vi "Results_file_Plotter.vi"() -> ()   [LabVIEW 2013]
uses:
  Anemometry/Anemometry Sub Vis/Data_plotting_vis/Plot_Slice.ctl
  Anemometry/Anemometry Sub Vis/Data_plotting_vis/Plotter_Mode.ctl
  Anemometry/Anemometry Sub Vis/Data_plotting_vis/Data_File_Type.ctl
  Anemometry/Anemometry Sub Vis/File/Setup_Filetype.ctl
  Anemometry/Anemometry Sub Vis/Controls/Global_mode.ctl
  Anemometry/Anemometry Sub Vis/Data_plotting_vis/Results_plotter_Global.vi
  Anemometry/Anemometry Sub Vis/Globals/Trav_pos_global.vi
  Instance           1 28Saved   Results_file_Plotter .vi
  Anemometry/Anemometry Sub Vis/Globals/Constants_global.vi
panel:
  out "Selected Row?":bool
  out "Edit Raw DF?":bool
  in  "Tab Control":T1(tab)=enum."Save "
  in  "Template":path
  in  "Empty":bool
  in  "Result files to read":path[](array[path])
  in  "Add results file":bool
  in  "File Types to Read":T2
  in  "Vector Plot?":bool
  in  "Ordinate Name":string
  out "2nd Add label":string
  out "First Add label":string
  in  "Additional X Values":dbl[](array[numeric]) format="%.2f"
  in  "Additional Y Values":dbl[](array[numeric]) format="%.2f"
  in  "Show Results Space Analysis":bool
  in  "Show Plot Space Analysis":bool
  in  "Multi Ordinate":i32[](listbox)
  in  "Multi Ordinate?":bool
  in  "Ordinate":u16(ring) items=["Date", "Profile", "Multi Run Start Time", "Multi Run Row Type", "Multi Run Row Number", "Point Time", "Time Stamp", "Measuring Instrument Type", "Comments", "Run Messages", "X_{HF} (mm)", "Y_{HF} (mm)", "Z_{HF} (mm)", "X_{5HP} (mm)", "Y_{5HP} (mm)", "Z_{5HP} (mm)", "Repeat", "U_{HF}/U_{ref}", "TI_{HF} %", "\\sigma_{HF}/U_{ref}", "L(U) Est (m)", "U_{5HP}/U_{ref}", "U_{HF}/U_{5HP}", "TI_{U(5HP)} %", "Vmag_{5HP}/U_{ref}", "V_{5HP}/U_{5HP}", "W_{5HP}/U_{5HP}", "U_{ref}", "U_{HF}", "Tau(HF)", "uhf^2", "uhf^3/(uhf^2)^1.5", "(uhf^4/(uhf^2)^2) -3", "HW (Uhf) Standard Error in Mean", "HW (Uhf) Standard Error in Variance", "HW Cal", "Vmag_{5HP}", "U_{5HP}", "V_{5HP}", "W_{5HP}", "Vmag_SD", "U_SD", "V_SD", "W_SD", "Tau(5HP1) (nose)", "Tau(5HP2) (bottom)", "Tau(5HP3) (top)", "Tau(5HP4) (side)", "Tau(5HP5) (side)", "GoodFraction", "5HP Mode", "5HP ReturnType", "Reference Temperature Used for Corrections", "Atmos Pressure Used for Corrections", "Av Analogue Sampling Rate", "No of Analogue Samples", "No Of Measurement Blocks", "Flow Measurement Time", "X (URef) (mm)", "Y (URef) (mm)", "Z (URef) (mm)", "Original Results Filename", "Current Data Filename", "Current Data File 1st Folder level", "Current Data File 2nd Folder level", "Current Data File 3rd Folder level", "Current Data File 4th Folder level", "Current File Number", "Raw Data Filename"]
  in  "Intensity Plot?":bool
  in  "Absisca":u16(ring) items=["Date", "Profile", "Multi Run Start Time", "Multi Run Row Type", "Multi Run Row Number", "Point Time", "Time Stamp", "Measuring Instrument Type", "Comments", "Run Messages", "X_{HF} (mm)", "Y_{HF} (mm)", "Z_{HF} (mm)", "X_{5HP} (mm)", "Y_{5HP} (mm)", "Z_{5HP} (mm)", "Repeat", "U_{HF}/U_{ref}", "TI_{HF} %", "\\sigma_{HF}/U_{ref}", "L(U) Est (m)", "U_{5HP}/U_{ref}", "U_{HF}/U_{5HP}", "TI_{U(5HP)} %", "Vmag_{5HP}/U_{ref}", "V_{5HP}/U_{5HP}", "W_{5HP}/U_{5HP}", "U_{ref}", "U_{HF}", "Tau(HF)", "uhf^2", "uhf^3/(uhf^2)^1.5", "(uhf^4/(uhf^2)^2) -3", "HW (Uhf) Standard Error in Mean", "HW (Uhf) Standard Error in Variance", "HW Cal", "Vmag_{5HP}", "U_{5HP}", "V_{5HP}", "W_{5HP}", "Vmag_SD", "U_SD", "V_SD", "W_SD", "Tau(5HP1) (nose)", "Tau(5HP2) (bottom)", "Tau(5HP3) (top)", "Tau(5HP4) (side)", "Tau(5HP5) (side)", "GoodFraction", "5HP Mode", "5HP ReturnType", "Reference Temperature Used for Corrections", "Atmos Pressure Used for Corrections", "Av Analogue Sampling Rate", "No of Analogue Samples", "No Of Measurement Blocks", "Flow Measurement Time", "X (URef) (mm)", "Y (URef) (mm)", "Z (URef) (mm)", "Original Results Filename", "Current Data Filename", "Current Data File 1st Folder level", "Current Data File 2nd Folder level", "Current Data File 3rd Folder level", "Current Data File 4th Folder level", "Current File Number", "Raw Data Filename"]
  in  "Job Directory":path
  in  "Save Averaged rows":bool
  in  "Save Surface Fit":bool
  in  "Output Filename":path
  in  "Save Data in Rows":bool
  in  "Save Plot data":bool
  in  "Header":string
  in  "Process Point":bool
  in  "Kill Point":bool
  out "Table":string[][](table)
  in  "Post Process Plotted Data":bool
  in  "...using routine":string
  in  "Calculate new metadata":bool
  in  "Add /Edit metadata":bool
  in  "Delete Plotted data from file":bool
  in  "Save Setup":bool
  in  "Load Setup":bool
  in  "stop":bool
  out "Current":string="Graph Scales"
  in  "Single Series":i32[](listbox)=[0]
  in  "Edit Template File":bool
  in  "color and symbol":bool
  out "nRows":i32
  in  "Filter Bins 2":i32[](listbox)=[0]
  in  "Filter 6":u16(ring)
  in  "Filter 5":u16(ring)
  in  "Filter 4":u16(ring) items=["Show All (160)", "BLANK (160)", "CalCheck (0)", "Zeroes (0)", "NOT BLANK (0)", "NOT CalCheck (160)", "NOT Zeroes (160)"]
  in  "Filter 3":u16(ring) items=["Show All (352)", "B2 (80)", "BLANK (0)", "C1 (160)", "C2 (112)", "NOT B2 (272)", "NOT BLANK (352)", "NOT C1 (192)", "NOT C2 (240)"]
  in  "Filter Array":u16[](array[ring])=[0, 0, 0, 0, 0, 0] items=["Don't Filter", "Date", "Profile", "Multi Run Start Time", "Multi Run Row Type", "Multi Run Row Number", "Point Time", "Time Stamp", "Measuring Instrument Type", "Comments", "Run Messages", "X_{HF} (mm)", "Y_{HF} (mm)", "Z_{HF} (mm)", "X_{5HP} (mm)", "Y_{5HP} (mm)", "Z_{5HP} (mm)", "Repeat", "U_{HF}/U_{ref}", "TI_{HF} %", "\\sigma_{HF}/U_{ref}", "L(U) Est (m)", "U_{5HP}/U_{ref}", "U_{HF}/U_{5HP}", "TI_{U(5HP)} %", "Vmag_{5HP}/U_{ref}", "V_{5HP}/U_{5HP}", "W_{5HP}/U_{5HP}", "U_{ref}", "U_{HF}", "Tau(HF)", "uhf^2", "uhf^3/(uhf^2)^1.5", "(uhf^4/(uhf^2)^2) -3", "HW (Uhf) Standard Error in Mean", "HW (Uhf) Standard Error in Variance", "HW Cal", "Vmag_{5HP}", "U_{5HP}", "V_{5HP}", "W_{5HP}", "Vmag_SD", "U_SD", "V_SD", "W_SD", "Tau(5HP1) (nose)", "Tau(5HP2) (bottom)", "Tau(5HP3) (top)", "Tau(5HP4) (side)", "Tau(5HP5) (side)", "GoodFraction", "5HP Mode", "5HP ReturnType", "Reference Temperature Used for Corrections", "Atmos Pressure Used for Corrections", "Av Analogue Sampling Rate", "No of Analogue Samples", "No Of Measurement Blocks", "Flow Measurement Time", "X (URef) (mm)", "Y (URef) (mm)", "Z (URef) (mm)", "Original Results Filename", "Current Data Filename", "Current Data File 1st Folder level", "Current Data File 2nd Folder level", "Current Data File 3rd Folder level", "Current Data File 4th Folder level", "Current File Number", "Raw Data Filename"]
  in  "Filter Bins 1":i32[](listbox)=[0]
  in  "Create picture Vi Name":string caption="Picture VI:"
  in  "Save Plot as jpg":bool
  in  "Reload Files":bool
  out "Selected Row":i32
  out "Warning!":string
  out "XY Plot":cluster{dbl[], dbl[]}[](graph)
  out "Edit Raw Data Header Info":bool
  out "Raw DF in Orig Pos?":bool
  out "Intensity Graph":dbl[][](graph)
  in  "Bkgnd Value":dbl
  in  "Update":bool
  in  "Plot Resolution":bool
  in  "Point Size":i32(slide)=1 scale=0.0..10.0
  in  "No of Contours":i32=20
  in  "Slice mode":T3
  in  "Z Ch Name":u16(ring) items=["Date", "Profile", "Multi Run Start Time", "Multi Run Row Type", "Multi Run Row Number", "Point Time", "Time Stamp", "Measuring Instrument Type", "Comments", "Run Messages", "X_{HF} (mm)", "Y_{HF} (mm)", "Z_{HF} (mm)", "X_{5HP} (mm)", "Y_{5HP} (mm)", "Z_{5HP} (mm)", "Repeat", "U_{HF}/U_{ref}", "TI_{HF} %", "\\sigma_{HF}/U_{ref}", "L(U) Est (m)", "U_{5HP}/U_{ref}", "U_{HF}/U_{5HP}", "TI_{U(5HP)} %", "Vmag_{5HP}/U_{ref}", "V_{5HP}/U_{5HP}", "W_{5HP}/U_{5HP}", "U_{ref}", "U_{HF}", "Tau(HF)", "uhf^2", "uhf^3/(uhf^2)^1.5", "(uhf^4/(uhf^2)^2) -3", "HW (Uhf) Standard Error in Mean", "HW (Uhf) Standard Error in Variance", "HW Cal", "Vmag_{5HP}", "U_{5HP}", "V_{5HP}", "W_{5HP}", "Vmag_SD", "U_SD", "V_SD", "W_SD", "Tau(5HP1) (nose)", "Tau(5HP2) (bottom)", "Tau(5HP3) (top)", "Tau(5HP4) (side)", "Tau(5HP5) (side)", "GoodFraction", "5HP Mode", "5HP ReturnType", "Reference Temperature Used for Corrections", "Atmos Pressure Used for Corrections", "Av Analogue Sampling Rate", "No of Analogue Samples", "No Of Measurement Blocks", "Flow Measurement Time", "X (URef) (mm)", "Y (URef) (mm)", "Z (URef) (mm)", "Original Results Filename", "Current Data Filename", "Current Data File 1st Folder level", "Current Data File 2nd Folder level", "Current Data File 3rd Folder level", "Current Data File 4th Folder level", "Current File Number", "Raw Data Filename"]
  in  "Y Ch Name":u16(ring) items=["Date", "Profile", "Multi Run Start Time", "Multi Run Row Type", "Multi Run Row Number", "Point Time", "Time Stamp", "Measuring Instrument Type", "Comments", "Run Messages", "X_{HF} (mm)", "Y_{HF} (mm)", "Z_{HF} (mm)", "X_{5HP} (mm)", "Y_{5HP} (mm)", "Z_{5HP} (mm)", "Repeat", "U_{HF}/U_{ref}", "TI_{HF} %", "\\sigma_{HF}/U_{ref}", "L(U) Est (m)", "U_{5HP}/U_{ref}", "U_{HF}/U_{5HP}", "TI_{U(5HP)} %", "Vmag_{5HP}/U_{ref}", "V_{5HP}/U_{5HP}", "W_{5HP}/U_{5HP}", "U_{ref}", "U_{HF}", "Tau(HF)", "uhf^2", "uhf^3/(uhf^2)^1.5", "(uhf^4/(uhf^2)^2) -3", "HW (Uhf) Standard Error in Mean", "HW (Uhf) Standard Error in Variance", "HW Cal", "Vmag_{5HP}", "U_{5HP}", "V_{5HP}", "W_{5HP}", "Vmag_SD", "U_SD", "V_SD", "W_SD", "Tau(5HP1) (nose)", "Tau(5HP2) (bottom)", "Tau(5HP3) (top)", "Tau(5HP4) (side)", "Tau(5HP5) (side)", "GoodFraction", "5HP Mode", "5HP ReturnType", "Reference Temperature Used for Corrections", "Atmos Pressure Used for Corrections", "Av Analogue Sampling Rate", "No of Analogue Samples", "No Of Measurement Blocks", "Flow Measurement Time", "X (URef) (mm)", "Y (URef) (mm)", "Z (URef) (mm)", "Original Results Filename", "Current Data Filename", "Current Data File 1st Folder level", "Current Data File 2nd Folder level", "Current Data File 3rd Folder level", "Current Data File 4th Folder level", "Current File Number", "Raw Data Filename"]
  in  "X Ch Name":u16(ring) items=["Date", "Profile", "Multi Run Start Time", "Multi Run Row Type", "Multi Run Row Number", "Point Time", "Time Stamp", "Measuring Instrument Type", "Comments", "Run Messages", "X_{HF} (mm)", "Y_{HF} (mm)", "Z_{HF} (mm)", "X_{5HP} (mm)", "Y_{5HP} (mm)", "Z_{5HP} (mm)", "Repeat", "U_{HF}/U_{ref}", "TI_{HF} %", "\\sigma_{HF}/U_{ref}", "L(U) Est (m)", "U_{5HP}/U_{ref}", "U_{HF}/U_{5HP}", "TI_{U(5HP)} %", "Vmag_{5HP}/U_{ref}", "V_{5HP}/U_{5HP}", "W_{5HP}/U_{5HP}", "U_{ref}", "U_{HF}", "Tau(HF)", "uhf^2", "uhf^3/(uhf^2)^1.5", "(uhf^4/(uhf^2)^2) -3", "HW (Uhf) Standard Error in Mean", "HW (Uhf) Standard Error in Variance", "HW Cal", "Vmag_{5HP}", "U_{5HP}", "V_{5HP}", "W_{5HP}", "Vmag_SD", "U_SD", "V_SD", "W_SD", "Tau(5HP1) (nose)", "Tau(5HP2) (bottom)", "Tau(5HP3) (top)", "Tau(5HP4) (side)", "Tau(5HP5) (side)", "GoodFraction", "5HP Mode", "5HP ReturnType", "Reference Temperature Used for Corrections", "Atmos Pressure Used for Corrections", "Av Analogue Sampling Rate", "No of Analogue Samples", "No Of Measurement Blocks", "Flow Measurement Time", "X (URef) (mm)", "Y (URef) (mm)", "Z (URef) (mm)", "Original Results Filename", "Current Data Filename", "Current Data File 1st Folder level", "Current Data File 2nd Folder level", "Current Data File 3rd Folder level", "Current Data File 4th Folder level", "Current File Number", "Raw Data Filename"]
  in  "Resolution":dbl=1.0 min=0.0 format="%.4f"
  out "Surface Area":dbl format="%^_6g"
  out "Surface Integral":dbl format="%^_6g"
  out "Surface Average":dbl format="%^#.6g"
  out "Uadvec":dbl
  in  "Full_Res_Results_Folder":path
  out "Last used Template":path
  out "Cursor index":i32
  out "Choosen Path":path
  in  "VI Refnum Calculation":refnum<vi>
  out "Filetype":string[](array[string])
  out "Mode":T4
  out "Plotted rows only?":bool
  in  "type specifier VI Refnum (for type only) 2":refnum<vi>
  in  "type specifier VI Refnum (for type only)":refnum<vi>
  out "Accept Array":bool[][](array[boolean])
  out "Previous slice mode":T3
  out "Slice mode Change?":bool
  out "Non-Blank Rows":bool[](array[boolean])
  out "File Index":i32
  out "Tolerances":dbl[](array[numeric]) format="%.2f"
  in  "Results files choosen":path[](array[path])
  in  "Transpose":bool
  out "Plotted Series":bool[][](array[boolean])
  in  "Results file":path
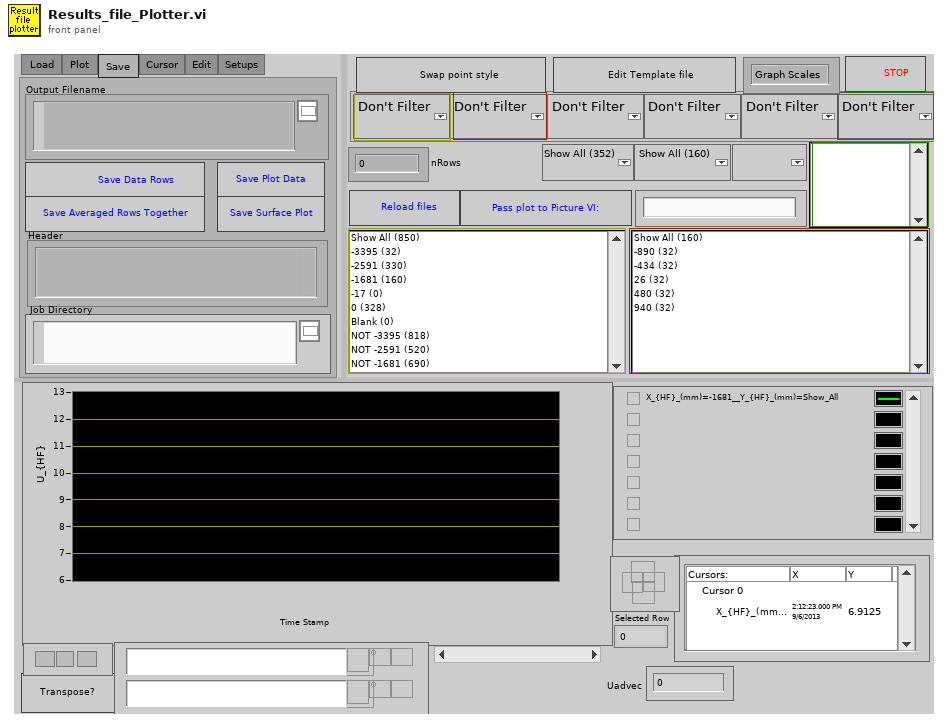
[diagram p1: front panel]
types:
  T1 = enum32{"Load ", "Plot ", "Save ", "Cursor", "Edit", "Setups"}
  T2 = typedef "Data_File_Type.ctl" = enum16{"Read All File Types", "Results Files Only", "Raw Data Files Only", "Calibration Files Only", "Gas Desk Files Only", "Old Results Files Only", "Tabulated Data Files Only"}
  T3 = typedef "Plot_Slice.ctl" = enum16{"XY Slice (Plan)", "YX Slice (Plan)", "YZ Slice (Cross)", "ZY Slice (Cross)", "XZ Slice (Side)", "ZX Slice (Side)"}
  T4 = typedef "Plotter_Mode.ctl" = enum16{"Save file", "Delete unwanted rows", "Edit Values with constants", "Edit values per row", "Edit Raw Data file header", "Post Process Plotted Rows"}
  T5 = typedef "Setup_Filetype.ctl" = enum16{"Measurement Setups", "Calibration Setups", "General", "Results File Plotter Setups", "Speed Calib Tweaks"}
  T6 = enum16{"Zero or one", "One", "Zero or more", "One or more"}
  T7 = typedef "Global_mode.ctl" = enum16{"Read Global", "Load Global From File", "Write Global to File"}
  T8 = enum16{"Edit Existing Template File", "Create New Template File"}
  T9 = enum16{"Show only data summary", "Show data summary", "No data summary"}
  T10 = typedef "All_Setup.ctl" = cluster{"Result files to read":path[], "Template":path, "Transpose":bool, "Additional X Values":dbl[], "Additional Y Values":dbl[], "Ordinate":u16, "Absisca":u16, "Filter Array":u16[], "color and symbol":bool, "Output Filename":path, "Jpg Vi Name":string, "Intensity Plot?":bool, "Multi Ordinate?":bool, "Filter Bins 1":i32[], "Filter Bins 2":i32[], "Multi Ordinate":i32[]}
  T11 = enum16{"Left Button", "Center Button", "Right Button", "Window Close"}
  T12 = enum32{"existing file", "new file", "new or existing file", "existing dir", "new dir", "new or existing dir", "existing file (use LLBs)", "new file (use LLBs)", "new or existing file (use LLBs)", "new or existing file or directory (use LLBs)"}
  T13 = cluster{"Plot Color":u32, "Plot Interpolation":u8, "Point Style":u8, "Line Style":u8, "Fill/Pt. Color":u32, "Line Width":u8, "Bar Plot Style":u8, "Fill To":i16}[]
  T14 = typedef "Group_Binning.ctl" = cluster{"Index":i32, "Tolerance":dbl, "Precision":string}
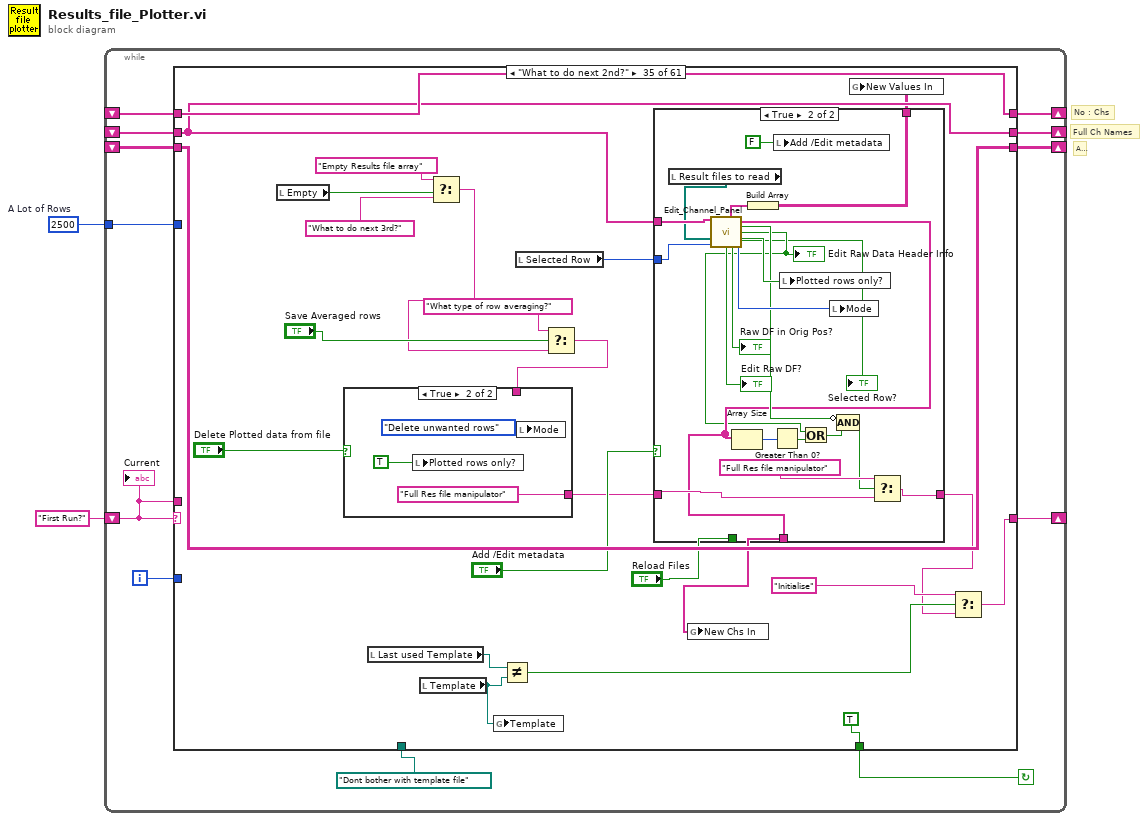
[diagram p0: block diagram]
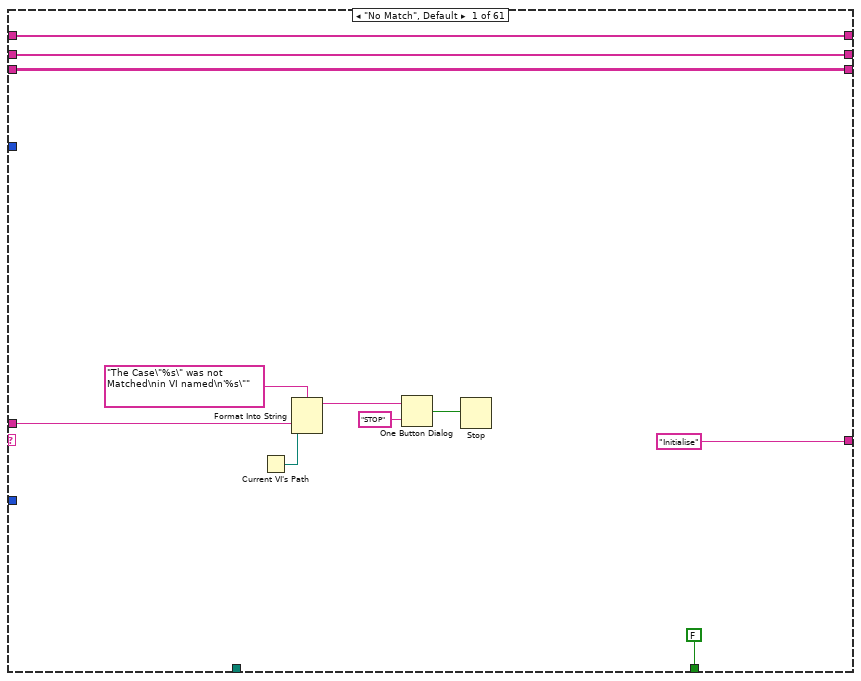
[diagram p2: hidden frame]
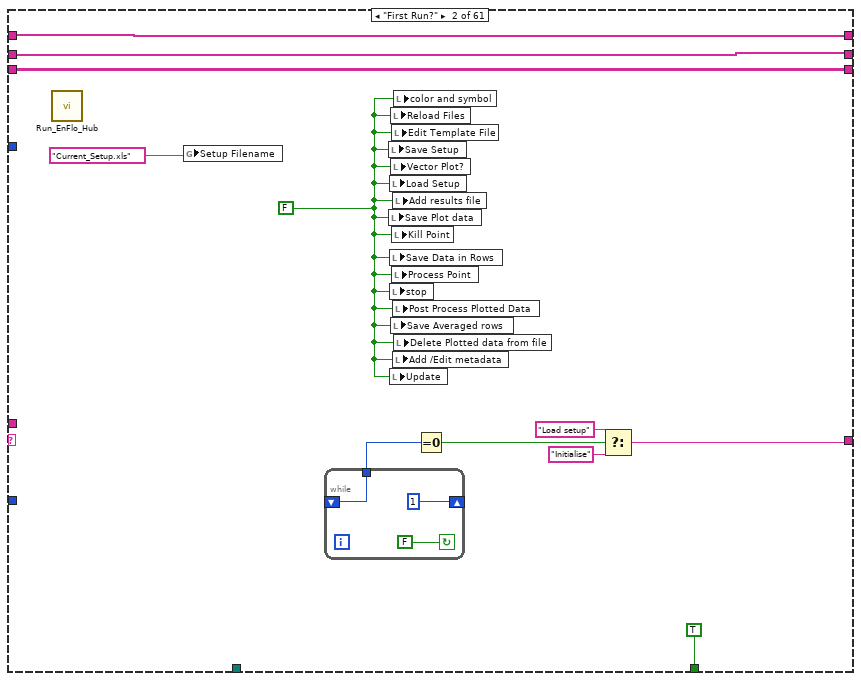
[diagram p3: hidden frame]
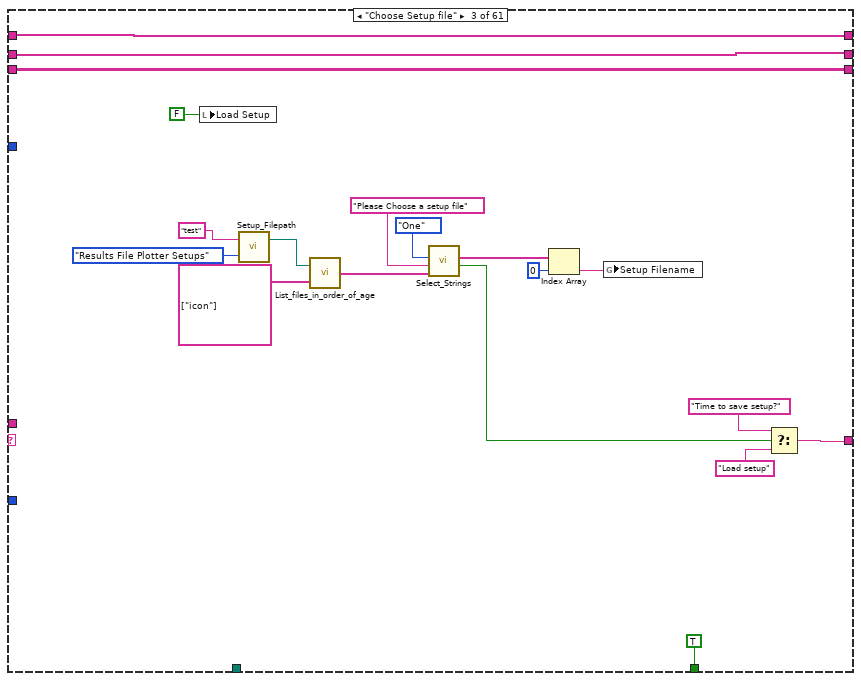
[diagram p4: hidden frame]
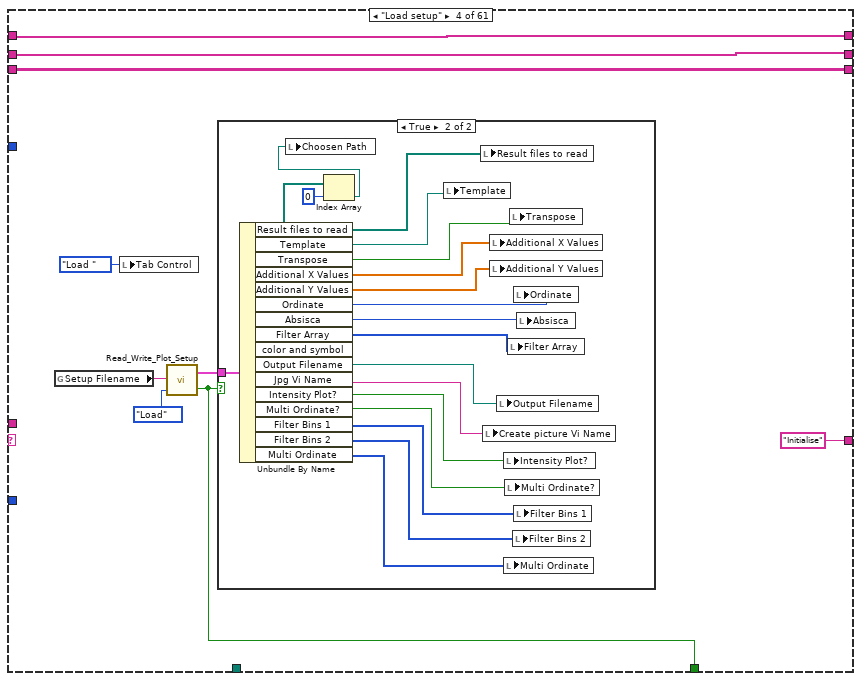
[diagram p5: hidden frame]
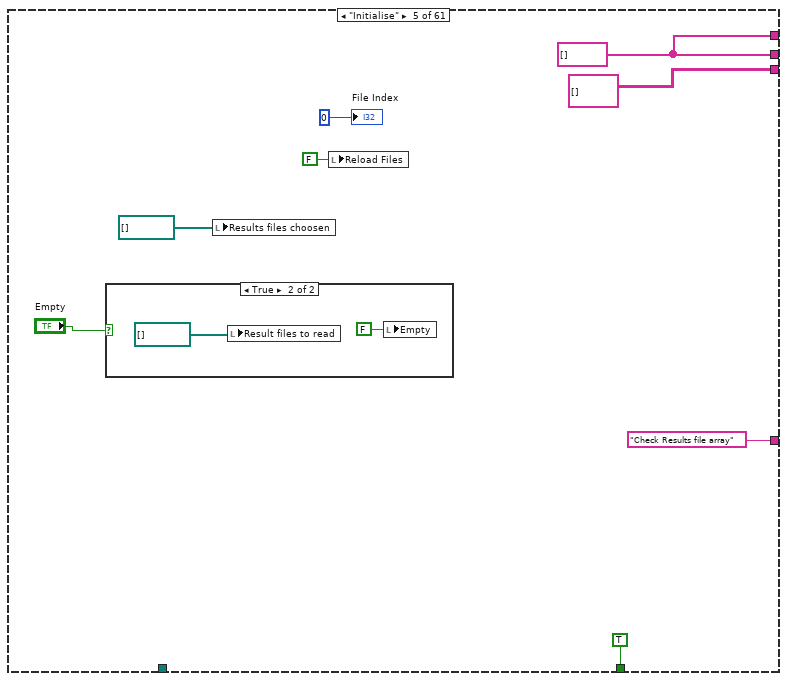
[diagram p7: hidden frame]
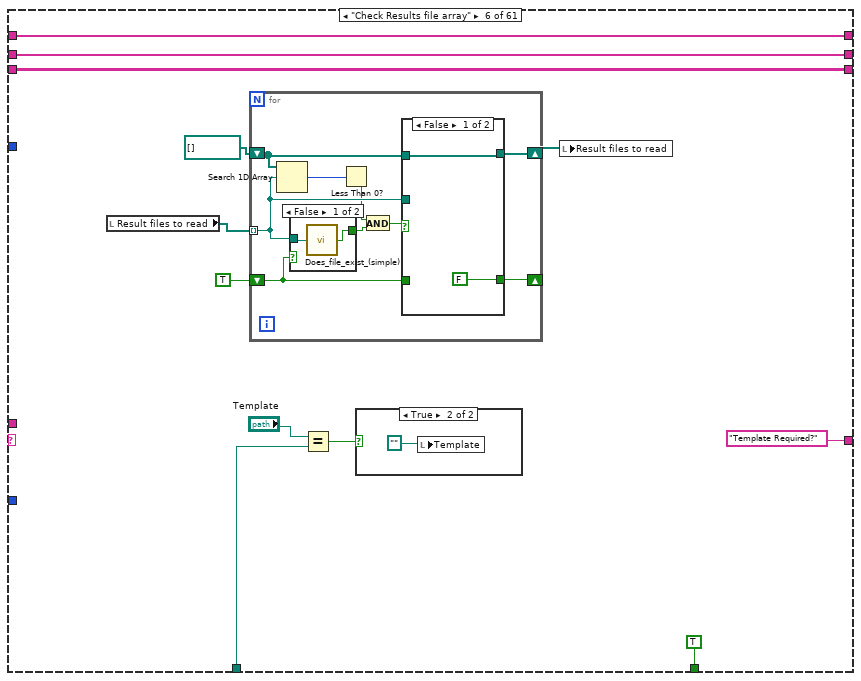
[diagram p9: hidden frame]
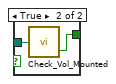
[diagram p11: hidden frame]
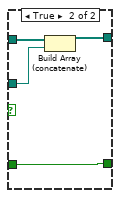
[diagram p12: hidden frame]
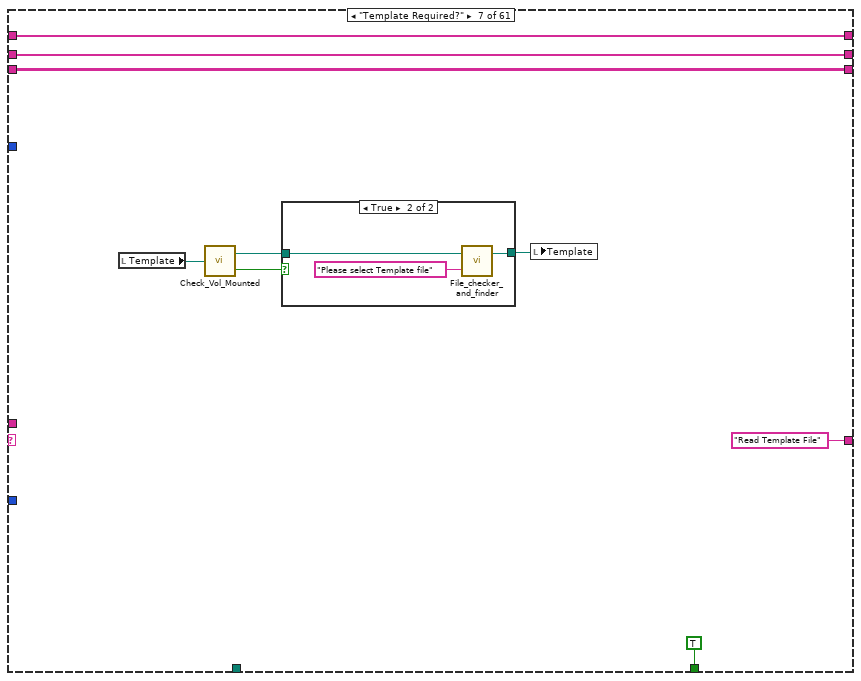
[diagram p13: hidden frame]
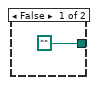
[diagram p14: hidden frame]
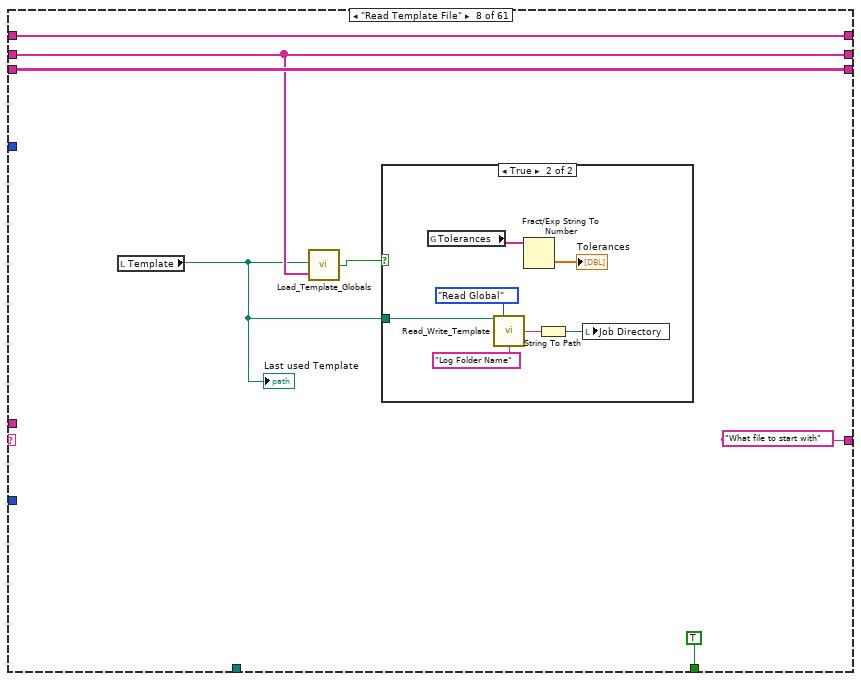
[diagram p15: hidden frame]
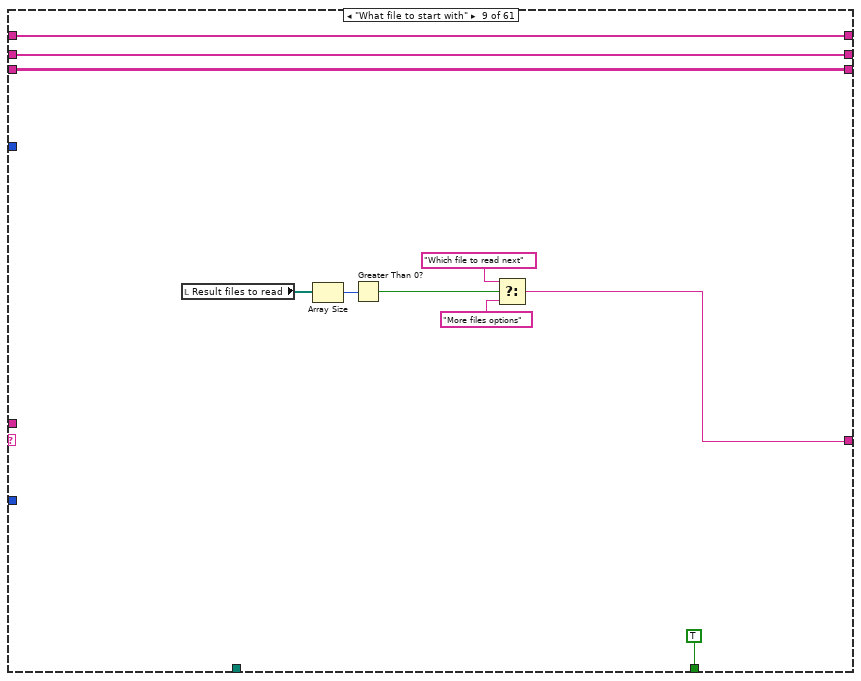
[diagram p17: hidden frame]
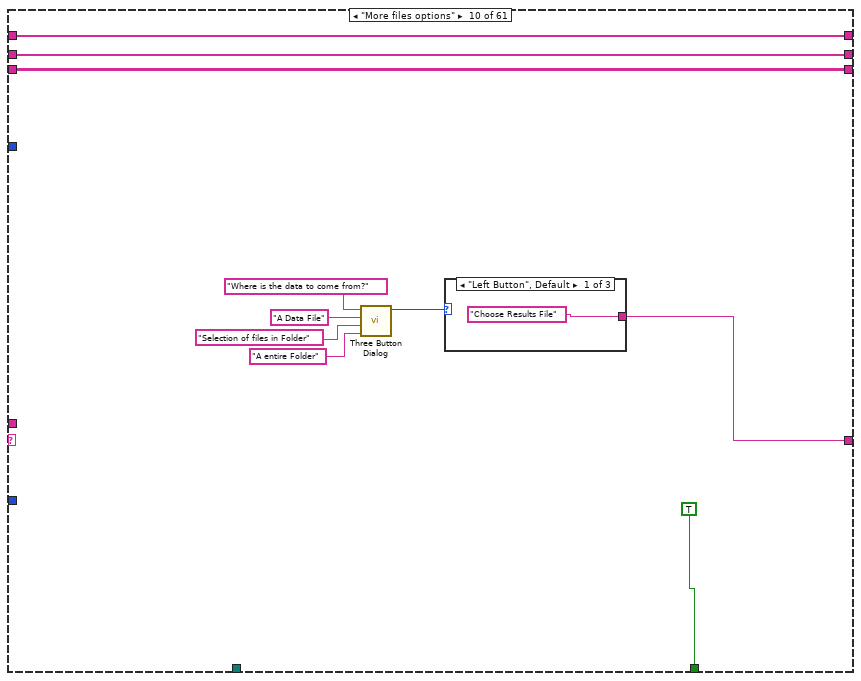
[diagram p18: hidden frame]
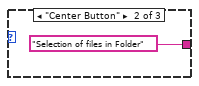
[diagram p19: hidden frame]
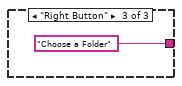
[diagram p20: hidden frame]
diagram:
  w1 = 2500  # A Lot of Rows
  # "No : Chs"
  # "Full Ch Names"
  # "All"
  n1 = while {
    shift-left: _ -> [w7]
    shift-right: [w8] -> _
    shift-left: "First Run?" -> [w11]
    shift-right: [w4] -> _
    shift-left: _ -> [w9]
    shift-right: [w14] -> _
    shift-left: _ -> [w12]
    shift-right: [w5] -> _
    tunnel: w1 -> [w3]
    i -> [w6]
    stop <- w13 continue-if-true
    n2 = case shown="\"What to do next 2nd?\"" w11 {
      tunnel: w9 -> [w25 w35 w57 w65 _ w106 w134 w143 w164 w174 w186 w200 w231 w258 w281 w403 w425 w451 w476 w502 w556 w570 w607 w909 w978 w1033 w1058 w1077 w1163 w1214 w1244 w1533 w1549 w1570 w1600 w1666 w1699 w1774 w1797 w1812 w1876 w1928 w1954 w2163 w2175 w2201 w2327 w2471 w2505 w2520 w2545 w2572 w2615 w2633 w2676 w2779 w2813 w3177 w3192 w3228 w3236]
      tunnel: [w25 w35 w57 w65 w91 w106 w134 w143 w164 w174 w186 w200 w231 w258 w279 w403 w425 w451 w476 w502 w556 w570 w607 w909 w978 w1033 w1058 w1077 w1163 w1214 w1242 w1533 w1549 w1570 w1600 w1666 w1699 w1774 w1797 w1812 w1876 w1928 w1952 w2163 w2175 w2199 w2320 w2471 w2505 w2520 w2545 w2572 w2615 w2633 w2676 w2779 w2813 w3177 w3192 w3228 w3236] -> w14
      tunnel: ["Initialise" w28 w52 "Initialise" ("t") "Check Results file array" ("t") "Template Required?" "Read Template File" "What file to start with" w155 w170 "Which file to read next" "Which file to read next" "Which file to read next" w254 w276 w394 "What is present?" "Ordinate Selector Type" w473 "Which rows are Non-Blank?" w549 "Create Selectors" w596 "Re Plot Data?" w973 "Prepare Filter2 strings" "Plot Data" w1074 "Add Axis names" "Analyse Plot Space" w1245 "What to do next?" "What to do next?" ("t") w1556 w1593 w1644 w1697 w1768 w1793 w1811 w1875 "Initialise" w1955 w2154 "Create Selectors" w2202 w2328 w2469 w2503 w2510 w2529 "Save XY plot as jpg" "Create Selectors" w2630 w2679 w2763 w2818 "Save Setup" ("t") "Initialise" ("t") w3197 "Time to save setup?"] -> w4
      tunnel: [FALSE TRUE TRUE w61 TRUE TRUE TRUE TRUE TRUE TRUE TRUE TRUE TRUE w249 w283 TRUE TRUE TRUE TRUE TRUE TRUE TRUE TRUE TRUE TRUE TRUE TRUE w1075 TRUE TRUE w1246 TRUE TRUE ("OK?") TRUE TRUE ("OK?") TRUE ("OK?") w1695 TRUE TRUE w1810 w1874 TRUE w1956 TRUE ("OK?") TRUE ("OK?") w2203 w2329 TRUE TRUE TRUE TRUE TRUE TRUE TRUE TRUE TRUE TRUE TRUE TRUE w3206 TRUE ("OK?")] -> w13
      tunnel: w12 -> [w24 w34 w56 w64 _ w105 w133 w145 w163 w173 w185 w199 w230 w257 w282 w399 w424 w452 w477 w503 w555 w568 w602 w911 w967 w1035 w1060 w1076 w1165 w1216 w1243 w1532 w1548 w1569 w1611 w1665 w1698 w1773 w1796 w1809 w1873 w1927 w1953 w2162 w2172 w2200 w2326 w2472 w2504 w2519 w2549 w2575 w2614 w2632 w2675 w2778 w2812 w3176 w3191 w3227 w3235]
      tunnel: w11 -> [w16 _ _ _ _ _ _ _ _ _ _ _ _ _ _ _ _ _ _ _ _ _ _ _ _ _ _ _ _ _ _ _ _ _ _ _ _ _ _ _ _ _ _ _ _ _ _ _ _ _ _ _ _ _ _ _ _ _ _ _ _]
      tunnel: path "Dont bother with template file" ("Template File") -> [_ _ _ _ _ w99 _ _ _ _ _ _ _ _ _ _ _ _ _ _ _ _ _ _ _ _ _ _ _ _ _ _ _ _ _ _ _ _ _ _ _ _ _ _ _ _ _ _ _ _ _ _ _ _ _ _ _ w3174 w3186 _ _]
      tunnel: [w15 w33 w55 w66 w91 w104 w132 w144 w161 w171 w183 w197 w228 w256 w278 w387 w423 w453 w475 w501 w547 w569 w600 w908 w969 w1026 w1053 w1073 w1157 w1209 w1238 w1529 w1550 w1568 w1601 w1667 w1700 w1772 w1795 w1808 w1872 w1926 w1946 w2164 w2180 w2190 w2323 w2481 w2506 w2521 w2546 w2573 w2616 w2634 w2680 w2780 w2819 w3178 w3193 w3229 w3237] -> w8
      tunnel: w7 -> [w15 w33 w55 w66 _ w104 w132 w144 w161 w171 w183 w197 w228 w256 w277 w387 w423 w453 w475 w501 w547 w569 w600 w908 w969 w1026 w1053 w1073 w1157 w1209 w1237 w1529 w1550 w1568 w1601 w1667 w1700 w1772 w1795 w1808 w1872 w1926 w1945 w2164 w2180 w2194 w2322 w2481 w2506 w2521 w2546 w2573 w2616 w2634 w2680 w2780 w2819 w3178 w3193 w3229 w3237]
      tunnel: w6 -> [_ _ _ _ _ _ _ _ _ _ _ _ _ _ _ _ _ _ _ _ _ _ _ _ _ _ _ _ _ _ _ _ _ _ _ _ w1696 _ _ _ _ _ _ _ _ _ _ _ _ _ _ _ _ _ _ _ _ _ _ _ _]
      tunnel: [w24 w34 w56 w64 string[][] [] w105 w133 w145 w163 w173 w185 w199 w230 w257 w280 w399 w424 w452 w477 w503 w555 w568 w602 w911 w967 w1035 w1060 w1076 w1165 w1216 w1241 w1532 w1548 w1569 w1611 w1665 w1698 w1773 w1796 w1809 w1873 w1927 w1951 w2162 w2172 w2198 w2319 w2472 w2504 w2519 w2549 w2575 w2614 w2632 w2675 w2778 w2812 w3176 w3191 w3227 w3235] -> w5
      tunnel: w3 -> [_ _ _ _ _ _ _ _ _ _ _ _ _ _ _ _ _ _ _ _ _ _ _ _ _ _ _ _ _ _ _ _ _ _ _ _ _ _ w1791 _ w1871 _ _ _ _ _ _ _ _ _ _ _ _ w2629 w2673 _ w2810 _ _ _ _]
      frame "No Match", Default {
        n3 = Current VI's Path() -> (path=w17:path)
        n4 = Format Into String(format string="The Case\"%s\" was not Matched\nin VI named\n'%s\"" ("Format String"), w16, w17) -> (resulting string=w20:string)  [unwired: 2 in, 1 out]
        n5 = One Button Dialog(message=w20, button name ("OK")="STOP") -> (true=w18:bool)
        n6 = Stop(stop? (T)=w18) -> ()
      }
      frame "First Run?" {
        w26 = FALSE ("Save Plot data")
        n7 = call "Run_EnFlo_Hub.vi"() -> ()  [unwired: 8 out]
        n8 = global write "Results_plotter_Global.vi" "Setup Filename"("Current_Setup.xls" ("Setup filename")) -> ()
        n9 = while {
          shift-right: [1] -> _
          shift-left: _ -> [w38]
          tunnel: [w38] -> w30
          stop <- FALSE continue-if-true
        }
        n10 = local write "Save Setup"(w26) -> ()
        n11 = local write "Save Plot data"(w26) -> ()
        n12 = local write "Load Setup"(w26) -> ()
        n13 = local write "Save Data in Rows"(w26) -> ()
        n14 = local write "stop"(w26) -> ()
        n15 = local write "Update"(w26) -> ()
        n16 = local write "Reload Files"(w26) -> ()
        n17 = local write "Vector Plot?"(w26) -> ()
        n18 = local write "Save Averaged rows"(w26) -> ()
        n19 = local write "Edit Template File"(w26) -> ()
        n20 = local write "Kill Point"(w26) -> ()
        n21 = local write "Process Point"(w26) -> ()
        n22 = local write "Add results file"(w26) -> ()
        n23 = local write "Post Process Plotted Data"(w26) -> ()
        n24 = local write "Add /Edit metadata"(w26) -> ()
        n25 = local write "color and symbol"(w26) -> ()
        n26 = local write "Delete Plotted data from file"(w26) -> ()
        n27 = Equal To 0?(x=w30) -> (x = 0?=w29:bool)
        n28 = Select(t="Load setup", s=w29, f="Initialise") -> (s? t:f=w28:string)
      }
      frame "Choose Setup file" {
        n29 = local write "Load Setup"(FALSE ("Save Setup")) -> ()
        n30 = call "Setup_Filepath.vi"("Setup File Type"=Setup_Filetype."Results File Plotter Setups", "Filename in"="test") -> ("Directory"=w40:path)  [unwired: 1 out]
        n31 = call "List_files_in_order_of_age.vi"("Files to Hide"=string[] ["icon"], "Folder"=w40) -> ("file names"=w51:string[])
        n32 = call "Select_Strings.vi"("Available Ch names"=w51, "Message"="Please Choose a setup file", "Selector mode"=T6."One") -> ("Cancel"=w45:bool, "Selected Channel Names"=w48:string[])  [unwired: 1 in, 3 out]
        n33 = Index Array(array=w48, index=0) -> (element=w46:string)
        n34 = global write "Results_plotter_Global.vi" "Setup Filename"(w46) -> ()
        n35 = Select(t="Time to save setup?", s=w45, f="Load setup") -> (s? t:f=w52:string)
      }
      frame "Load setup" {
        n36 = global read "Results_plotter_Global.vi" "Setup Filename"() -> (w60:string)
        n37 = local write "Tab Control"(T1."Load " ("Tab Control")) -> ()
        n38 = call "Read_Write_Plot_Setup.vi"("Mode"=enum16{"Load", "Save"}."Load", "Setup filename"=w60) -> ("OK?"=w61:bool, "Cluster 2"=w62:T10)  [unwired: 1 in]
        n39 = case shown="True" w61 {
          tunnel: w62 -> [_ w85]
          frame False {
          }
          frame True {
            n40 = Unbundle By Name(w85) -> ("Result files to read"=w70:path[], "Template"=w68:path, "Transpose"=w75:bool, "Additional X Values"=w76:dbl[], "Additional Y Values"=w77:dbl[], "Ordinate"=w78:u16, "Absisca"=w79:u16, "Filter Array"=w80:u16[], "Output Filename"=w81:path, "Jpg Vi Name"=w82:string, "Intensity Plot?"=w83:bool, "Multi Ordinate?"=w84:bool, "Filter Bins 1"=w74:i32[], "Filter Bins 2"=w73:i32[], "Multi Ordinate"=w72:i32[])  [unwired: 1 out]
            n41 = Index Array(array=w70, index=0) -> (element=w69:path)
            n42 = local write "Choosen Path"(w69) -> ()
            n43 = local write "Template"(w68) -> ()
            n44 = local write "Result files to read"(w70) -> ()
            n45 = local write "Create picture Vi Name"(w82) -> ()
            n46 = local write "Additional X Values"(w76) -> ()
            n47 = local write "Additional Y Values"(w77) -> ()
            n48 = local write "Output Filename"(w81) -> ()
            n49 = local write "Intensity Plot?"(w83) -> ()
            n50 = local write "Multi Ordinate"(w72) -> ()
            n51 = local write "Multi Ordinate?"(w84) -> ()
            n52 = local write "Filter Array"(w80) -> ()
            n53 = local write "Transpose"(w75) -> ()
            n54 = local write "Filter Bins 2"(w73) -> ()
            n55 = local write "Ordinate"(w78) -> ()
            n56 = local write "Filter Bins 1"(w74) -> ()
            n57 = local write "Absisca"(w79) -> ()
          }
        }
      }
      frame "Initialise" {
        w91 = string[] [] ("Channel names")
        n58 = case shown="True" "Empty" {
          frame False {
          }
          frame True {
            n59 = local write "Result files to read"(path[] [] ("Result files to read")) -> ()
            n60 = local write "Empty"(FALSE ("Empty")) -> ()
          }
        }
        n61 = local write "Results files choosen"(path[] [] ("Results file choosen")) -> ()
        n62 = local write "Reload Files"(FALSE ("Reload Files")) -> ()
        "File Index" <- 0
      }
      frame "Check Results file array" {
        n63 = local read "Result files to read"() -> (w103:path[])
        n64 = for {
          shift-right: [w117] -> w101
          shift-left: path[] [] -> [w116]
          tunnel: w103 -> [w115] mode=indexing
          shift-right: [w110] -> _
          shift-left: TRUE -> [w109]
          n65 = Search 1D Array(1D array=w116, element=w115) -> (index of element=w114:i32)  [unwired: 1 out]
          n66 = case shown="False" w109 {
            tunnel: w115 -> [w119 w121]
            tunnel: [w118 w120] -> w112
            frame False {
              n67 = call "Does_file_exist_(simple).vi"("Pathname"=w119) -> ("exists?"=w118:bool)
            }
            frame True {
              n68 = call "Check_Vol_Mounted.vi"("Filename"=w121) -> ("exists?"=w120:bool)  [unwired: 1 out]
            }
          }
          n69 = Less Than 0?(x=w114) -> (x < 0?=w111:bool)
          n70 = And(x=w111, y=w112) -> (x .and. y?=w113:bool)
          n71 = case shown="False" w113 {
            tunnel: w116 -> [w123 w127]
            tunnel: w115 -> [_ w126]
            tunnel: [w123 w125] -> w117
            tunnel: [FALSE w124] -> w110
            tunnel: w109 -> [_ w124]
            frame False {
            }
            frame True {
              n72 = Build Array (concatenate)(w127, w126) -> (w125:path[])
            }
          }
        }
        n73 = Equal?(x="Template", y=w99) -> (x = y?=w98:bool)
        n74 = case shown="True" w98 {
          frame False {
          }
          frame True {
            n75 = local write "Template"(path "") -> ()
          }
        }
        n76 = local write "Result files to read"(w101) -> ()
      }
      frame "Template Required?" {
        n77 = local read "Template"() -> (w131:path)
        n78 = call "Check_Vol_Mounted.vi"("Filename"=w131) -> ("Filename Out"=w130:path, "exists?"=w129:bool)
        n79 = case shown="True" w129 {
          tunnel: w130 -> [_ w139]
          tunnel: [path "" w138] -> w128
          frame False {
          }
          frame True {
            n80 = call "File_checker_and_finder.vi"("Promp if not found"="Please select Template file", "Filename In"=w139) -> ("Filename Out"=w138:path)  [unwired: 1 out]
          }
        }
        n81 = local write "Template"(w128) -> ()
      }
      frame "Read Template File" {
        n82 = local read "Template"() -> (w141:path)
        "Last used Template" <- w141
        n83 = call "Load_Template_Globals.vi"("Channel Names"=w143, "Template-read"=w141) -> ("Valid Template File?"=w142:bool)
        n84 = case shown="True" w142 {
          tunnel: w141 -> [_ w149]
          frame False {
          }
          frame True {
            n85 = global read "Results_plotter_Global.vi" "Tolerances"() -> (w153:string[])
            n86 = call "Read_Write_Template.vi"("Template File"=w149, "Mode"=Global_mode."Read Global", "Data type"="Log Folder Name" ("Variable name")) -> ("Single Value Out"=w151:string)  [unwired: 5 in, 7 out]
            n87 = Fract/Exp String To Number(string=w153) -> (number=→"Tolerances":dbl[])  [unwired: 4 out]
            n88 = String To Path(string=w151) -> (path=w148:path)
            n89 = local write "Job Directory"(w148) -> ()
          }
        }
      }
      frame "What file to start with" {
        n90 = local read "Result files to read"() -> (w160:path[])
        n91 = Array Size(array=w160) -> (size(s)=w159:i32)
        n92 = Greater Than 0?(x=w159) -> (x > 0?=w156:bool)
        n93 = Select(t="Which file to read next", s=w156, f="More files options") -> (s? t:f=w155:string)
      }
      frame "More files options" {
        n94 = call <vilib>:"Three Button Dialog.vi"("Right Button Text (\"Cancel\")"="A entire Folder" ("F button name (\"Cancel\")"), "Center Button Text (\"No\")"="Selection of files in Folder" ("T button name (\"OK\")"), "Left Button Text (\"Yes\")"="A Data File" ("T button name (\"OK\")"), "message"="Where is the data to come from?") -> ("Which Button?"=w169:T11)  [unwired: 1 in, 6 out]
        n95 = case shown="\"Left Button\", Default" w169 {
          tunnel: ["Choose Results File" "Selection of files in Folder" "Choose a Folder"] -> w170
          frame "Left Button", Default {
          }
          frame "Center Button" {
          }
          frame "Right Button" {
          }
        }
      }
      frame "Choose Results File" {
        (unwired) T12."existing file" ("select mode (2)")
        n96 = local read "Choosen Path"() -> (w178:path)
        n97 = File Dialog(7:"Please Choose a Results File" ("Promp if not found"), 11:w178) -> (1:w180:bool, 3:w179:path)  [unwired: 1 in, 6 out]
        "Choosen Path" <- w179
        n98 = case shown="False" w180 {
          tunnel: w179 -> [w187 _]
          frame False {
            n99 = local read "Result files to read"() -> (w188:path[])
            n100 = Build Array (concatenate)(w188, w187) -> (w189:path[])
            n101 = local write "Result files to read"(w189) -> ()
          }
          frame True {
          }
        }
      }
      frame "Choose a Folder" {
        n102 = local read "Choosen Path"() -> (w191:path)
        n103 = File Dialog(7:"Please Choose the folder that contains the Results files to be plotted" ("prompt"), 11:w191) -> (3:w190:path)  [unwired: 1 in, 7 out]
        n104 = local write "Choosen Path"(w190) -> ()
        n105 = call "Get_folder_and_filenames.vi"("file path (dialog if empty)"=w190) -> ("Files"=w192:path[])  [unwired: 1 out]
        n106 = for {
          shift-right: [w211] -> w193
          shift-left: "Result files to read" -> [w210]
          tunnel: w192 -> [w208] mode=indexing
          n107 = Search 1D Array(1D array=w210, element=w208) -> (index of element=w209:i32)  [unwired: 1 out]
          n108 = Strip Path(path=w208) -> (name=w207:string)  [unwired: 1 out]
          n109 = Less Than 0?(x=w209) -> (x < 0?=w206:bool)
          n110 = call "Add_filename_suffix.vi"("Filename"=w207) -> ("Original Suffix"=w204:string)  [unwired: 1 in, 3 out]
          n111 = call "Match_Pat_Case_In.vi"("String to match"=".jpg" ("x"), "String"=w204) -> ("offset past match"=w202:i32)  [unwired: 1 in, 3 out]
          n112 = Less Than 0?(x=w202) -> (x < 0?=w201:bool)
          n113 = And(x=w206, y=w201) -> (x .and. y?=w205:bool)
          n114 = case shown="True" w205 {
            tunnel: w210 -> [w212 w215]
            tunnel: w208 -> [_ w214]
            tunnel: [w212 w213] -> w211
            frame False {
            }
            frame True {
              n115 = Build Array (concatenate)(w215, w214) -> (w213:path[])
            }
          }
        }
        n116 = local write "Result files to read"(w193) -> ()
      }
      frame "Selection of files in Folder" {
        n117 = local read "Choosen Path"() -> (w217:path)
        n118 = local read "Result files to read"() -> (w220:path[])
        n119 = File Dialog(7:"Please Choose the folder that contains the Results files to be plotted" ("prompt"), 11:w217) -> (3:w216:path)  [unwired: 1 in, 7 out]
        n120 = call "Get_folder_and_filenames.vi"("file path (dialog if empty)"=w216) -> ("Files"=w222:path[])  [unwired: 1 out]
        n121 = local write "Choosen Path"(w216) -> ()
        n122 = for {
          tunnel: w222 -> [w245] mode=indexing
          tunnel: [w244] -> w225 mode=indexing
          n123 = Strip Path(path=w245) -> (name=w244:string)  [unwired: 1 out]
        }
        n124 = call "Select_Strings.vi"("Available Ch names"=w225, "Message"="Please select the desired data files", "Selector mode"=T6."Zero or more") -> ("Ch Indicies Choosen"=w223:i32[])  [unwired: 1 in, 4 out]
        n125 = for {
          tunnel: w223 -> [w243] mode=indexing
          tunnel: w222 -> [w242]
          tunnel: [w241] -> w218 mode=indexing
          n126 = Index Array(array=w242, index=w243) -> (element=w241:path)
        }
        n127 = for {
          shift-right: [w236] -> w219
          shift-left: w220 -> [w235]
          tunnel: w218 -> [w234] mode=indexing
          n128 = Search 1D Array(1D array=w235, element=w234) -> (index of element=w233:i32)  [unwired: 1 out]
          n129 = Less Than 0?(x=w233) -> (x < 0?=w232:bool)
          n130 = case shown="True" w232 {
            tunnel: w235 -> [w237 w240]
            tunnel: w234 -> [_ w239]
            tunnel: [w237 w238] -> w236
            frame False {
            }
            frame True {
              n131 = Build Array (concatenate)(w240, w239) -> (w238:path[])
            }
          }
        }
        n132 = local write "Result files to read"(w219) -> ()
      }
      frame "Which file to read next" {
        n133 = local read "Result files to read"() -> (w255:path[])
        n134 = local read "File Index"() -> (w252:i32)
        n135 = Array Size(array=w255) -> (size(s)=w253:i32)
        n136 = Equal?(x=w253, y=w252) -> (x = y?=w251:bool)
        n137 = case shown="False" w251 {
          tunnel: w255 -> [w261 _]
          tunnel: [w262 "Load Selectors"] -> w254
          tunnel: w252 -> [w260 w274]
          tunnel: [w259 w274] -> w247
          frame False {
            n138 = Index Array(array=w261, index=w260) -> (element=w263:path)
            n139 = Search 1D Array(1D array="Results files choosen", element=w263) -> (index of element=w265:i32)  [unwired: 1 out]
            n140 = call "Add_filename_suffix.vi"() -> ()  [unwired: 2 in, 4 out]
            n141 = case shown="-1" w265 {
              tunnel: "Results files choosen" -> [_ w273]
              tunnel: w263 -> [w269 w272]
              tunnel: ["Which file to read next" "Load Data"] -> w262
              frame 0, Default {
                n142 = Format Into String(format string="The filename\n \"%s\"\n has already been chosen" ("Format String"), w269) -> (resulting string=w267:string)  [unwired: 2 in, 1 out]
                n143 = One Button Dialog(message=w267) -> ()  [unwired: 2 out]
              }
              frame -1 {
                n144 = Build Array (concatenate)(w273, w272) -> (w271:path[])
                n145 = local write "Results files choosen"(w271) -> ()
              }
            }
            n146 = local write "Results file"(w263) -> ()
            n147 = Increment(x=w260) -> (x+1=w259:i32)
          }
          frame True {
          }
        }
        n148 = local read "stop"() -> (w250:bool)
        n149 = Decrement(x=w247) -> (x-1=w246:i32)
        n150 = Build Array(w246) -> (w248:i32[])
        n151 = Not(x=w250) -> (.not. x?=w249:bool)
        n152 = local write "File Index"(w247) -> ()
        n153 = property on="Result files to read" class="Arr (strict)"("Index Values"=w248) -> ()  [unwired: 2 in, 2 out]
      }
      frame "Load Data" {
        n154 = stacked-sequence {
          seq-local: [w288 _] -> [_ w348]
          seq-local: [w287 _] -> [_ w353]
          seq-local: [w286 _] -> [_ w352]
          seq-local: [w284 _] -> [_ w351]
          tunnel: [TRUE _] -> w283
          tunnel: w282 -> [w302 w354]
          tunnel: w281 -> [w301 _]
          tunnel: [w300 _] -> w280
          tunnel: [w299 _] -> w279
          tunnel: [w298 _] -> w278
          tunnel: w277 -> [w297 _]
          tunnel: ["Which file to read next" _] -> w276
          frame #0 {
            w291 = TRUE  # Add Extra Channels?
            n155 = local read "Template"() -> (w295:path)
            n156 = call "Read_Data_file.vi"("Results file"="Results file", "Add Extra Channels?"=w291, "Template File"=w295, "Desired File Types"="File Types to Read") -> ("Row numbers"=w286:i32[], "Template File Out"=w292:path, "Filetype"=w287:string, "Results file Out"=w288:path, "Ch names Out"=w293:string[], "Channel Values Out"=w289:string[][])  [unwired: 1 in, 9 out]
            n157 = local write "Template"(w292) -> ()
            n158 = Array Size(array=w293) -> (size(s)=w294:i32)
            n159 = Greater Than 0?(x=w294) -> (x > 0?=w284:bool)
            n160 = case shown="True" w284 {
              tunnel: w302 -> [w304 w318]
              tunnel: w301 -> [w306 w312]
              tunnel: w289 -> [_ w310]
              tunnel: [w304 w308] -> w300
              tunnel: [w306 w316] -> w299
              tunnel: [w305 w307] -> w298
              tunnel: w297 -> [w305 _]
              tunnel: w293 -> [_ w311]
              frame False {
              }
              frame True {
                n161 = for {
                  tunnel: w310 -> [w320] mode=indexing
                  tunnel: [w319] -> w309 mode=indexing
                  n162 = for {
                    tunnel: w320 -> [w322] mode=indexing
                    tunnel: [w321] -> w319 mode=indexing
                    n163 = call "Fast_string_Replace.vi"("Replace match with:"="[", "Input String"=w322, "regular expression"="(") -> ("Output String"=w323:string)  [unwired: 2 out]
                    n164 = call "Fast_string_Replace.vi"("Replace match with:"="]", "Input String"=w323, "regular expression"=")") -> ("Output String"=w321:string)  [unwired: 2 out]
                  }
                }
                n165 = call "Merge_channel_names.vi"("Preferred Channel array"=w312, "Channel array"=w311) -> ("Merged Channels"=w316:string[], "Preferred Channels Changed?"=w314:bool, "Channel Array Changed?"=w315:bool)
                n166 = for {
                  tunnel: w316 -> [w345] mode=indexing
                  tunnel: [w342] -> w307 mode=indexing
                  n167 = call "Fast_string_Replace.vi"("Replace match with:"=" ", "Input String"=w345, "regular expression"=":") -> ("Output String"=w341:string)  [unwired: 2 out]
                  n168 = call "Fast_string_Replace.vi"("Replace match with:"=" ", "Input String"=w341, "regular expression"="  ") -> ("Output String"=w340:string)  [unwired: 2 out]
                  n169 = call <vilib>:"Trim Whitespace.vi"("string"=w340) -> ("trimmed string"=w342:string)  [unwired: 1 in]
                }
                n170 = case shown="True" w314 {
                  tunnel: w318 -> [w333 w335]
                  tunnel: w312 -> [_ w337]
                  tunnel: [w333 w334] -> w313
                  tunnel: w316 -> [_ w336]
                  frame False {
                  }
                  frame True {
                    n171 = call "Merge_2D_values.vi"("Values In"=w335, "Present Channels"=w337, "Desired Channels"=w336) -> ("Values Out"=w334:string[][])
                  }
                }
                n172 = case shown="True" w315 {
                  tunnel: [w328 w332] -> w317
                  tunnel: w311 -> [_ w331]
                  tunnel: w309 -> [w328 w330]
                  tunnel: w316 -> [_ w329]
                  frame False {
                  }
                  frame True {
                    n173 = call "Merge_2D_values.vi"("Values In"=w330, "Present Channels"=w331, "Desired Channels"=w329) -> ("Values Out"=w332:string[][])
                  }
                }
                n174 = global write "Results_plotter_Global.vi" "Channel names"(w307) -> ()
                n175 = Build Array (concatenate)(w313, w317) -> (w308:string[][])
                n176 = global write "Results_plotter_Global.vi" "All Data"(w308) -> ()
              }
            }
          }
          frame #1 {
            n177 = local read "File Index"() -> (w350:i32)
            n178 = Decrement(x=w350) -> (x-1=w349:i32)
            n179 = local read "Result files to read"() -> (w347:path[])
            n180 = case shown="True" w351 {
              tunnel: w354 -> [_ w367]
              tunnel: w353 -> [_ w365]
              tunnel: w352 -> [_ w363]
              tunnel: w349 -> [w355 w361]
              tunnel: w348 -> [_ w360]
              tunnel: w347 -> [w357 w362]
              tunnel: [w356 w359] -> w346
              frame False {
                n181 = Delete From Array(array=w357, length=1, index=w355) -> (array with subset deleted=w356:path[])  [unwired: 1 out]
                n182 = local write "File Index"(w355) -> ()
              }
              frame True {
                n183 = Array Size(array=w367) -> (size(s)=w369:i32[])
                n184 = Index Array(array=w369, index=0 ("Index")) -> (element=w366:i32)
                n185 = for {
                  tunnel: w361 -> [w386]
                  tunnel: [w385] -> w371 mode=indexing
                  tunnel: w366 -> [w382]
                  tunnel: w363 -> [w381] mode=indexing
                  i -> [w383]
                  n186 = Add(x=w383, y=w382) -> (x+y=w384:i32)
                  n187 = Build Array(w386, w381, w384) -> (w385:i32[])
                }
                n188 = case shown="1, Default" w361 {
                  tunnel: w371 -> [w374 w379]
                  tunnel: [w374 w378] -> w370
                  tunnel: w365 -> [w373 w377]
                  tunnel: [w372 w375] -> w364
                  frame 0 {
                    n189 = Build Array(w373) -> (w372:string[])
                  }
                  frame 1, Default {
                    n190 = global read "Results_plotter_Global.vi" "Row Reference"() -> (w380:i32[][])
                    n191 = local read "Filetype"() -> (w376:string[])
                    n192 = Build Array (concatenate)(w376, w377) -> (w375:string[])
                    n193 = Build Array (concatenate)(w380, w379) -> (w378:i32[][])
                  }
                }
                "Filetype" <- w364
                n194 = Replace Array Subset(array=w362, new element=w360, index=w361) -> (w359:path[])
                n195 = global write "Results_plotter_Global.vi" "Row Reference"(w370) -> ()
              }
            }
            n196 = local write "Result files to read"(w346) -> ()
          }
        }
      }
      frame "Load Selectors" {
        n197 = while {
          shift-right: [w407] -> w392
          shift-left: _ -> [w409]
          tunnel: [w409] -> w391
          tunnel: w387 -> [w407]
          stop <- FALSE continue-if-true
        }
        n198 = Array Size(array=w399) -> (size(s)=w398:i32[])
        n199 = local read "Tolerances"() -> (w395:dbl[])
        n200 = Index Array(array=w398, index=0 ("Index")) -> (element=→"nRows":i32)
        n201 = Equal?(x=w392, y=w391) -> (x = y?=w390:bool)
        n202 = Build Array (concatenate)("Don't Filter" ("Input Element"), w387) -> (w404:string[])
        n203 = Array Size(array=w387) -> (size(s)=w401:i32)
        n204 = Array Size(array=w395) -> (size(s)=w400:i32)
        n205 = property on="Z Ch Name" class="Ring (strict)"("Strings []"=w387) -> ()  [unwired: 2 in, 2 out]
        n206 = property on="Y Ch Name" class="Ring (strict)"("Strings []"=w387) -> ()  [unwired: 2 in, 2 out]
        n207 = property on="X Ch Name" class="Ring (strict)"("Strings []"=w387) -> ()  [unwired: 2 in, 2 out]
        n208 = property on="X Axis" class="Ring (strict)"("Strings []"=w387) -> ()  [unwired: 2 in, 2 out]
        n209 = property on="Ordinate" class="Ring (strict)"("Strings []"=w387) -> ()  [unwired: 2 in, 2 out]
        n210 = property on="Filter on column 1:" class="Ring (strict)"("Strings []"=w404) -> ()  [unwired: 2 in, 2 out]
        n211 = property on="Multi Ordinate" class="LstBox (strict)"("Item Names"=w387) -> ()  [unwired: 2 in, 2 out]
        n212 = Not Equal?(x=w401, y=w400) -> (x != y?=w402:bool)
        n213 = case shown="True" w402 {
          tunnel: w401 -> [_ w416]
          tunnel: w400 -> [_ w415]
          tunnel: w395 -> [_ w412]
          frame False {
          }
          frame True {
            n214 = Subtract(x=w416, y=w415) -> (x-y=w414:i32)
            n215 = Initialize Array(1.0 ("Element Data"), w414) -> (w411:dbl[])
            n216 = Build Array (concatenate)(w412, w411) -> (w410:dbl[])
            n217 = local write "Tolerances"(w410) -> ()
          }
        }
        n218 = global write "Results_plotter_Global.vi" "First Loop"(TRUE) -> ()
        n219 = Select(t="What is present?", s=w390, f="Set Axis Channels") -> (s? t:f=w394:string)
      }
      frame "Set Axis Channels" {
        n220 = Array Size(array=w423) -> (size(s)=w422:i32)
        n221 = Build Array("X" ("regular expression"), "Y" ("regular expression"), "Z" ("regular expression")) -> (w417:string[])
        n222 = Decrement(x=w422) -> (x-1=w421:i32)
        n223 = for {
          tunnel: w423 -> [w435]
          tunnel: w421 -> [w434]
          tunnel: w417 -> [w433] mode=indexing
          i -> [w429]
          n224 = while {
            tunnel: w435 -> [w449] mode=indexing
            tunnel: w434 -> [w448]
            tunnel: w433 -> [w446]
            tunnel: [w439] -> w432
            tunnel: [w444] -> w431
            i -> [w444]
            stop <- w447 continue-if-true
            n225 = call "Match_Pat_Case_In.vi"("String to match"=w446, "String"=w449) -> ("offset past match"=w443:i32)  [unwired: 1 in, 3 out]
            n226 = In Range and Coerce(upper limit=4, x=w443, lower limit=0) -> (In Range?=w440:bool)  [unwired: 1 out]
            n227 = Less?(x=w444, y=w448) -> (x < y?=w445:bool)
            n228 = Not(x=w440) -> (.not. x?=w439:bool)
            n229 = And(x=w439, y=w445) -> (x .and. y?=w447:bool)
          }
          n230 = Select(t=0, s=w432, f=w431) -> (s? t:f=w428:i32)
          n231 = case shown="1" w429 {
            tunnel: w428 -> [w436 w437 w438]
            frame 0, Default {
              n232 = local write "X Ch Name"(w436) -> ()
            }
            frame 1 {
              n233 = local write "Y Ch Name"(w437) -> ()
            }
            frame 2 {
              n234 = local write "Z Ch Name"(w438) -> ()
            }
          }
        }
      }
      frame "What is present?" {
        n235 = case shown="True" "Show Results Space Analysis" {
          tunnel: w453 -> [_ w457]
          tunnel: w452 -> [_ w456]
          frame False {
          }
          frame True {
            n236 = stacked-sequence {
              tunnel: w457 -> [w461]
              tunnel: w456 -> [w460]
              frame #0 {
                w458 = FALSE  # Summarise All
                n237 = call "Summarise.vi"("Channel Names"=w461, "Data"=w460, "Summarise All"=w458) -> ("Summary"=w459:string[][])  [unwired: 2 in]
                n238 = call "Results_Space_Analysis.vi"("Table"=w459) -> ()
              }
            }
          }
        }
      }
      frame "Ordinate Selector Type" {
        n239 = while {
          tunnel: [w480] -> w471
          shift-left: _ -> [w480]
          shift-right: ["Slice mode"] -> w472
          stop <- FALSE continue-if-true
          "Previous slice mode" <- w480
        }
        n240 = Not(x="Multi Ordinate?") -> (.not. x?=w466:bool)
        n241 = property on="Multi Ordinate" class="LstBox (strict)"("Visible"="Multi Ordinate?") -> ()  [unwired: 2 in, 2 out]
        n242 = property on="Ordinate Name" class="Str"("Visible"="Multi Ordinate?") -> ()  [unwired: 2 in, 2 out]
        n243 = property on="Ordinate" class="Ring (strict)"("Visible"=w466) -> ()  [unwired: 2 in, 2 out]
        n244 = property on="First Add label" class="Str"("Visible"=w466) -> ()  [unwired: 2 in, 2 out]
        n245 = property on="2nd Add label" class="Str"("Visible"=w466) -> ()  [unwired: 2 in, 2 out]
        n246 = property on="Additional Y Values" class="Arr (strict)"("Visible"=w466) -> ()  [unwired: 2 in, 2 out]
        n247 = property on="Additional X Values" class="Arr (strict)"("Visible"=w466) -> ()  [unwired: 2 in, 2 out]
        n248 = Not Equal?(x=w472, y=w471) -> (x != y?=w463:bool)
        n249 = local read "Intensity Plot?"() -> (w470:bool)
        n250 = Or(x=w463, y="Update") -> (x .or. y?=w464:bool)
        n251 = global read "Results_plotter_Global.vi" "First Loop"() -> (w467:bool)
        n252 = case shown="False" "Multi Ordinate?" {
          frame False {
            n253 = Build Array("Ordinate") -> (w482:u16[])
            n254 = local write "Multi Ordinate"(w482) -> ()
          }
          frame True {
          }
        }
        n255 = Compound Arithmetic op=AND(invert w467, w464, w470) -> (w469:bool)
        "Slice mode Change?" <- w469
        n256 = Select(t="Change Slice mode", s=w469, f="Which rows are Non-Blank?") -> (s? t:f=w473:string)
      }
      frame "Change Slice mode" {
        n257 = local read "Previous slice mode"() -> (w486:T3)
        n258 = local read "Slice mode"() -> (w500:T3)
        n259 = case shown="\"YX Slice (Plan)\"" w500 {
          tunnel: [w512 w517 w524 w529 w536 w542] -> w499
          tunnel: "Y Ch Name" -> [w510 w517 w524 w530 w535 w540]
          tunnel: "X Ch Name" -> [w512 w516 w523 w528 w536 w541]
          tunnel: [w511 w518 w523 w528 w535 w540] -> w490
          tunnel: "Z Ch Name" -> [w511 w518 w522 w529 w534 w542]
          tunnel: [w510 w516 w522 w530 w534 w541] -> w488
          tunnel: w486 -> [w509 w514 w520 w526 w533 w538]
          tunnel: [w507 w513 w519 w525 w532 w537] -> w485
          frame "XY Slice (Plan)" {
            n260 = Equal?(x=Plot_Slice."YX Slice (Plan)" ("Previous slice mode"), y=w509) -> (x = y?=w507:bool)
          }
          frame "YX Slice (Plan)" {
            n261 = Equal?(x=Plot_Slice."XY Slice (Plan)" ("Previous slice mode"), y=w514) -> (x = y?=w513:bool)
          }
          frame "YZ Slice (Cross)" {
            n262 = Equal?(x=Plot_Slice."ZY Slice (Cross)" ("Previous slice mode"), y=w520) -> (x = y?=w519:bool)
          }
          frame "ZY Slice (Cross)" {
            n263 = Equal?(x=Plot_Slice."YZ Slice (Cross)" ("Previous slice mode"), y=w526) -> (x = y?=w525:bool)
          }
          frame "XZ Slice (Side)" {
            n264 = Equal?(x=Plot_Slice."ZX Slice (Side)" ("Previous slice mode"), y=w533) -> (x = y?=w532:bool)
          }
          frame "ZX Slice (Side)" {
            n265 = Equal?(x=Plot_Slice."XZ Slice (Side)" ("Previous slice mode"), y=w538) -> (x = y?=w537:bool)
          }
        }
        n266 = case shown="True" w485 {
          frame False {
          }
          frame True {
            n267 = local read "Transpose"() -> (w506:bool)
            n268 = Not(x=w506) -> (.not. x?=w505:bool)
            n269 = local write "Transpose"(w505) -> ()
          }
        }
        n270 = local write "Update"(FALSE ("Update")) -> ()
        n271 = Increment(x=w490) -> (x+1=w493:u16)
        n272 = Increment(x=w488) -> (x+1=w492:u16)
        n273 = local read "Filter Array"() -> (w497:u16[])
        n274 = Array Subset(array=w497, index=2 ("Array Index")) -> (w495:u16[])  [unwired: 1 in]
        n275 = Build Array (concatenate)(w493, w492, w495) -> (w494:u16[])
        n276 = local write "Filter Array"(w494) -> ()
        n277 = local write "Absisca"(w499) -> ()
      }
      frame "Which rows are Non-Blank?" {
        n278 = while {
          tunnel: [w559] -> w553
          tunnel: [w560] -> w554
          shift-left: _ -> [w561]
          shift-right: [w562] -> w546
          shift-left: _ -> [w564]
          shift-right: [w563] -> _
          stop <- FALSE continue-if-true
          n279 = local read "Multi Ordinate"() -> (w562:i32[])
          n280 = local read "Absisca"() -> (w563:u16)
          n281 = Equal?(x=w563, y=w564) -> (x = y?=w560:bool)
          n282 = Equal?(x=w562, y=w561) -> (x = y?=w559:bool)
        }
        n283 = global read "Results_plotter_Global.vi" "First Loop"() -> (w548:bool)
        n284 = Compound Arithmetic op=AND(invert w548, w554, w553) -> (w552:bool)
        n285 = Array Size(array=w546) -> (size(s)=w545:i32)
        n286 = Greater?(x=w545, y=1) -> (0:w543:bool)
        n287 = global write "Results_plotter_Global.vi" "Multi Ordinate?"(w543) -> ()
        n288 = Select(t="Create Selectors", s=w552, f="Evaluate Blank Rows") -> (s? t:f=w549:string)
      }
      frame "Evaluate Blank Rows" {
        n289 = local read "Multi Ordinate"() -> (w566:i32[])
        n290 = local read "Absisca"() -> (w567:u16)
        n291 = for {
          tunnel: w568 -> [w574] mode=indexing
          tunnel: w567 -> [w577]
          tunnel: w566 -> [w576]
          tunnel: [w573] -> w565 mode=indexing
          n292 = Index Array(array=w574, index=w577) -> (element=w578:string)
          n293 = call "Convert_to_number.vi"("string"=w578) -> ("Number"=w579:dbl)  [unwired: 1 out]
          n294 = Not A Number/Path/Refnum?(number/path/refnum=w579) -> (NaN/Path/Refnum?=w575:bool)
          n295 = case shown="False" w575 {
            tunnel: w576 -> [w583 _]
            tunnel: w574 -> [w582 _]
            tunnel: [w580 FALSE] -> w573
            frame False {
              n296 = for {
                tunnel: w583 -> [w589] mode=indexing
                tunnel: w582 -> [w587]
                tunnel: [w584] -> w581 mode=indexing
                n297 = Index Array(array=w587, index=w589) -> (element=w588:string)
                n298 = call "Convert_to_number.vi"("string"=w588) -> ("Number"=w586:dbl)  [unwired: 1 out]
                n299 = Not A Number/Path/Refnum?(number/path/refnum=w586) -> (NaN/Path/Refnum?=w585:bool)
                n300 = Not(x=w585) -> (.not. x?=w584:bool)
              }
              n301 = Or Array Elements(Boolean array=w581) -> (logical OR=w580:bool)
            }
            frame True {
            }
          }
        }
        "Non-Blank Rows" <- w565
      }
      frame "Create Selectors" {
        n302 = local read "Non-Blank Rows"() -> (w594:bool[])
        n303 = local read "Tolerances"() -> (w592:dbl[])
        n304 = global read "Results_plotter_Global.vi" "Precision"() -> (w591:string[])
        n305 = Array Size(array=w602) -> (size(s)=w601:i32[])
        n306 = Index Array(array=w601, index=0 ("Index")) -> (element=w604:i32)
        n307 = for {
          tunnel: w602 -> [w620]
          tunnel: "Filter Array" -> [w612] mode=indexing
          shift-right: [w619] -> w593
          shift-left: _ -> [w617]
          tunnel: w604 -> [w618]
          tunnel: [w615] -> w599 mode=indexing
          tunnel: w594 -> [w614]
          tunnel: w592 -> [w613]
          tunnel: w591 -> [w610]
          i -> [w616]
          n308 = Decrement(x=w612) -> (x-1=w609:u16)
          n309 = Index Array(array=w610, index=w609) -> (element=w608:string)
          n310 = Index Array(array=w613, index=w609) -> (element=w611:dbl)
          n311 = case shown="1" w616 {
            tunnel: w620 -> [w633 w669 w710 w751 w792 w835 w876]
            tunnel: w612 -> [w632 w668 w709 w750 w791 w834 w875]
            tunnel: w611 -> [w631 w667 w708 w749 w790 w833 w874]
            tunnel: [w630 w666 w707 w748 w789 w832 w873] -> w619
            tunnel: w618 -> [w628 w665 w706 w747 w788 w831 w872]
            tunnel: w617 -> [_ w664 w705 w746 w787 w830 w871]
            tunnel: w616 -> [w627 w663 w702 w743 w784 w829 w868]
            tunnel: [w623 w658 w701 w742 w783 w824 w867] -> w615
            tunnel: w614 -> [w622 w657 w700 w741 w782 w823 w866]
            tunnel: w608 -> [w621 w656 w699 w740 w781 w822 w865]
            frame 0, Default {
              n312 = case shown="1, Default" w632 {
                tunnel: w633 -> [w639 w649]
                tunnel: w632 -> [w640 w648]
                tunnel: w631 -> [_ w655]
                tunnel: [w635 w652] -> w630
                tunnel: "Filter Bins 1" -> [_ w653]
                tunnel: [string[] [] ("Write Attribute") w654] -> w629
                tunnel: w628 -> [w637 _]
                tunnel: w627 -> [w643 w651]
                tunnel: [i32[] [0] ("Filter Bins Out") w650] -> w625
                tunnel: [TRUE ("Unchanged?") w647] -> w623
                tunnel: w622 -> [_ w646]
                tunnel: w621 -> [_ w645]
                frame 0 {
                  n313 = call "Create_filter_points.vi"("Channel to Filter On"=w640, "Index"=w643, "Ch Values In"=w639) -> ()  [unwired: 4 in, 4 out]
                  n314 = Initialize Array(TRUE, w637) -> (w636:bool[])
                  n315 = Build Array(w636) -> (w635:bool[][])
                }
                frame 1, Default {
                  n316 = call "Create_filter_points.vi"("Non-Blank Rows"=w646, "Precision"=w645, "Channel to Filter On"=w648, "Tolerance"=w655, "Index"=w651, "Filter Bins 1"=w653, "Ch Values In"=w649) -> ("Unchanged?"=w647:bool, "Accept array"=w652:bool[][], "Filter Bins Out"=w650:i32[], "Bin Names"=w654:string[])
                }
              }
              n317 = Equal?(x="Filter Bins 1", y=w625) -> (x = y?=w624:bool)
              n318 = case shown="False" w624 {
                tunnel: w625 -> [w634 _]
                frame False {
                  n319 = local write "Filter Bins 1"(w634) -> ()
                }
                frame True {
                }
              }
              n320 = property on="Filter bins 1" class="LstBox (strict)"("Item Names"=w629) -> ()  [unwired: 2 in, 2 out]
            }
            frame 1 {
              n321 = case shown="1, Default" w668 {
                tunnel: w669 -> [_ w681]
                tunnel: w668 -> [w672 w680]
                tunnel: w667 -> [_ w688]
                tunnel: [w676 w684] -> w666
                tunnel: "Filter Bins 2" -> [_ w686]
                tunnel: [string[] [] ("Write Attribute") w690] -> w662
                tunnel: w665 -> [_ _]
                tunnel: w664 -> [w676 w689]
                tunnel: w663 -> [w675 w687]
                tunnel: [i32[] [0] ("Filter Bins Out") w682] -> w661
                tunnel: [TRUE ("Unchanged?") w679] -> w658
                tunnel: w657 -> [_ w678]
                tunnel: w656 -> [_ w677]
                frame 0 {
                  n322 = call "Create_filter_points.vi"("Channel to Filter On"=w672, "Index"=w675) -> ()  [unwired: 5 in, 4 out]
                }
                frame 1, Default {
                  n323 = call "Create_filter_points.vi"("Non-Blank Rows"=w678, "Precision"=w677, "Channel to Filter On"=w680, "Tolerance"=w688, "Index"=w687, "Filter Bins 1"=w686, "Ch Values In"=w681) -> ("Unchanged?"=w679:bool, "Accept array"=w685:bool[][], "Filter Bins Out"=w682:i32[], "Bin Names"=w690:string[])
                  n324 = for {
                    tunnel: w689 -> [w695]
                    tunnel: w685 -> [w694] mode=indexing
                    shift-right: [w691] -> w684
                    shift-left: bool[][] [] -> [w693]
                    n325 = for {
                      tunnel: w694 -> [w698]
                      tunnel: w695 -> [w697] mode=indexing
                      tunnel: [w696] -> _ mode=indexing
                      tunnel: [w696] -> w692 mode=indexing
                      n326 = And(x=w698, y=w697) -> (x .and. y?=w696:bool[])
                    }
                    n327 = Build Array (concatenate)(w693, w692) -> (w691:bool[][])
                  }
                }
              }
              n328 = Equal?(x="Filter Bins 2", y=w661) -> (x = y?=w659:bool)
              n329 = case shown="False" w659 {
                tunnel: w661 -> [w670 _]
                frame False {
                  n330 = local write "Filter Bins 2"(w670) -> ()
                }
                frame True {
                }
              }
              n331 = property on="Filter Bins 2" class="LstBox (strict)"("Item Names"=w662) -> ()  [unwired: 2 in, 2 out]
            }
            frame 2 {
              n332 = case shown="0" w709 {
                tunnel: w710 -> [_ w720]
                tunnel: w709 -> [w713 w721]
                tunnel: w708 -> [_ w732]
                tunnel: [w716 w733] -> w707
                tunnel: "Filter 3" -> [_ w724]
                tunnel: [string[] [] ("Write Attribute") w735] -> w703
                tunnel: w706 -> [_ _]
                tunnel: w705 -> [w716 w734]
                tunnel: w702 -> [w715 w727]
                tunnel: [TRUE ("Unchanged?") w719] -> w701
                tunnel: w700 -> [_ w718]
                tunnel: w699 -> [_ w717]
                frame 0 {
                  n333 = call "Create_filter_points.vi"("Channel to Filter On"=w713, "Index"=w715) -> ()  [unwired: 5 in, 4 out]
                  n334 = local write "Filter 3"(0) -> ()
                }
                frame 1, Default {
                  n335 = Build Array(w724) -> (w731:u16[])
                  n336 = call "Create_filter_points.vi"("Non-Blank Rows"=w718, "Precision"=w717, "Channel to Filter On"=w721, "Tolerance"=w732, "Index"=w727, "Filter Bins 1"=w731, "Ch Values In"=w720) -> ("Unchanged?"=w719:bool, "Accept array"=w729:bool[][], "Filter Bins Out"=w725:i32[], "Bin Names"=w735:string[])
                  n337 = Index Array(array=w725, index=0 ("Index")) -> (element=w722:i32)
                  n338 = Index Array(array=w729, index (row)=0 ("Index")) -> (element=w728:bool[])  [unwired: 1 in]
                  n339 = Equal?(x=w724, y=w722) -> (x = y?=w723:bool)
                  n340 = case shown="True" w723 {
                    tunnel: w722 -> [w736 _]
                    frame False {
                      n341 = local write "Filter 3"(w736) -> ()
                    }
                    frame True {
                    }
                  }
                  n342 = for {
                    tunnel: w728 -> [w739]
                    tunnel: w734 -> [w738] mode=indexing
                    tunnel: [w737] -> w733 mode=indexing
                    n343 = And(x=w739, y=w738) -> (x .and. y?=w737:bool[])
                  }
                }
              }
              n344 = property on="Filter 3" class="Ring (strict)"("Strings []"=w703) -> ()  [unwired: 2 in, 2 out]
            }
            frame 3 {
              n345 = case shown="1, Default" w750 {
                tunnel: w751 -> [_ w762]
                tunnel: w750 -> [w754 w761]
                tunnel: w749 -> [_ w773]
                tunnel: [w757 w774] -> w748
                tunnel: "Filter 4" -> [_ w765]
                tunnel: [string[] [] ("Write Attribute") w776] -> w744
                tunnel: w747 -> [_ _]
                tunnel: w746 -> [w757 w775]
                tunnel: w743 -> [w756 w768]
                tunnel: [TRUE ("Unchanged?") w760] -> w742
                tunnel: w741 -> [_ w759]
                tunnel: w740 -> [_ w758]
                frame 0 {
                  n346 = call "Create_filter_points.vi"("Channel to Filter On"=w754, "Index"=w756) -> ()  [unwired: 5 in, 4 out]
                  n347 = local write "Filter 4"(0) -> ()
                }
                frame 1, Default {
                  n348 = Build Array(w765) -> (w772:u16[])
                  n349 = call "Create_filter_points.vi"("Non-Blank Rows"=w759, "Precision"=w758, "Channel to Filter On"=w761, "Tolerance"=w773, "Index"=w768, "Filter Bins 1"=w772, "Ch Values In"=w762) -> ("Unchanged?"=w760:bool, "Accept array"=w770:bool[][], "Filter Bins Out"=w766:i32[], "Bin Names"=w776:string[])
                  n350 = Index Array(array=w766, index=0 ("Index")) -> (element=w764:i32)
                  n351 = Equal?(x=w765, y=w764) -> (x = y?=w763:bool)
                  n352 = Index Array(array=w770, index (row)=0 ("Index")) -> (element=w769:bool[])  [unwired: 1 in]
                  n353 = case shown="False" w763 {
                    tunnel: w764 -> [w777 _]
                    frame False {
                      n354 = local write "Filter 4"(w777) -> ()
                    }
                    frame True {
                    }
                  }
                  n355 = for {
                    tunnel: w769 -> [w780]
                    tunnel: w775 -> [w779] mode=indexing
                    tunnel: [w778] -> w774 mode=indexing
                    n356 = And(x=w780, y=w779) -> (x .and. y?=w778:bool[])
                  }
                }
              }
              n357 = property on="Filter 4" class="Ring (strict)"("Strings []"=w744) -> ()  [unwired: 2 in, 2 out]
            }
            frame 4 {
              n358 = case shown="1, Default" w791 {
                tunnel: w792 -> [_ w803]
                tunnel: w791 -> [w795 w802]
                tunnel: w790 -> [_ w814]
                tunnel: [w798 w815] -> w789
                tunnel: "Filter 5" -> [_ w805]
                tunnel: [string[] [] ("Write Attribute") w817] -> w785
                tunnel: w788 -> [_ _]
                tunnel: w787 -> [w798 w816]
                tunnel: w784 -> [w797 w809]
                tunnel: [TRUE ("Unchanged?") w801] -> w783
                tunnel: w782 -> [_ w800]
                tunnel: w781 -> [_ w799]
                frame 0 {
                  n359 = call "Create_filter_points.vi"("Channel to Filter On"=w795, "Index"=w797) -> ()  [unwired: 5 in, 4 out]
                  n360 = local write "Filter 5"(0) -> ()
                }
                frame 1, Default {
                  n361 = Build Array(w805) -> (w813:u16[])
                  n362 = call "Create_filter_points.vi"("Non-Blank Rows"=w800, "Precision"=w799, "Channel to Filter On"=w802, "Tolerance"=w814, "Index"=w809, "Filter Bins 1"=w813, "Ch Values In"=w803) -> ("Unchanged?"=w801:bool, "Accept array"=w811:bool[][], "Filter Bins Out"=w807:i32[], "Bin Names"=w817:string[])
                  n363 = Index Array(array=w807, index=0 ("Index")) -> (element=w806:i32)
                  n364 = Equal?(x=w805, y=w806) -> (x = y?=w804:bool)
                  n365 = Index Array(array=w811, index (row)=0 ("Index")) -> (element=w810:bool[])  [unwired: 1 in]
                  n366 = case shown="False" w804 {
                    tunnel: w806 -> [w818 _]
                    frame False {
                      n367 = local write "Filter 5"(w818) -> ()
                    }
                    frame True {
                    }
                  }
                  n368 = for {
                    tunnel: w810 -> [w821]
                    tunnel: w816 -> [w820] mode=indexing
                    tunnel: [w819] -> w815 mode=indexing
                    n369 = And(x=w821, y=w820) -> (x .and. y?=w819:bool[])
                  }
                }
              }
              n370 = property on="Filter 5" class="Ring (strict)"("Strings []"=w785) -> ()  [unwired: 2 in, 2 out]
            }
            frame 5 {
              n371 = case shown="1, Default" w834 {
                tunnel: w835 -> [_ w852]
                tunnel: w834 -> [w838 w851]
                tunnel: w833 -> [_ w856]
                tunnel: [w842 w843] -> w832
                tunnel: "Single Series" -> [_ w854]
                tunnel: [string[] [] ("Write Attribute") w858] -> w828
                tunnel: w831 -> [_ _]
                tunnel: w830 -> [w842 w857]
                tunnel: w829 -> [w841 w855]
                tunnel: [i32[] [0] ("Filter Bins Out") w853] -> w827
                tunnel: [TRUE ("Unchanged?") w850] -> w824
                tunnel: w823 -> [_ w849]
                tunnel: w822 -> [_ w848]
                frame 0 {
                  n372 = call "Create_filter_points.vi"("Channel to Filter On"=w838, "Index"=w841) -> ()  [unwired: 5 in, 4 out]
                }
                frame 1, Default {
                  n373 = call "Create_filter_points.vi"("Non-Blank Rows"=w849, "Precision"=w848, "Channel to Filter On"=w851, "Tolerance"=w856, "Index"=w855, "Filter Bins 1"=w854, "Ch Values In"=w852) -> ("Unchanged?"=w850:bool, "Accept array"=w845:bool[][], "Filter Bins Out"=w853:i32[], "Bin Names"=w858:string[])
                  n374 = Index Array(array=w845, index (row)=0 ("Index")) -> (element=w846:bool[])  [unwired: 1 in]
                  n375 = for {
                    shift-right: [w859] -> w844
                    shift-left: w846 -> [w861]
                    tunnel: w845 -> [w860] mode=indexing
                    n376 = Or(x=w860, y=w861) -> (x .or. y?=w859:bool[])
                  }
                  n377 = for {
                    tunnel: w844 -> [w864]
                    tunnel: w857 -> [w863] mode=indexing
                    tunnel: [w862] -> w843 mode=indexing
                    n378 = And(x=w864, y=w863) -> (x .and. y?=w862:bool[])
                  }
                }
              }
              n379 = Equal?(x="Single Series", y=w827) -> (x = y?=w825:bool)
              n380 = case shown="False" w825 {
                tunnel: w827 -> [w836 _]
                frame False {
                  n381 = local write "Single Series"(w836) -> ()
                }
                frame True {
                }
              }
              n382 = property on="Single Series" class="LstBox (strict)"("Item Names"=w828) -> ()  [unwired: 2 in, 2 out]
            }
            frame 6 {
              n383 = case shown="1, Default" w875 {
                tunnel: w876 -> [_ w887]
                tunnel: w875 -> [w879 w886]
                tunnel: w874 -> [_ w894]
                tunnel: [w882 w899] -> w873
                tunnel: "Filter 6" -> [_ w889]
                tunnel: [string[] [] ("Write Attribute") w901] -> w869
                tunnel: w872 -> [_ _]
                tunnel: w871 -> [w882 w900]
                tunnel: w868 -> [w881 w893]
                tunnel: [TRUE ("Unchanged?") w885] -> w867
                tunnel: w866 -> [_ w884]
                tunnel: w865 -> [_ w883]
                frame 0 {
                  n384 = call "Create_filter_points.vi"("Channel to Filter On"=w879, "Index"=w881) -> ()  [unwired: 5 in, 4 out]
                  n385 = local write "Filter 6"(0) -> ()
                }
                frame 1, Default {
                  n386 = Build Array(w889) -> (w895:u16[])
                  n387 = call "Create_filter_points.vi"("Non-Blank Rows"=w884, "Precision"=w883, "Channel to Filter On"=w886, "Tolerance"=w894, "Index"=w893, "Filter Bins 1"=w895, "Ch Values In"=w887) -> ("Unchanged?"=w885:bool, "Accept array"=w897:bool[][], "Filter Bins Out"=w891:i32[], "Bin Names"=w901:string[])
                  n388 = Index Array(array=w891, index=0 ("Index")) -> (element=w890:i32)
                  n389 = Equal?(x=w889, y=w890) -> (x = y?=w888:bool)
                  n390 = Index Array(array=w897, index (row)=0 ("Index")) -> (element=w896:bool[])  [unwired: 1 in]
                  n391 = case shown="False" w888 {
                    tunnel: w890 -> [w902 _]
                    frame False {
                      n392 = local write "Filter 6"(w902) -> ()
                    }
                    frame True {
                    }
                  }
                  n393 = for {
                    tunnel: w896 -> [w905]
                    tunnel: w900 -> [w904] mode=indexing
                    tunnel: [w903] -> w899 mode=indexing
                    n394 = And(x=w905, y=w904) -> (x .and. y?=w903:bool[])
                  }
                }
              }
              n395 = property on="Filter 6" class="Ring (strict)"("Strings []"=w869) -> ()  [unwired: 2 in, 2 out]
            }
          }
        }
        "Accept Array" <- w593
        n396 = And Array Elements(Boolean array=w599) -> (logical AND=w598:bool)
        n397 = Select(t="Select all for Filter 2", s=w598, f="Create Selectors") -> (s? t:f=w596:string)
      }
      frame "Select all for Filter 2" {
        n398 = local read "Slice mode Change?"() -> (w907:bool)
        n399 = case shown="True" w907 {
          frame False {
          }
          frame True {
            n400 = property on="Filter Bins 2" class="LstBox (strict)"() -> ("Item Names"=w921:string[])  [unwired: 2 in, 2 out]
            n401 = Array Size(array=w921) -> (size(s)=w920:i32)
            n402 = Build Array("Blanks", "Numeric", "Non Numeric", "Non Blanks", "Show All" ("Input Element")) -> (w914:string[])
            n403 = local read "Filter Bins 1"() -> (w923:i32[])
            n404 = while {
              tunnel: w921 -> [w936] mode=indexing
              tunnel: w920 -> [w939]
              shift-right: [w930] -> w912
              shift-left: i32[] [] -> [w931]
              tunnel: w914 -> [w933]
              i -> [w932]
              stop <- w937 stop-if-true
              n405 = String Subset(string=w936, length (rest)=4 ("length (rest)")) -> (substring=w941:string)  [unwired: 1 out]
              n406 = Match Pattern(string=w936, regular expression=" (") -> (before substring=w934:string)  [unwired: 4 out]
              n407 = Search 1D Array(1D array=w933, element=w934) -> (index of element=w929:i32)  [unwired: 1 out]
              n408 = Equal?(x="NOT ", y=w941) -> (x = y?=w928:bool)
              n409 = Equal?(x=w939, y=w932) -> (x = y?=w938:bool)
              n410 = Less Than 0?(x=w929) -> (x < 0?=w927:bool)
              n411 = Or(x=w928, y=w938) -> (x .or. y?=w937:bool)
              n412 = Compound Arithmetic op=AND(w927, invert w928) -> (w926:bool)
              n413 = case shown="False" w926 {
                tunnel: w932 -> [_ w946]
                tunnel: w931 -> [w943 w945]
                tunnel: [w943 w944] -> w930
                frame False {
                }
                frame True {
                  n414 = Build Array (concatenate)(w945, w946) -> (w944:i32[])
                }
              }
            }
            n415 = Array Size(array=w923) -> (size(s)=w925:i32)
            n416 = case shown="1" w925 {
              tunnel: [w947 w950] -> w924
              tunnel: w923 -> [_ w949]
              tunnel: i32[] [1] ("Filter Bins 1") -> [w947 w948]
              frame 0, Default {
              }
              frame 1 {
                n417 = Index Array(array=w949, index=0 ("Index")) -> (element=w952:i32)
                n418 = Greater Than 0?(x=w952) -> (x > 0?=w951:bool)
                n419 = Select(t=w949, s=w951, f=w948) -> (s? t:f=w950:i32[])
              }
            }
            n420 = local write "Filter Bins 1"(w924) -> ()
            n421 = local write "Filter Bins 2"(w912) -> ()
          }
        }
      }
      frame "Re Plot Data?" {
        n422 = while {
          tunnel: [w1000] -> w962
          shift-left: _ -> [w1002]
          shift-right: [w1001] -> _
          tunnel: [w1005] -> w968
          shift-left: _ -> [w1003]
          shift-right: [w1004] -> _
          tunnel: [w1009] -> w970
          shift-left: _ -> [w1008]
          shift-right: [w1007] -> w954
          tunnel: [w1010] -> w971
          shift-left: _ -> [w1012]
          shift-right: [w1011] -> _
          tunnel: [w1014] -> w972
          shift-left: _ -> [w1013]
          shift-right: [w1006] -> _
          tunnel: [w1015] -> w975
          tunnel: [w1016] -> w976
          shift-left: _ -> [w1017]
          shift-right: [w1018] -> _
          shift-left: _ -> [w1020]
          shift-right: [w1019] -> _
          tunnel: [w1021] -> w955
          shift-left: _ -> [w1022]
          shift-right: [w1023] -> _
          tunnel: [w998] -> w965
          shift-right: [w995] -> _
          shift-left: _ -> [w994]
          tunnel: [w997] -> w964
          shift-right: [w993] -> _
          shift-left: _ -> [w996]
          tunnel: [w990] -> w963
          shift-right: [w991] -> _
          shift-left: _ -> [w992]
          shift-right: [w988] -> _
          shift-left: _ -> [w989]
          tunnel: [w987] -> w957
          stop <- FALSE continue-if-true
          n423 = local read "Ordinate Name"() -> (w988:string)
          n424 = local read "Additional X Values"() -> (w995:dbl[])
          n425 = local read "Additional Y Values"() -> (w993:dbl[])
          n426 = local read "Intensity Plot?"() -> (w1007:bool)
          n427 = local read "Accept Array"() -> (w1023:bool[][])
          n428 = local read "color and symbol"() -> (w991:bool)
          n429 = local read "No of Contours"() -> (w1004:i32)
          n430 = local read "Point Size"() -> (w1001:i32)
          n431 = local read "Multi Ordinate"() -> (w1018:i32[])
          n432 = local read "Transpose"() -> (w1006:bool)
          n433 = local read "Resolution"() -> (w1011:dbl)
          n434 = local read "Absisca"() -> (w1019:u16)
          n435 = Equal?(x=w988, y=w989) -> (x = y?=w987:bool)
          n436 = Equal?(x=w1006, y=w1013) -> (x = y?=w1014:bool)
          n437 = Equal?(x=w991, y=w992) -> (x = y?=w990:bool)
          n438 = Equal?(x=w1004, y=w1003) -> (x = y?=w1005:bool)
          n439 = Equal?(x=w1001, y=w1002) -> (x = y?=w1000:bool)
          n440 = Equal?(x=w1011, y=w1012) -> (x = y?=w1010:bool)
          n441 = Equal?(x=w995, y=w994) -> (x = y?=w998:bool)
          n442 = Equal?(x=w993, y=w996) -> (x = y?=w997:bool)
          n443 = Equal?(x=w1019, y=w1020) -> (x = y?=w1016:bool)
          n444 = Equal?(x=w1023, y=w1022) -> (x = y?=w1021:bool)
          n445 = Equal?(x=w1007, y=w1008) -> (x = y?=w1009:bool)
          n446 = Equal?(x=w1018, y=w1017) -> (x = y?=w1015:bool)
        }
        n447 = global read "Results_plotter_Global.vi" "First Loop"() -> (w966:bool)
        n448 = while {
          shift-right: [w986] -> _
          shift-left: _ -> [w985]
          shift-right: [w983] -> _
          shift-left: _ -> [w984]
          tunnel: [w982] -> w961
          tunnel: [w981] -> w960
          stop <- FALSE continue-if-true
          n449 = local read "Filter Bins 1"() -> (w983:i32[])
          n450 = local read "Filter Bins 2"() -> (w986:i32[])
          n451 = Equal?(x=w983, y=w984) -> (x = y?=w981:bool)
          n452 = Equal?(x=w986, y=w985) -> (x = y?=w982:bool)
        }
        n453 = Not(x=w954) -> (.not. x?=w958:bool)
        n454 = property on="Resolution" class="DigNum (strict)"("Visible"=w954) -> ()  [unwired: 2 in, 2 out]
        n455 = property on="Bkgnd Value" class="DigNum (strict)"("Visible"=w954) -> ()  [unwired: 2 in, 2 out]
        n456 = property on="Intensity Graph" class="IntGraph (strict)"("Visible"=w954) -> ()  [unwired: 2 in, 2 out]
        n457 = property on="XY Plot" class="XYGraph (strict)"("Visible"=w958) -> ()  [unwired: 2 in, 2 out]
        n458 = Compound Arithmetic op=AND(w961, w960) -> (w959:bool)
        n459 = Compound Arithmetic op=AND(w957, w959, w962, w963, w968, w971, w972, w976, w975, w955, w970, w965, w964, invert w966) -> (w974:bool)
        n460 = Select(t="What to do next?", s=w974, f="Prepare for Plotting") -> (s? t:f=w973:string)
      }
      frame "Prepare for Plotting" {
        n461 = local read "Filter Array"() -> (w1032:u16[])
        n462 = local read "Multi Ordinate"() -> (w1027:i32[])
        n463 = Index Array(array=w1032, index=0 ("Index")) -> (element=w1029:u16)
        n464 = Equal To 0?(x=w1029) -> (x = 0?=w1030:bool)
        n465 = for {
          tunnel: w1027 -> [w1038] mode=indexing
          tunnel: [w1037] -> w1025 mode=indexing
          tunnel: w1026 -> [w1036]
          n466 = Index Array(array=w1036, index=w1038) -> (element=w1037:string)
        }
        n467 = case shown="False" w1030 {
          tunnel: w1029 -> [w1044 _]
          tunnel: w1026 -> [w1042 _]
          tunnel: [w1039 string[] []] -> w1024
          frame False {
            n468 = Decrement(x=w1044) -> (x-1=w1043:u16)
            n469 = local read "Filter Bins 1"() -> (w1046:i32[])
            n470 = property on="Filter bins 1" class="LstBox (strict)"() -> ("Item Names"=w1045:string[])  [unwired: 2 in, 2 out]
            n471 = Index Array(array=w1042, index=w1043) -> (element=w1040:string)
            n472 = for {
              tunnel: w1046 -> [w1049] mode=indexing
              tunnel: w1045 -> [w1048]
              tunnel: [w1047] -> w1041 mode=indexing
              n473 = Index Array(array=w1048, index=w1049) -> (element=w1047:string)
            }
            n474 = Build Array (concatenate)(w1040, w1041) -> (w1039:string[])
          }
          frame True {
          }
        }
        n475 = global write "Results_plotter_Global.vi" "Ordinate Strings"(w1025) -> ()
        n476 = global write "Results_plotter_Global.vi" "Filter 1 Strings"(w1024) -> ()
      }
      frame "Prepare Filter2 strings" {
        n477 = local read "Filter Array"() -> (w1057:u16[])
        n478 = Index Array(array=w1057, index=1 ("Index")) -> (element=w1054:u16)
        n479 = Equal To 0?(x=w1054) -> (x = 0?=w1055:bool)
        n480 = case shown="False" w1055 {
          tunnel: w1054 -> [w1066 _]
          tunnel: w1053 -> [w1064 _]
          tunnel: [w1061 string[] []] -> w1051
          frame False {
            n481 = Decrement(x=w1066) -> (x-1=w1065:u16)
            n482 = local read "Filter Bins 2"() -> (w1068:i32[])
            n483 = property on="Filter Bins 2" class="LstBox (strict)"() -> ("Item Names"=w1067:string[])  [unwired: 2 in, 2 out]
            n484 = Index Array(array=w1064, index=w1065) -> (element=w1062:string)
            n485 = for {
              tunnel: w1068 -> [w1071] mode=indexing
              tunnel: w1067 -> [w1070]
              tunnel: [w1069] -> w1063 mode=indexing
              n486 = Index Array(array=w1070, index=w1071) -> (element=w1069:string)
            }
            n487 = Build Array (concatenate)(w1062, w1063) -> (w1061:string[])
          }
          frame True {
          }
        }
        n488 = global write "Results_plotter_Global.vi" "Filter 2 Strings"(w1051) -> ()
      }
      frame "Plot Data" {
        n489 = stacked-sequence {
          seq-local: [w1078 _ _] -> [_ w1114 _]
          seq-local: [w1079 _ _] -> [_ w1113 _]
          tunnel: w1076 -> [_ w1123 _]
          tunnel: [_ TRUE _] -> w1075
          tunnel: [_ _ w1141] -> w1074
          tunnel: w1073 -> [w1080 _ _]
          frame #0 {
            n490 = global read "Results_plotter_Global.vi" "Ordinate Strings"() -> (w1078:string[])
            n491 = for {
              tunnel: w1078 -> [w1082] mode=indexing
              tunnel: w1080 -> [w1085]
              tunnel: [w1083] -> w1079 mode=indexing
              n492 = String Length(string=w1082) -> (length=w1081:i32)
              n493 = for {
                tunnel: w1082 -> [w1089]
                tunnel: w1085 -> [w1086] mode=indexing
                shift-right: [w1093] -> w1083
                shift-left: -1 -> [w1091]
                tunnel: w1081 -> [w1087]
                i -> [w1092]
                n494 = String Subset(string=w1086, length (rest)=w1087) -> (substring=w1088:string)  [unwired: 1 out]
                n495 = Equal?(x=w1088, y=w1089) -> (x = y?=w1090:bool)
                n496 = case shown="True" w1090 {
                  tunnel: [w1105 w1108] -> w1093
                  tunnel: w1092 -> [w1104 _]
                  tunnel: w1091 -> [w1103 w1108]
                  tunnel: w1087 -> [w1102 _]
                  tunnel: w1086 -> [w1101 _]
                  frame True {
                    n497 = String Subset(string=w1101, offset (0)=w1102) -> (substring=w1095:string)  [unwired: 1 out]
                    n498 = call <vilib>:"Trim Whitespace.vi"("string"=w1095) -> ("trimmed string"=w1094:string)  [unwired: 1 in]
                    n499 = Equal?(x=w1094, y="Err") -> (x = y?=w1097:bool)
                    n500 = Equal?(x=w1094, y="err") -> (x = y?=w1098:bool)
                    n501 = Or(x=w1097, y=w1098) -> (x .or. y?=w1096:bool)
                    n502 = case shown="True" w1096 {
                      tunnel: [w1106 w1107] -> w1105
                      tunnel: w1104 -> [w1106 _]
                      tunnel: w1103 -> [_ w1107]
                      frame True {
                      }
                      frame False {
                      }
                    }
                  }
                  frame False {
                  }
                }
              }
            }
          }
          frame #1 {
            n503 = global read "Results_plotter_Global.vi" "Filter 1 Strings"() -> (w1109:string[])
            n504 = global read "Results_plotter_Global.vi" "Filter 2 Strings"() -> (w1110:string[])
            n505 = local read "Accept Array"() -> (w1125:bool[][])
            n506 = local read "Multi Ordinate?"() -> (w1119:bool)
            n507 = Select(t=5, s=w1119, f=2 ("y")) -> (s? t:f=w1117:i32)
            n508 = global write "Results_plotter_Global.vi" "Ordinate"("Multi Ordinate") -> ()
            n509 = global write "Results_plotter_Global.vi" "Absisca"("Absisca") -> ()
            n510 = global write "Results_plotter_Global.vi" "Transpose"("Transpose") -> ()
            n511 = while {
              shift-right: [w1128] -> w1122
              shift-left: _ -> [w1129]
              tunnel: "color and symbol" -> [w1130]
              tunnel: w1117 -> [w1126]
              stop <- FALSE continue-if-true
              n512 = case shown="True" w1130 {
                tunnel: w1129 -> [w1137 w1139]
                tunnel: [w1136 w1139] -> w1128
                tunnel: w1126 -> [w1131 _]
                frame True {
                  n513 = Add(x=w1137, y=1) -> (x+y=w1134:i32)
                  n514 = local write "color and symbol"(FALSE ("color and symbol")) -> ()
                  n515 = Greater?(x=w1134, y=w1131) -> (0:w1135:bool)
                  n516 = Select(t=0, s=w1135, f=w1134) -> (s? t:f=w1136:i32)
                }
                frame False {
                }
              }
            }
            n517 = call "Plot_XY_data.vi"("Channel Values"=w1123, "Ordinate Strings"=w1114, "Swap color and symbol"=w1122, "Error Bar Chs"=w1113, "Accept Array"=w1125, "Filter 1 Strings"=w1109, "Filter 2 Strings"=w1110, "Ordinate"="Multi Ordinate", "Absisca"="Absisca", "Transpose"="Transpose") -> ("Accept Array Out"=→"Plotted Series":bool[][])  [unwired: 5 out]
          }
          frame #2 {
            n518 = Select(t="Intensity plot", s="Intensity Plot?", f="Add Legend and scales") -> (s? t:f=w1141:string)
            n519 = property on="Surface Area" class="DigNum (strict)"("Visible"="Intensity Plot?") -> ()  [unwired: 2 in, 2 out]
            n520 = property on="Surface Integral" class="DigNum (strict)"("Visible"="Intensity Plot?") -> ()  [unwired: 2 in, 2 out]
            n521 = property on="Surface Average" class="DigNum (strict)"("Visible"="Intensity Plot?") -> ()  [unwired: 2 in, 2 out]
            n522 = property on="X Ch Name" class="Ring (strict)"("Visible"="Intensity Plot?") -> ()  [unwired: 2 in, 2 out]
            n523 = property on="Y Ch Name" class="Ring (strict)"("Visible"="Intensity Plot?") -> ()  [unwired: 2 in, 2 out]
            n524 = property on="Z Ch Name" class="Ring (strict)"("Visible"="Intensity Plot?") -> ()  [unwired: 2 in, 2 out]
            n525 = property on="Point Size" class="Slide (strict)"("Visible"="Intensity Plot?") -> ()  [unwired: 2 in, 2 out]
            n526 = property on="No of Contours" class="DigNum (strict)"("Visible"="Intensity Plot?") -> ()  [unwired: 2 in, 2 out]
            n527 = property on="Slice mode" class="Enum (strict)"("Visible"="Intensity Plot?") -> ()  [unwired: 2 in, 2 out]
            n528 = property on="Plot Resolution" class="Bool (strict)"("Visible"="Intensity Plot?") -> ()  [unwired: 2 in, 2 out]
            n529 = property on="Update" class="Bool (strict)"("Visible"="Intensity Plot?") -> ()  [unwired: 2 in, 2 out]
          }
        }
      }
      frame "Add Legend and scales" {
        n530 = local read "Transpose"() -> (w1147:bool)
        n531 = global read "Results_plotter_Global.vi" "Plot Index values"() -> (w1150:dbl[][])
        n532 = global read "Results_plotter_Global.vi" "XY Graph Cluster"() -> (→"XY Plot":cluster{dbl[], dbl[]}[])
        n533 = Select(t=1 ("index (row)"), s=w1147, f=0 ("index (row)")) -> (s? t:f=w1144:i32)
        n534 = Index Array(array=w1150, index (row)=w1144) -> (element=w1149:dbl[])  [unwired: 1 in]
        n535 = Array Max & Min(array=w1149) -> (max value=w1148:dbl)  [unwired: 3 out]
        n536 = global read "Results_plotter_Global.vi" "Point info"() -> (w1155:T13)
        n537 = global read "Results_plotter_Global.vi" "Legend"() -> (w1156:string[])
        n538 = Greater?(x=w1148, y=2680560000.0) -> (0:w1152:bool)
        n539 = case shown="False" w1152 {
          tunnel: [w1167 u8 7 ("X Scale.Format & Precision:Precision")] -> w1151
          tunnel: w1148 -> [w1173 _]
          frame False {
            n540 = Absolute Value(x=w1173) -> (abs(x)=w1166:dbl)
            n541 = In Range and Coerce(upper limit=100000.0 ("y"), x=w1166, lower limit=0.0001) -> (In Range?=w1170:bool)  [unwired: 1 out]
            n542 = Select(t=u8 0 ("f"), s=w1170, f=u8 1) -> (s? t:f=w1167:u8)
          }
          frame True {
          }
        }
        n543 = local write "Warning!"("") -> ()
        n544 = for {
          tunnel: w1156 -> [w1193] mode=indexing
          tunnel: w1155 -> [w1190] mode=indexing
          tunnel: [w1191] -> w1160
          i -> [w1191]
          n545 = call "Abbreviate_string.vi"("Input String"=w1193, "Max String Length"=50) -> ("Output String"=w1184:string)
          n546 = String Length(string=w1184) -> (length=w1187:i32)
          n547 = Subtract(x=w1187, y=2) -> (x-y=w1185:i32)
          n548 = String Subset(string=w1184, length (rest)=w1185) -> (substring=w1183:string)  [unwired: 1 out]
          n549 = Unbundle By Name(w1190) -> ("Point Style"=w1189:u8, "Fill/Pt. Color"=w1188:u32)
          n550 = call "Fast_string_Replace.vi"("Replace match with:"="_", "Input String"=w1183, "regular expression"=" ") -> ("Output String"=w1182:string)  [unwired: 1 in, 1 out]
          n551 = property on="XY Plot" class="XYGraph (strict)"("Active Plot"=w1191, "Plot.Plot Name"=w1182, "Plot.Point Style"=w1189, "Plot.Fill/Point Color"=w1188, "Plot.Plot Color"=w1188) -> ()  [unwired: 2 in, 2 out]
        }
        n552 = Increment(x=w1160) -> (x+1=w1159:i32)
        n553 = property on="XY Plot" class="XYGraph (strict)"("X Scale.Format & Precision:Format"=w1151) -> ()  [unwired: 2 in, 2 out]
        n554 = for {
          N: 10 -> [_]
          tunnel: w1159 -> [w1178]
          i -> [w1179]
          w1175 = u32 0
          n555 = Add(x=w1178, y=w1179) -> (x+y=w1177:i32)
          n556 = property on="XY Plot" class="XYGraph (strict)"("Active Plot"=w1177, "Plot.Plot Name"="" ("Write Attribute"), "Plot.Plot Color"=w1175, "Plot.Fill/Point Color"=w1175) -> ()  [unwired: 2 in, 2 out]
        }
      }
      frame "Add Axis names" {
        n557 = local read "Multi Ordinate"() -> (w1208:i32[])
        n558 = for {
          tunnel: w1208 -> [w1225] mode=indexing
          shift-right: [w1222] -> w1201
          shift-left: "" -> [w1221]
          tunnel: w1209 -> [w1224]
          tunnel: [w1217] -> w1200
          i -> [w1217]
          n559 = Index Array(array=w1224, index=w1225) -> (element=w1223:string)
          n560 = String Length(string=w1221) -> (length=w1220:i32)
          n561 = Less?(x=w1220, y=40) -> (x < y?=w1218:bool)
          n562 = case shown="True" w1218 {
            tunnel: w1223 -> [_ w1230]
            tunnel: [w1226 w1229] -> w1222
            tunnel: w1221 -> [w1226 w1227]
            frame False {
            }
            frame True {
              n563 = Concatenate Strings(w1227, w1230, "   ") -> (w1229:string)
            }
          }
        }
        n564 = Greater Than 0?(x=w1200) -> (x > 0?=w1198:bool)
        n565 = local read "Transpose"() -> (w1211:bool)
        n566 = local read "Absisca"() -> (w1212:u16)
        n567 = Index Array(array=w1209, index=w1212) -> (element=w1210:string)
        n568 = String Length(string=w1201) -> (length=w1204:i32)
        n569 = Empty String/Path?(string/path="Ordinate Name") -> (empty?=w1199:bool)
        n570 = Subtract(x=w1204, y=3) -> (x-y=w1202:i32)
        n571 = Compound Arithmetic op=AND(invert w1199, w1198) -> (w1197:bool)
        n572 = String Subset(string=w1201, length (rest)=w1202) -> (substring=w1196:string)  [unwired: 1 out]
        n573 = Select(t="Ordinate Name", s=w1197, f=w1196) -> (s? t:f=w1194:string)
        n574 = case shown="False" w1211 {
          tunnel: [w1231 w1234] -> w1207
          tunnel: w1194 -> [w1232 w1234]
          tunnel: [w1232 w1233] -> w1206
          tunnel: w1210 -> [w1231 w1233]
          frame False {
          }
          frame True {
          }
        }
        n575 = global write "Results_plotter_Global.vi" "X Axis Name"(w1207) -> ()
        n576 = global write "Results_plotter_Global.vi" "Y Axis Name"(w1206) -> ()
        n577 = global write "Results_plotter_Global.vi" "Value plotted Name"(w1194) -> ()
        n578 = property on="XY Plot" class="XYGraph (strict)"("X Scale.Name Label.Text"=w1207, "Y Scale.Name Label.Text"=w1206) -> ()  [unwired: 2 in, 2 out]
      }
      frame "Intensity plot" {
        # "Max"
        # "Min"
        n579 = global read "Results_plotter_Global.vi" "XY Graph Cluster"() -> (w1235:cluster{dbl[], dbl[]}[])
        n580 = local read "Tolerances"() -> (w1240:dbl[])
        n581 = local read "Absisca"() -> (w1239:u16)
        n582 = local read "Transpose"() -> (w1236:bool)
        n583 = stacked-sequence {
          seq-local: [w1253 _ _ _ _ _ _ _ _ _ _ _ _] -> [_ _ _ w1318 w1325 _ w1350 _ _ _ _ _ _]
          seq-local: [_ w1269 _ _ _ _ _ _ _ _ _ _ _] -> [_ _ _ _ w1324 _ w1349 _ _ _ _ _ _]
          seq-local: [_ _ w1301 _ _ _ _ _ _ _ _ _ _] -> [_ _ _ _ _ _ w1358 _ _ _ _ _ _]
          seq-local: [_ _ _ _ _ _ w1360 _ _ _ _ _ _] -> [_ _ _ _ _ _ _ _ w1384 _ _ _ _]
          seq-local: [_ _ _ _ _ _ w1359 _ _ _ _ _ _] -> [_ _ _ _ _ _ _ _ w1385 _ _ _ _]
          seq-local: [_ w1265 _ _ _ _ _ _ _ _ _ _ _] -> [_ _ _ _ _ _ _ _ _ w1449 _ _ _]
          seq-local: [_ _ _ w1316 _ _ _ _ _ _ _ _ _] -> [_ _ _ _ w1323 _ w1354 _ _ _ _ _ _]
          seq-local: [_ _ _ _ _ _ _ _ _ _ _ w1475 _] -> [_ _ _ _ _ _ _ _ _ _ _ _ w1525]
          seq-local: [_ _ _ _ _ _ _ _ _ _ _ w1474 _] -> [_ _ _ _ _ _ _ _ _ _ _ _ w1526]
          seq-local: [_ _ _ w1315 _ _ _ _ _ _ _ _ _] -> [_ _ _ _ _ w1338 _ _ _ _ _ _ _]
          seq-local: [_ _ _ _ _ _ _ _ _ _ _ w1472 _] -> [_ _ _ _ _ _ _ _ _ _ _ _ w1518]
          tunnel: [_ _ _ TRUE _ _ _ _ _ _ _ _ _] -> w1246
          tunnel: [_ _ _ _ _ _ _ _ _ _ _ _ "Analyse Plot Space"] -> w1245
          tunnel: w1243 -> [w1250 _ _ _ _ _ _ _ _ _ _ _ _]
          tunnel: w1244 -> [w1251 _ w1302 _ _ _ _ _ _ w1430 _ _ _]
          tunnel: [w1251 _ _ _ _ _ _ _ _ _ _ _ _] -> w1242
          tunnel: [w1250 _ _ _ _ _ _ _ _ _ _ _ _] -> w1241
          tunnel: w1240 -> [w1255 _ _ _ _ _ _ _ _ _ _ _ _]
          tunnel: w1235 -> [w1254 _ _ w1320 _ _ _ _ _ _ _ _ _]
          tunnel: w1239 -> [w1252 _ _ _ _ _ _ _ _ w1446 _ _ _]
          tunnel: w1236 -> [w1249 _ _ w1317 _ _ w1362 _ _ w1444 _ _ _]
          tunnel: [_ w1270 _ _ _ _ _ _ _ _ _ _ _] -> w1238
          tunnel: w1237 -> [_ w1270 _ _ _ _ _ _ _ w1431 _ _ _]
          frame #0 {
            n584 = Not(x=w1249) -> (.not. x?=w1248:bool)
            n585 = for {
              tunnel: w1254 -> [w1264] mode=indexing
              tunnel: w1248 -> [w1261]
              shift-right: [w1259] -> w1256
              shift-left: dbl[] [] -> [w1260]
              n586 = Unbundle(w1264) -> (w1263:dbl[], w1262:dbl[])
              n587 = Select(t=w1263, s=w1261, f=w1262) -> (s? t:f=w1258:dbl[])
              n588 = Build Array (concatenate)(w1260, w1258) -> (w1259:dbl[])
            }
            n589 = Index Array(array=w1255, index=w1252) -> (element=w1247:dbl)
            n590 = call "Numeric_bins.vi"("Values"=w1256, "Tolerance"=w1247) -> ("Bin Centres"=w1253:dbl[])  [unwired: 2 out]
          }
          frame #1 {
            n591 = local read "Filter Bins 2"() -> (w1271:i32[])
            n592 = local read "Filter Bins 1"() -> (w1273:i32[])
            n593 = Array Size(array=w1271) -> (size(s)=w1275:i32)
            n594 = Array Size(array=w1273) -> (size(s)=w1276:i32)
            n595 = Greater?(x=w1276, y=w1275) -> (0:w1274:bool)
            n596 = case shown="True" w1274 {
              tunnel: w1273 -> [_ w1298]
              tunnel: [w1294 w1298] -> w1272
              tunnel: [w1295 w1297] -> w1267
              tunnel: w1271 -> [w1294 _]
              tunnel: [1 0] -> w1265
              frame False {
                n597 = property on="Filter Bins 2" class="LstBox (strict)"() -> ("Item Names"=w1295:string[])  [unwired: 2 in, 2 out]
              }
              frame True {
                n598 = property on="Filter Bins 1" class="LstBox (strict)"() -> ("Item Names"=w1297:string[])  [unwired: 2 in, 2 out]
              }
            }
            n599 = Array Size(array=w1267) -> (size(s)=w1266:i32)
            n600 = for {
              tunnel: w1272 -> [w1281] mode=indexing
              tunnel: w1267 -> [w1287]
              shift-right: [w1284] -> w1269
              shift-left: dbl[] [] -> [w1285]
              tunnel: w1266 -> [w1280]
              n601 = Index Array(array=w1287, index=w1281) -> (element=w1283:string)
              n602 = Less?(x=w1281, y=w1280) -> (x < y?=w1279:bool)
              n603 = Match Pattern(string=w1283, regular expression=" (0)") -> (offset past match=w1282:i32)  [unwired: 4 out]
              n604 = Less Than 0?(x=w1282) -> (x < 0?=w1278:bool)
              n605 = And(x=w1278, y=w1279) -> (x .and. y?=w1277:bool)
              n606 = case shown="True" w1277 {
                tunnel: w1285 -> [w1288 w1292]
                tunnel: [w1288 w1291] -> w1284
                tunnel: w1283 -> [_ w1290]
                frame False {
                }
                frame True {
                  n607 = Fract/Exp String To Number(string=w1290) -> (number=w1289:dbl)  [unwired: 4 out]
                  n608 = Build Array (concatenate)(w1292, w1289) -> (w1291:dbl[])
                }
              }
            }
          }
          frame #2 {
            n609 = local read "Template"() -> (w1300:path)
            n610 = call "Valid_Path.vi"("Filename"=w1300) -> ("Valid Path?"=w1299:bool)
            n611 = case shown="True" w1299 {
              tunnel: w1300 -> [_ w1312]
              tunnel: w1302 -> [_ w1311]
              tunnel: [nan w1308] -> w1301
              frame False {
              }
              frame True {
                n612 = local read "Multi Ordinate"() -> (w1307:i32[])
                n613 = call "Read_Write_Template.vi"("Template File"=w1312, "Mode"=Global_mode."Read Global", "Channel names In"=w1311, "Data type"="Minimum Value") -> ("1D Info Out"=w1310:string[])  [unwired: 4 in, 7 out]
                n614 = Index Array(array=w1307, index=0 ("Index")) -> (element=w1306:i32)
                n615 = Index Array(array=w1310, index=w1306) -> (element=w1309:string)
                n616 = Fract/Exp String To Number(string=w1309, default (0 dbl)=nan) -> (number=w1308:dbl)  [unwired: 3 out]
              }
            }
          }
          frame #3 {
            n617 = call "Grid_Data.vi"("Transpose"=w1317, "XY Graph"=w1320, "Bin Centres"=w1318) -> ("No of Duplicates"=w1315:i32, "Grided data"=w1316:dbl[][])
          }
          frame #4 {
            n618 = for {
              tunnel: w1325 -> [w1330]
              tunnel: w1324 -> [w1329] mode=indexing
              tunnel: w1323 -> [w1328] mode=indexing
              shift-right: [w1326] -> w1321
              shift-left: dbl[][] [] -> [w1327]
              n619 = for {
                tunnel: w1330 -> [w1336] mode=indexing
                tunnel: w1329 -> [w1331]
                tunnel: w1328 -> [w1335] mode=indexing
                shift-right: [w1332] -> w1326
                shift-left: w1327 -> [w1334]
                n620 = Build Array(w1336, w1331, w1335) -> (w1333:dbl[])
                n621 = Build Array (concatenate)(w1334, w1333) -> (w1332:dbl[][])
              }
            }
            n622 = global write "Results_plotter_Global.vi" "Intensity Plot data in rows"(w1321) -> ()
          }
          frame #5 {
            n623 = case shown="1, Default" w1338 {
              tunnel: w1338 -> [_ w1342]
              tunnel: ["" w1340] -> w1337
              frame 0 {
              }
              frame 1, Default {
                n624 = Format Into String(format string="The Intensity Plot has %d duplicate points which have been averaged together.", w1342) -> (resulting string=w1340:string)  [unwired: 2 in, 1 out]
              }
            }
            "Warning!" <- w1337
          }
          frame #6 {
            n625 = call "Insert_extra_rows_and_col.vi"("Row Values In"=w1349, "Additional Row Values"="Additional X Values", "Column Values In"=w1350, "Data In"=w1354, "Additional Column Values"="Additional Y Values") -> ("Row Values Out"=w1351:dbl[], "Column Values Out"=w1352:dbl[], "Data Out"=w1353:dbl[][])  [unwired: 2 out]
            n626 = Select(t="Resolution", s="Plot Resolution", f=0.0) -> (s? t:f=w1344:dbl)
            n627 = call "2D_interpolation.vi"("X Axis Current"=w1352, "Min Z Value In"=w1358, "Y axis Current"=w1351, "Bkgnd Value"="Bkgnd Value", "Plot In"=w1353, "Increment Value"=w1344, "Transpose"=w1362, "Point Size"="Point Size") -> ("min Z value"=w1360:dbl, "max Z value"=w1359:dbl, "Increment Value Out"=w1348:dbl, "Plot Out"=→"Intensity Graph":dbl[][])  [unwired: 4 out]
            n628 = local write "Resolution"(w1348) -> ()
          }
          frame #7 {
            n629 = global read "Results_plotter_Global.vi" "X Scale"() -> (w1370:cluster{"Xo":dbl, "delta X":dbl})
            n630 = global read "Results_plotter_Global.vi" "Y Scale"() -> (w1366:cluster{"Xo":dbl, "delta X":dbl})
            n631 = global read "Results_plotter_Global.vi" "X Max"() -> (w1368:dbl)
            n632 = global read "Results_plotter_Global.vi" "Y Max"() -> (w1367:dbl)
            n633 = Unbundle By Name(w1366) -> ("Xo"=w1365:dbl)
            n634 = Unbundle By Name(w1370) -> ("Xo"=w1369:dbl)
            n635 = Subtract(x=w1367, y=w1365) -> (x-y=w1371:dbl)
            n636 = Subtract(x=w1368, y=w1369) -> (x-y=w1380:dbl)
            n637 = Greater?(x=w1380, y=5.0) -> (0:w1378:bool)
            n638 = Greater?(x=w1371, y=5.0) -> (0:w1373:bool)
            n639 = Select(t=u8 0 ("Write Attribute"), s=w1378, f=u8 3) -> (s? t:f=w1364:u8)
            n640 = Select(t=u8 0 ("Write Attribute"), s=w1373, f=u8 3) -> (s? t:f=w1363:u8)
            n641 = property on="Intensity Graph" class="IntGraph (strict)"("X Scale.Offset and Multiplier"=w1370, "X Scale.Range:Maximum"=w1368, "Y Scale.Offset and Multiplier"=w1366, "Y Scale.Range:Maximum"=w1367, "X Scale.Format & Precision:Precision"=w1364, "Y Scale.Format & Precision:Precision"=w1363) -> ()  [unwired: 2 in, 2 out]
          }
          frame #8 {
            n642 = Greater Than 0?(x=w1385) -> (x > 0?=w1382:bool)
            n643 = Less Than 0?(x=w1384) -> (x < 0?=w1383:bool)
            n644 = And(x=w1382, y=w1383) -> (x .and. y?=w1381:bool)
            n645 = case shown="True" w1381 {
              tunnel: w1385 -> [w1414 w1428]
              tunnel: [w1422 w1426] -> w1387
              tunnel: w1384 -> [w1410 w1423]
              frame True {
                (unwired) u32 3743
                (unwired) u32 16721152
                n646 = Absolute Value(x=w1410) -> (abs(x)=w1409:dbl)
                n647 = Absolute Value(x=w1414) -> (abs(x)=w1416:dbl)
                n648 = Absolute Value(x=w1410) -> (abs(x)=w1417:dbl)
                n649 = Max & Min(x=w1416, y=w1417) -> (max(x,y)=w1412:dbl)  [unwired: 1 out]
                n650 = Divide(x=w1409, y=w1412) -> (x/y=w1403:dbl)
                n651 = Subtract(x=1.0, y=w1403) -> (x-y=w1402:dbl)
                n652 = Multiply(x=w1402, y=u32 255) -> (x*y=w1408:dbl)
                n653 = To Unsigned Long Integer(number=w1408) -> (unsigned 32bit integer=w1392:u32)
                n654 = Multiply(x=w1392, y=u32 256) -> (x*y=w1394:u32)
                n655 = Multiply(x=w1392, y=u32 65536) -> (x*y=w1391:u32)
                n656 = Compound Arithmetic op=ADD(w1391, w1394, u32 255) -> (w1390:u32)
                n657 = Bundle("min Z value"=w1410, w1390) -> (w1419:cluster{"min Z value":dbl, u32})  [unwired: 1 out]
                n658 = Divide(x=w1414, y=w1412) -> (x/y=w1407:dbl)
                n659 = Bundle("max Z value"=0.0, u32 16777215) -> (w1418:cluster{"max Z value":dbl, u32})  [unwired: 1 out]
                n660 = Subtract(x=1.0, y=w1407) -> (x-y=w1405:dbl)
                n661 = Multiply(x=w1405, y=u32 255) -> (x*y=w1401:dbl)
                n662 = To Unsigned Long Integer(number=w1401) -> (unsigned 32bit integer=w1388:u32)
                n663 = Multiply(x=w1388, y=u32 256) -> (x*y=w1398:u32)
                n664 = Compound Arithmetic op=ADD(w1388, w1398, u32 16711680) -> (w1389:u32)
                n665 = Bundle("max Z value"=w1414, w1389) -> (w1421:cluster{"max Z value":dbl, u32})  [unwired: 1 out]
                n666 = Build Array(w1421, w1419) -> (w1420:cluster{"min Z value":dbl, u32}[])
                n667 = Build Array (concatenate)(w1420, w1418) -> (w1422:cluster{"max Z value":dbl, u32}[])
              }
              frame False {
                n668 = Bundle("max Z value"=w1428, u32 16721152) -> (w1425:cluster{"max Z value":dbl, u32})  [unwired: 1 out]
                n669 = Bundle("min Z value"=w1423, u32 3743) -> (w1424:cluster{"min Z value":dbl, u32})  [unwired: 1 out]
                n670 = Build Array(w1425, w1424) -> (w1426:cluster{"min Z value":dbl, u32}[])
              }
            }
            n671 = property on="Intensity Graph" class="IntGraph (strict)"("Ignore Array"=FALSE ("Write Attribute"), "Z Scale.Marker Values[]"=w1387) -> ()  [unwired: 2 in, 2 out]
          }
          frame #9 {
            n672 = local read "Filter Array"() -> (w1448:u16[])
            n673 = Index Array(array=w1448, index=w1449) -> (element=w1447:u16)
            n674 = Decrement(x=w1447) -> (x-1=w1445:u16)
            n675 = local read "Multi Ordinate"() -> (w1435:i32[])
            n676 = Index Array(array=w1431, index=w1445) -> (element=w1439:string)
            n677 = Index Array(array=w1431, index=w1446) -> (element=w1438:string)
            n678 = case shown="False" w1444 {
              tunnel: [w1451 w1453] -> w1437
              tunnel: w1439 -> [w1451 w1452]
              tunnel: w1438 -> [w1450 w1453]
              tunnel: [w1450 w1452] -> w1436
              frame False {
              }
              frame True {
              }
            }
            n679 = Index Array(array=w1435, index=0) -> (element=w1433:i32)
            n680 = Index Array(array=w1430, index=w1433) -> (element=w1432:string)
            n681 = global write "Results_plotter_Global.vi" "Value plotted Name"(w1432) -> ()
            n682 = property on="Intensity Graph" class="IntGraph (strict)"("X Scale.Name Label.Text"=w1436, "Y Scale.Name Label.Text"=w1437) -> ()  [unwired: 2 in, 2 out]
            n683 = global write "Results_plotter_Global.vi" "Y Axis Name"(w1436) -> ()
            n684 = global write "Results_plotter_Global.vi" "X Axis Name"(w1437) -> ()
            n685 = Format Into String(format string="Add %s values", w1439) -> (resulting string=→"First Add label":string)  [unwired: 2 in, 1 out]
            n686 = Format Into String(format string="Add %s values", w1438) -> (resulting string=→"2nd Add label":string)  [unwired: 2 in, 1 out]
          }
          frame #10 {
            n687 = property on="Intensity Graph" class="IntGraph (strict)"() -> ("Color Table"=w1455:u32[])  [unwired: 2 in, 2 out]
            n688 = Increment(x="No of Contours") -> (x+1=w1456:i32)
            n689 = Divide(x=255, y=w1456) -> (x/y=w1460:dbl)
            n690 = To Long Integer(number=w1460) -> (32bit integer=w1459:i32)
            n691 = for {
              tunnel: w1459 -> [w1468]
              tunnel: [w1465] -> w1454 mode=indexing
              tunnel: w1455 -> [w1464] mode=indexing
              tunnel: u32 0 -> [w1463]
              i -> [w1469]
              n692 = Increment(x=w1469) -> (x+1=w1466:i32)
              n693 = Quotient & Remainder(x=w1466, y=w1468) -> (x-y*floor(x/y)=w1467:i32)  [unwired: 1 out]
              n694 = case shown="0" w1467 {
                tunnel: [w1470 w1471] -> w1465
                tunnel: w1464 -> [_ w1471]
                tunnel: w1463 -> [w1470 _]
                frame 0 {
                }
                frame 1, Default {
                }
              }
            }
            n695 = property on="Intensity Graph" class="IntGraph (strict)"("Ignore Array"=TRUE ("Write Attribute"), "Color Table"=w1454) -> ()  [unwired: 2 in, 2 out]
          }
          frame #11 {
            n696 = global read "Results_plotter_Global.vi" "Raw Interpolation"() -> (w1473:dbl[][])
            n697 = Add Array Elements(numeric array=w1473) -> (sum=w1472:dbl)
            n698 = Array Size(array=w1473) -> (size(s)=w1483:i32[])
            n699 = Decrement(x=w1483) -> (x-1=w1481:i32[])
            n700 = Index Array(array=w1481, index=0) -> (element=w1482:i32)
            n701 = Index Array(array=w1481, index=1) -> (element=w1478:i32)
            n702 = for {
              N: w1482 -> [_]
              tunnel: w1473 -> [w1491]
              tunnel: w1478 -> [w1490]
              shift-right: [w1486] -> w1475
              shift-left: 0.0 -> [w1487]
              shift-right: [w1485] -> w1474
              shift-left: 0 -> [w1484]
              i -> [w1489]
              n703 = Increment(x=w1489) -> (x+1=w1488:i32)
              n704 = for {
                N: w1490 -> [_]
                tunnel: w1491 -> [w1500]
                tunnel: w1489 -> [w1505]
                tunnel: w1488 -> [w1503]
                shift-right: [w1496] -> w1486
                shift-left: w1487 -> [w1495]
                shift-right: [w1492] -> w1485
                shift-left: w1484 -> [w1493]
                i -> [w1504]
                n705 = Increment(x=w1504) -> (x+1=w1502:i32)
                n706 = Index Array(array=w1500, index (row)=w1505, index (col)=w1502) -> (element=w1501:dbl)
                n707 = Index Array(array=w1500, index (row)=w1503, index (col)=w1502) -> (element=w1498:dbl)
                n708 = Index Array(array=w1500, index (row)=w1505, index (col)=w1504) -> (element=w1506:dbl)
                n709 = Index Array(array=w1500, index (row)=w1503, index (col)=w1504) -> (element=w1499:dbl)
                n710 = Compound Arithmetic op=ADD(w1506, w1501, w1499, w1498) -> (w1494:dbl)
                n711 = Not A Number/Path/Refnum?(number/path/refnum=w1494) -> (NaN/Path/Refnum?=w1497:bool)
                n712 = case shown="False" w1497 {
                  tunnel: [w1510 w1514] -> w1496
                  tunnel: w1495 -> [w1512 w1514]
                  tunnel: w1494 -> [w1511 _]
                  tunnel: [w1509 w1513] -> w1492
                  tunnel: w1493 -> [w1508 w1513]
                  frame False {
                    n713 = Add(x=w1511, y=w1512) -> (x+y=w1510:dbl)
                    n714 = Add(x=1, y=w1508) -> (x+y=w1509:i32)
                  }
                  frame True {
                  }
                }
              }
            }
          }
          frame #12 {
            n715 = local read "Resolution"() -> (w1527:dbl)
            n716 = Divide(x=w1525, y=4.0) -> (x/y=w1523:dbl)
            n717 = Multiply(x=w1527, y=w1527) -> (x*y=w1519:dbl)
            n718 = Multiply(x=w1519, y=w1518) -> ()  [unwired: 1 out]
            n719 = Multiply(x=w1519, y=w1526) -> (x*y=w1520:dbl)
            "Surface Area" <- w1520
            n720 = Multiply(x=w1519, y=w1523) -> (x*y=w1516:dbl)
            "Surface Integral" <- w1516
            n721 = global write "Results_plotter_Global.vi" "Surface Area"(w1520) -> ()
            n722 = global write "Results_plotter_Global.vi" "Surface Integral"(w1516) -> ()
            n723 = Divide(x=16666667, y=w1516) -> (x/y=→"Uadvec":dbl)
            n724 = Divide(x=w1516, y=w1520) -> (x/y=→"Surface Average":dbl)
          }
        }
      }
      frame "Analyse Plot Space" {
        n725 = case shown="True" "Show Plot Space Analysis" {
          tunnel: w1532 -> [_ w1542]
          tunnel: w1529 -> [_ w1541]
          frame False {
          }
          frame True {
            w1538 = TRUE  # Summarise All
            n726 = global read "Results_plotter_Global.vi" "Plot Index values"() -> (w1536:dbl[][])
            n727 = Index Array(array=w1536, index (row)=2) -> (element=w1535:dbl[])  [unwired: 1 in]
            n728 = To Long Integer(number=w1535) -> (32bit integer=w1534:i32[])
            n729 = for {
              tunnel: w1534 -> [w1545] mode=indexing
              tunnel: w1542 -> [w1544]
              tunnel: [w1543] -> w1539 mode=indexing
              n730 = Index Array(array=w1544, index (row)=w1545) -> (element=w1543:string[])  [unwired: 1 in]
            }
            n731 = call "Summarise.vi"("Channel Names"=w1541, "Data"=w1539, "Summarise All"=w1538) -> ("Summary"=w1540:string[][])  [unwired: 2 in]
            n732 = call "Plot_Space_Analysis.vi"("Table"=w1540) -> ()
          }
        }
      }
      frame "Vector Plot" {
        n733 = flat-sequence {
          tunnel: w1550 -> [w1552]
          tunnel: w1548 -> [w1551]
          frame #0 {
            n734 = local read "Template"() -> (w1553:path)
            n735 = call "Vector_Plotting.vi"("Template Filename"=w1553, "Data"=w1551, "Channel Names"=w1552) -> ()  [unwired: 1 out]
          }
          frame #1 {
            n736 = local write "Vector Plot?"(FALSE ("Vector Plot?")) -> ()
          }
        }
      }
      frame "What to do next?" {
        n737 = local read "Warning!"() -> (w1563:string)
        n738 = Empty String/Path?(string/path=w1563) -> (empty?=w1562:bool)
        n739 = Not(x=w1562) -> (.not. x?=w1561:bool)
        n740 = property on="Warning!" class="Str" props=["Visible", "Blinking", "Caption"]("Visible"=w1561, "Blinking"=w1561) -> ()  [unwired: 2 in, 3 out]
        n741 = case shown="False" "Add results file" {
          tunnel: [w1585 "More files options"] -> w1566
          tunnel: "Add results file" -> [_ _]
          tunnel: "Edit Template File" -> [w1576 _]
          frame False {
            n742 = Select(t="Edit template file", s=w1576, f="What to do next 2nd?") -> (s? t:f=w1574:string)
            n743 = Or(x="Save Plot data", y="Save Surface Fit") -> (x .or. y?=w1578:bool)
            n744 = Select(t="Save Plot Data", s=w1578, f=w1574) -> (s? t:f=w1581:string)
            n745 = Select(t="Create Plot summary", s="Save Plot as jpg", f=w1581) -> (s? t:f=w1572:string)
            n746 = Select(t="Save Data in Rows", s="Save Data in Rows", f=w1572) -> (s? t:f=w1585:string)
          }
          frame True {
            n747 = local write "Add results file"(FALSE) -> ()
          }
        }
        n748 = Select(t="End", s="stop", f=w1566) -> (s? t:f=w1557:string)
        n749 = Select(t="Vector Plot", s="Vector Plot?", f=w1557) -> (s? t:f=w1556:string)
      }
      frame "What to do next 2nd?" {
        n750 = local read "Empty"() -> (w1609:bool)
        n751 = local read "Last used Template"() -> (w1597:path)
        n752 = local read "Template"() -> (w1589:path)
        n753 = Select(t="Empty Results file array", s=w1609, f="What to do next 3rd?") -> (s? t:f=w1592:string)
        n754 = global write "Results_plotter_Global.vi" "Template"(w1589) -> ()
        n755 = Not Equal?(x=w1597, y=w1589) -> (x != y?=w1596:bool)
        n756 = local read "Selected Row"() -> (w1588:i32)
        n757 = Select(t="What type of row averaging?", s="Save Averaged rows", f=w1592) -> (s? t:f=w1604:string)
        n758 = case shown="True" "Delete Plotted data from file" {
          tunnel: [w1639 "Full Res file manipulator" ("t")] -> w1602
          tunnel: w1604 -> [w1639 _]
          frame False {
          }
          frame True {
            n759 = local write "Plotted rows only?"(TRUE ("Save Plotted rows only?")) -> ()
            n760 = local write "Mode"(Plotter_Mode."Delete unwanted rows" ("Mode")) -> ()
          }
        }
        n761 = case shown="True" "Add /Edit metadata" {
          tunnel: [w1614 w1631] -> w1594
          tunnel: w1602 -> [w1615 w1632]
          tunnel: w1600 -> [_ w1630]
          tunnel: "Reload Files" -> [w1616 _]
          tunnel: [string[] [] ("New Chs Out") w1624] -> w1591
          tunnel: [string[][] [] w1623] -> w1590
          tunnel: w1588 -> [_ w1619]
          frame False {
            n762 = Select(t="Initialise", s=w1616, f=w1615) -> (s? t:f=w1614:string)
          }
          frame True {
            n763 = local read "Result files to read"() -> (w1625:path[])
            n764 = call "Edit_Channel_Panel.vi"("All Channel names"=w1630, "Result files to read"=w1625, "Selected Row"=w1619) -> ("New Values Out"=w1638:string[], "New Chs Out"=w1624:string[], "Cancel Out"=w1627:bool, "Edit Raw Data Header Info Out"=w1621:bool, "Plotted rows only?"=w1637:bool, "Selected Row?"=→"Selected Row?":bool, "Edit Raw data files?"=→"Edit Raw DF?":bool, "Raw data files in Orig Positions?"=→"Raw DF in Orig Pos?":bool, "Mode"=w1635:T4)  [unwired: 4 out]
            "Edit Raw Data Header Info" <- w1621
            n765 = Array Size(array=w1624) -> (size(s)=w1634:i32)
            n766 = Build Array(w1638) -> (w1623:string[][])
            n767 = Greater Than 0?(x=w1634) -> (x > 0?=w1622:bool)
            n768 = local write "Add /Edit metadata"(FALSE ("Add /Edit metadata")) -> ()
            n769 = local write "Plotted rows only?"(w1637) -> ()
            n770 = Or(x=w1621, y=w1622) -> (x .or. y?=w1620:bool)
            n771 = local write "Mode"(w1635) -> ()
            n772 = Compound Arithmetic op=AND(invert w1627, w1620) -> (w1626:bool)
            n773 = Select(t="Full Res file manipulator", s=w1626, f=w1632) -> (s? t:f=w1631:string)
          }
        }
        n774 = global write "Results_plotter_Global.vi" "New Chs In"(w1591) -> ()
        n775 = global write "Results_plotter_Global.vi" "New Values In"(w1590) -> ()
        n776 = Select(t="Initialise", s=w1596, f=w1594) -> (s? t:f=w1593:string)
      }
      frame "What to do next 3rd?" {
        n777 = local read "Show Results Space Analysis"() -> (w1654:bool)
        n778 = local read "Show Plot Space Analysis"() -> (w1653:bool)
        n779 = while {
          shift-right: [w1677] -> _
          shift-left: _ -> [w1676]
          shift-left: _ -> [w1675]
          shift-left: _ -> [w1674]
          tunnel: w1654 -> [w1677]
          shift-right: [w1682] -> _
          shift-left: _ -> [w1681]
          shift-left: _ -> [w1680]
          shift-left: _ -> [w1679]
          tunnel: w1653 -> [w1682]
          tunnel: [w1678] -> w1652
          tunnel: [w1673] -> w1651
          stop <- TRUE stop-if-true
          n780 = Compound Arithmetic op=AND(w1677, w1676, w1675, w1674) -> (w1673:bool)
          n781 = Compound Arithmetic op=AND(w1682, w1681, w1680, w1679) -> (w1678:bool)
        }
        n782 = Select(t="Run Calculation Routine", s="Calculate new metadata", f="Time to save setup?") -> (s? t:f=w1660:string)
        n783 = case shown="True" w1652 {
          frame False {
          }
          frame True {
            n784 = Open VI Reference(vi path="Plot_Space_Analysis.vi" ("VI path")) -> (vi reference=w1694:refnum<vi>, error out=w1693:errorcluster)  [unwired: 1 in, 4 out]
            n785 = property class="VI"(reference=w1694, error in=w1693) -> (reference out=w1692:refnum<vi>, error out=w1691:errorcluster, "Front Panel Window:Open"=w1689:bool)
            n786 = local write "Show Plot Space Analysis"(w1689) -> ()
            n787 = Close Reference(reference=w1692, error in (no error)=w1691) -> ()  [unwired: 1 out]
          }
        }
        n788 = case shown="True" w1651 {
          frame False {
          }
          frame True {
            n789 = Open VI Reference(vi path="Results_Space_Analysis.vi" ("VI path")) -> (vi reference=w1688:refnum<vi>, error out=w1687:errorcluster)  [unwired: 1 in, 4 out]
            n790 = property class="VI"(reference=w1688, error in=w1687) -> (reference out=w1686:refnum<vi>, error out=w1685:errorcluster, "Front Panel Window:Open"=w1683:bool)
            n791 = local write "Show Results Space Analysis"(w1683) -> ()
            n792 = Close Reference(reference=w1686, error in (no error)=w1685) -> ()  [unwired: 1 out]
          }
        }
        n793 = Select(t="Save Setup", s="Save Setup", f=w1660) -> (s? t:f=w1657:string)
        n794 = Select(t="Choose Setup file", s="Load Setup", f=w1657) -> (s? t:f=w1650:string)
        n795 = Or(x="Kill Point", y="Process Point") -> (x .or. y?=w1647:bool)
        n796 = Select(t="Process cursor point", s=w1647, f=w1650) -> (s? t:f=w1643:string)
        n797 = case shown="False" "Post Process Plotted Data" {
          tunnel: [w1668 "Full Res file manipulator" ("t")] -> w1644
          tunnel: w1643 -> [w1668 _]
          frame False {
          }
          frame True {
            n798 = local write "Plotted rows only?"(TRUE ("Plotted rows only?")) -> ()
            n799 = local write "Mode"(Plotter_Mode."Post Process Plotted Rows" ("Mode")) -> ()
          }
        }
      }
      frame "Time to save setup?" {
        n800 = stacked-sequence {
          seq-local: [w1704 _] -> [_ w1748]
          seq-local: [w1703 _] -> [_ w1747]
          tunnel: [w1712 _] -> w1697
          tunnel: w1696 -> [w1702 _]
          tunnel: [w1701 _] -> w1695
          frame #0 {
            n801 = while {
              shift-right: [w1734] -> _
              shift-left: _ -> [w1732]
              shift-right: [w1721] -> _
              shift-left: _ -> [w1729]
              tunnel: [w1721] -> w1711
              tunnel: [w1720] -> w1710
              shift-right: [w1722] -> _
              shift-left: _ -> [w1728]
              tunnel: [w1726] -> w1705
              tunnel: [w1723] -> w1706
              tunnel: [w1722] -> w1707
              tunnel: [w1719] -> w1703
              tunnel: w1702 -> [w1715]
              tunnel: [w1714] -> w1701
              stop <- FALSE continue-if-true
              n802 = Get Date/Time In Seconds() -> (seconds since 1Jan1904=w1730:timestamp)
              n803 = To Double Precision Float(number=w1730) -> (double precision float=w1733:dbl)
              n804 = Subtract(x=w1733, y=w1732) -> (x-y=w1736:dbl)
              n805 = local read "Show Plot Space Analysis"() -> (w1722:bool)
              n806 = Greater?(x=w1736, y=600.0) -> (0:w1717:bool)
              n807 = local read "Show Results Space Analysis"() -> (w1721:bool)
              n808 = Greater?(x=w1715, y=300) -> (0:w1713:bool)
              n809 = And(x=w1717, y=w1713) -> (x .and. y?=w1716:bool)
              n810 = case shown="False" w1716 {
                tunnel: [w1737 w1746] -> w1734
                tunnel: w1733 -> [w1738 w1746]
                tunnel: w1732 -> [w1739 _]
                tunnel: ["Check modification dates?" "Save Setup"] -> w1725
                tunnel: [TRUE w1743] -> w1714
                tunnel: w1713 -> [w1740 _]
                frame False {
                  n811 = Select(t=w1739, s=w1740, f=w1738) -> (s? t:f=w1737:dbl)
                }
                frame True {
                  n812 = global read "Trav_pos_global.vi" "Estimated Completion time"() -> (w1745:string)
                  n813 = Empty String/Path?(string/path=w1745) -> (empty?=w1743:bool)
                }
              }
              n814 = Not Equal?(x=w1722, y=w1728) -> (x != y?=w1723:bool)
              n815 = Not Equal?(x=w1721, y=w1729) -> (x != y?=w1720:bool)
              n816 = Compound Arithmetic op=AND(invert w1721, w1720) -> (w1719:bool)
              n817 = And(x=w1722, y=w1723) -> (x .and. y?=w1727:bool)
              n818 = Select(t="Analyse Plot Space", s=w1727, f=w1725) -> (s? t:f=w1726:string)
            }
            n819 = Compound Arithmetic op=AND(invert w1707, w1706) -> (w1704:bool)
            n820 = And(x=w1711, y=w1710) -> (x .and. y?=w1709:bool)
            n821 = Select(t="What is present?", s=w1709, f=w1705) -> (s? t:f=w1712:string)
          }
          frame #1 {
            n822 = case shown="True" w1747 {
              frame False {
              }
              frame True {
                n823 = Open VI Reference(vi path="Results_Space_Analysis.vi" ("VI path")) -> (vi reference=w1754:refnum<vi>, error out=w1753:errorcluster)  [unwired: 1 in, 4 out]
                n824 = property class="VI"(reference=w1754, error in=w1753, "Front Panel Window:Open"=FALSE) -> (reference out=w1752:refnum<vi>, error out=w1751:errorcluster)
                n825 = Close Reference(reference=w1752, error in (no error)=w1751) -> ()  [unwired: 1 out]
              }
            }
            n826 = case shown="True" w1748 {
              frame False {
              }
              frame True {
                n827 = Open VI Reference(vi path="Plot_Space_Analysis.vi" ("VI path")) -> (vi reference=w1760:refnum<vi>, error out=w1759:errorcluster)  [unwired: 1 in, 4 out]
                n828 = property class="VI"(reference=w1760, error in=w1759, "Front Panel Window:Open"=FALSE) -> (reference out=w1758:refnum<vi>, error out=w1757:errorcluster)
                n829 = Close Reference(reference=w1758, error in (no error)=w1757) -> ()  [unwired: 1 out]
              }
            }
          }
        }
      }
      frame "Check modification dates?" {
        n830 = while {
          shift-right: [w1780] -> _
          shift-left: _ -> [w1778]
          tunnel: [w1777] -> w1769
          stop <- FALSE continue-if-true
          n831 = Get Date/Time In Seconds() -> (seconds since 1Jan1904=w1775:timestamp)
          n832 = To Double Precision Float(number=w1775) -> (double precision float=w1779:dbl)
          n833 = Subtract(x=w1779, y=w1778) -> (x-y=w1783:dbl)
          n834 = Greater?(x=w1783, y=200.0) -> (0:w1781:bool)
          n835 = case shown="True" w1781 {
            tunnel: [w1785 w1788] -> w1780
            tunnel: w1779 -> [_ w1788]
            tunnel: w1778 -> [w1785 _]
            tunnel: [FALSE w1786] -> w1777
            frame False {
            }
            frame True {
              n836 = global read "Results_plotter_Global.vi" "First Loop"() -> (w1787:bool)
              n837 = Not(x=w1787) -> (.not. x?=w1786:bool)
            }
          }
        }
        n838 = Equal?(x="Tab Control", y=enum32{"Load ", "Plot ", "Save ", "Cursor"}."Cursor" ("Tab Control")) -> (x = y?=w1765:bool)
        n839 = global write "Results_plotter_Global.vi" "First Loop"(FALSE) -> ()
        n840 = Select(t="Read Cursor", s=w1765, f="Ordinate Selector Type") -> (s? t:f=w1763:string)
        n841 = Select(t="Files Modified?", s=w1769, f=w1763) -> (s? t:f=w1768:string)
      }
      frame "Files Modified?" {
        n842 = local read "nRows"() -> (w1792:i32)
        n843 = Less?(x=w1792, y=w1791) -> (x < y?=w1789:bool)
        n844 = case shown="True" w1789 {
          tunnel: [w1798 w1804] -> w1793
          tunnel: "Ordinate Selector Type" -> [w1798 w1799]
          frame False {
          }
          frame True {
            n845 = local read "Result files to read"() -> (w1803:path[])
            n846 = for {
              tunnel: w1803 -> [w1807] mode=indexing
              tunnel: [w1805] -> w1802 mode=indexing
              n847 = call "File_Modified_Since_Check.vi"("Pathname"=w1807, "Just Modified?"=TRUE) -> ("Modified?"=w1805:bool)
            }
            n848 = Or Array Elements(Boolean array=w1802) -> (logical OR=w1801:bool)
            n849 = Select(t="Initialise", s=w1801, f=w1799) -> (s? t:f=w1804:string)
          }
        }
      }
      frame "Read Cursor" {
        n850 = stacked-sequence {
          seq-local: [w1813 _] -> [_ w1848]
          tunnel: ["Ordinate Selector Type" _] -> w1811
          tunnel: [TRUE _] -> w1810
          tunnel: w1809 -> [_ w1847]
          tunnel: w1808 -> [_ w1846]
          frame #0 {
            n851 = property on="XY Plot" class="XYGraph (strict)"() -> ("Cursor.Cursor Position:Cursor X"=w1815:dbl, "Cursor.Cursor Position:Cursor Y"=w1814:dbl)  [unwired: 2 in, 2 out]
            n852 = local read "Transpose"() -> (w1828:bool)
            n853 = global read "Results_plotter_Global.vi" "Plot Index values"() -> (w1821:dbl[][])
            n854 = Index Array(array=w1821, index (row)=1) -> (element=w1819:dbl[])  [unwired: 1 in]
            n855 = Index Array(array=w1821, index (row)=2) -> (element=w1818:dbl[])  [unwired: 1 in]
            n856 = Index Array(array=w1821, index (row)=0) -> (element=w1820:dbl[])  [unwired: 1 in]
            n857 = case shown="True" w1828 {
              tunnel: [w1832 w1834] -> w1827
              tunnel: w1815 -> [w1832 w1833]
              tunnel: [w1831 w1833] -> w1826
              tunnel: w1814 -> [w1831 w1834]
              frame False {
              }
              frame True {
              }
            }
            n858 = for {
              tunnel: w1827 -> [w1843]
              tunnel: w1826 -> [w1842]
              tunnel: [w1837] -> w1825 mode=indexing
              tunnel: w1820 -> [w1836] mode=indexing
              tunnel: w1819 -> [w1835] mode=indexing
              n859 = Subtract(x=w1843, y=w1836) -> (x-y=w1841:dbl)
              n860 = Subtract(x=w1842, y=w1835) -> (x-y=w1840:dbl)
              n861 = Multiply(x=w1841, y=w1841) -> (x*y=w1838:dbl)
              n862 = Multiply(x=w1840, y=w1840) -> (x*y=w1839:dbl)
              n863 = Add(x=w1838, y=w1839) -> (x+y=w1837:dbl)
            }
            n864 = Array Max & Min(array=w1825) -> (min index (indices)=w1817:i32)  [unwired: 3 out]
            n865 = Index Array(array=w1818, index=w1817) -> (element=w1816:dbl)
            n866 = To Long Integer(number=w1816) -> (32bit integer=w1813:i32)
            "Cursor index" <- w1813
          }
          frame #1 {
            n867 = Index Array(array=w1847, index (row)=w1848) -> (element=w1845:string[])  [unwired: 1 in]
            n868 = for {
              tunnel: w1846 -> [w1856] mode=indexing
              tunnel: w1845 -> [w1849] mode=indexing
              tunnel: [w1855] -> w1844 mode=indexing
              n869 = while {
                shift-right: [w1868] -> _
                shift-left: w1849 -> [w1869]
                tunnel: [w1865] -> w1853
                tunnel: [w1864] -> w1851 mode=indexing
                i -> [w1865]
                stop <- w1866 continue-if-true
                n870 = Match Pattern(string=w1869, regular expression=":") -> (before substring=w1864:string, after substring=w1868:string, offset past match=w1867:i32)  [unwired: 2 out]
                n871 = Greater Than 0?(x=w1867) -> (x > 0?=w1866:bool)
              }
              n872 = Greater?(x=w1853, y=2) -> (0:w1852:bool)
              n873 = Reverse 1D Array(array=w1851) -> (reversed array=w1850:string[])
              n874 = case shown="True" w1852 {
                tunnel: w1856 -> [w1859 w1863]
                tunnel: [w1857 w1862] -> w1855
                tunnel: w1850 -> [_ w1861]
                tunnel: w1849 -> [w1858 w1860]
                frame False {
                  n875 = Build Array(w1859, w1858) -> (w1857:string[])
                }
                frame True {
                  n876 = Build Array (concatenate)(w1863, w1861, w1860) -> (w1862:string[])
                }
              }
            }
            "Table" <- w1844
          }
        }
      }
      frame "Process Cursor Point" {
        n877 = stacked-sequence {
          tunnel: [w1883] -> w1875
          tunnel: [TRUE] -> w1874
          tunnel: w1873 -> [_]
          tunnel: w1872 -> [_]
          tunnel: w1871 -> [w1884]
          frame #0 {
            n878 = local read "Kill Point"() -> (w1885:bool)
            n879 = global read "Results_plotter_Global.vi" "Row Reference"() -> (w1891:i32[][])
            n880 = local read "Cursor index"() -> (w1890:i32)
            n881 = Index Array(array=w1891, index (row)=w1890) -> (element=w1886:i32[])  [unwired: 1 in]
            n882 = local read "Result files to read"() -> (w1889:path[])
            n883 = Index Array(array=w1886, index #1=0 ("index"), index #2=1 ("index")) -> (element #1=w1888:i32, element #2=w1877:i32)
            "Selected Row" <- w1877
            n884 = Index Array(array=w1889, index=w1888) -> (element=w1882:path)
            n885 = call "GetRawDataFilePaths.vi"("Results file or Folder"=w1882) -> ("RawDataFilePaths"=w1881:string[])  [unwired: 9 in, 1 out]
            n886 = Index Array(array=w1881, index=w1877) -> (element=w1880:string)
            n887 = call "String_to_Pathname.vi"("Input String"=w1880) -> ("path"=w1879:path)
            n888 = case shown="True" w1885 {
              tunnel: w1882 -> [_ w1913]
              tunnel: w1877 -> [_ w1909]
              tunnel: w1884 -> [_ w1916]
              tunnel: ["What to do next?" ("t") w1915] -> w1883
              tunnel: w1879 -> [w1893 w1907]
              frame False {
                n889 = disable-structure shown="Enabled" {
                  disable-tunnel: w1893 -> [_ w1905]
                  frame Disabled {
                    n890 = local read "Table"() -> (w1904:string[][])
                    n891 = Index Array(array=w1904, index (col) #1=1 ("disabled index (col)"), index (col) #2=0 ("index (col)")) -> (element #1=w1897:string[], element #2=w1896:string[])  [unwired: 2 in]
                    n892 = Search 1D Array(1D array=w1896, element="Raw Data Filename") -> (index of element=w1900:i32)  [unwired: 1 in]
                    n893 = Index Array(array=w1897, index=w1900) -> (element=w1899:string)
                    n894 = call "String_to_Pathname.vi"("Input String"=w1899) -> ("path"=w1898:path)
                    n895 = call "Post_Process_Measurement.vi"("Raw data file"=w1898) -> ()  [unwired: 1 out]
                  }
                  frame Enabled {
                    n896 = call "Post_Process_Measurement.vi"("Raw data file"=w1905) -> ()  [unwired: 1 out]
                  }
                }
                n897 = local write "Process Point"(FALSE ("Kill Point")) -> ()
              }
              frame True {
                n898 = Strip Path(path=w1913) -> (name=w1908:string)  [unwired: 1 out]
                n899 = Strip Path(path=w1907) -> (name=w1906:string)  [unwired: 1 out]
                n900 = local read "nRows"() -> (w1918:i32)
                n901 = Format Into String(format string="Are you sure you want to remove the row in the results file \"%s\" generated from the raw data filename \"%s\"?", w1908, w1906) -> (resulting string=w1911:string)  [unwired: 2 in, 1 out]
                n902 = Less?(x=w1918, y=w1916) -> (x < y?=w1917:bool)
                n903 = Two Button Dialog(message=w1911) -> (T button?=w1910:bool)  [unwired: 2 out]
                n904 = case shown="True" w1917 {
                  tunnel: ["Create Selectors" "Initialise" ("t")] -> w1915
                  frame False {
                  }
                  frame True {
                  }
                }
                n905 = case shown="True" w1910 {
                  tunnel: w1913 -> [_ w1920]
                  tunnel: w1909 -> [_ w1919]
                  frame False {
                  }
                  frame True {
                    n906 = Build Array(w1919) -> (w1921:i32[])
                    n907 = call "Delete_unwanted_rows.vi"("Selected Rows"=w1921, "Filename"=w1920) -> ()  [unwired: 1 out]
                  }
                }
                n908 = local write "Kill Point"(FALSE ("Kill Point")) -> ()
              }
            }
          }
        }
      }
      frame "Edit template file" {
        n909 = stacked-sequence {
          frame #0 {
            n910 = local read "Template"() -> (w1930:path)
            n911 = call "Valid_Path.vi"("Filename"=w1930) -> ("Valid Path?"=w1929:bool)
            n912 = case shown="False" w1929 {
              tunnel: [T8."Edit Existing Template File" ("Mode") T8."Create New Template File" ("Mode")] -> w1933
              frame True {
              }
              frame False {
              }
            }
            n913 = local read "Results file"() -> (w1932:path)
            n914 = call "Edit_Template_File.vi"("Mode"=w1933, "Template Filename"=w1930, "Data Filename"=w1932) -> ("Template Filename Out"=w1931:path)  [unwired: 12 out]
            n915 = local write "Template"(w1931) -> ()
          }
          frame #1 {
            n916 = local read "Job Directory"() -> (w1936:path)
            n917 = Path To String(path=w1936) -> (string=w1939:string)
            n918 = call "Read_Write_Template.vi"("Mode"=Global_mode."Write Global to File", "Single Value In"=w1939, "Data type"="Log Folder Name" ("Variable name")) -> ()  [unwired: 5 in, 8 out]
            n919 = local write "Edit Template File"(FALSE ("Edit Template File")) -> ()
            n920 = Current VI's Path() -> (path=w1942:path)
            n921 = call "Open_Close_Front_Panel.ph.vi"("Front Panel Window:Open"=TRUE, "VI path"=w1942) -> ()  [unwired: 2 out]
          }
        }
      }
      frame "Save Plot Data" {
        n922 = global read "Results_plotter_Global.vi" "XY Graph Cluster"() -> (w1943:cluster{dbl[], dbl[]}[])
        n923 = local read "Tolerances"() -> (w1950:dbl[])
        n924 = local read "Absisca"() -> (w1949:u16)
        n925 = local read "Transpose"() -> (w1948:bool)
        n926 = local read "Multi Ordinate"() -> (w1947:i32[])
        n927 = global read "Results_plotter_Global.vi" "Precision"() -> (w1944:string[])
        n928 = stacked-sequence {
          seq-local: [w1961 _ _ _ _ _ _ _ _] -> [_ w1986 _ w2024 _ _ _ _ _]
          seq-local: [_ w1982 _ _ _ _ _ _ _] -> [_ _ _ _ _ _ _ w2146 _]
          seq-local: [_ _ _ _ _ w2076 _ _ _] -> [_ _ _ _ _ _ _ w2145 _]
          seq-local: [_ _ _ _ _ w2078 _ _ _] -> [_ _ _ _ _ _ w2114 _ _]
          seq-local: [_ _ _ w2022 _ _ _ _ _] -> [_ _ _ _ _ _ w2115 _ _]
          seq-local: [_ _ _ _ w2045 _ _ _ _] -> [_ _ _ _ _ w2071 _ _ _]
          seq-local: [w1958 _ _ _ _ _ _ _ _] -> [_ _ _ _ _ _ _ _ w2151]
          seq-local: [w1957 _ _ _ _ _ _ _ _] -> [_ w1974 _ _ _ _ _ _ _]
          seq-local: [_ _ w2003 _ _ _ _ _ _] -> [_ _ _ w2023 _ _ w2116 _ _]
          seq-local: [_ _ _ _ _ _ w2112 _ _] -> [_ _ _ _ _ _ _ w2143 _]
          tunnel: [_ _ _ _ _ _ _ _ TRUE] -> w1956
          tunnel: [_ _ _ _ _ _ _ _ w2149] -> w1955
          tunnel: w1953 -> [_ _ _ _ _ w2074 _ _ _]
          tunnel: w1954 -> [_ w1979 _ _ _ w2077 _ _ _]
          tunnel: [_ _ _ _ _ w2077 _ _ _] -> w1952
          tunnel: [_ _ _ _ _ w2074 _ _ _] -> w1951
          tunnel: w1950 -> [w1963 _ _ _ w2050 w2075 _ _ _]
          tunnel: w1943 -> [w1962 _ _ w2026 _ _ _ _ _]
          tunnel: w1949 -> [w1960 w1996 _ _ w2052 _ _ _ _]
          tunnel: w1948 -> [w1959 _ _ w2025 _ _ _ _ _]
          tunnel: w1947 -> [_ _ _ _ w2049 _ _ _ _]
          tunnel: [_ _ _ w2020 _ _ _ _ _] -> w1946
          tunnel: w1945 -> [_ _ w2006 w2020 _ _ _ _ _]
          tunnel: w1944 -> [_ _ _ w2019 _ w2070 _ _ _]
          frame #0 {
            n929 = local read "Save Surface Fit"() -> (w1958:bool)
            n930 = Not(x=w1959) -> (.not. x?=w1966:bool)
            n931 = for {
              tunnel: w1962 -> [w1973] mode=indexing
              tunnel: w1966 -> [w1970]
              shift-right: [w1968] -> w1964
              shift-left: dbl[] [] -> [w1969]
              n932 = Unbundle(w1973) -> (w1972:dbl[], w1971:dbl[])
              n933 = Select(t=w1972, s=w1970, f=w1971) -> (s? t:f=w1967:dbl[])
              n934 = Build Array (concatenate)(w1969, w1967) -> (w1968:dbl[])
            }
            n935 = Index Array(array=w1963, index=w1960) -> (element=w1957:dbl)
            n936 = call "Numeric_bins.vi"("Values"=w1964, "Tolerance"=w1957) -> ("Bin Centres"=w1961:dbl[])  [unwired: 2 out]
          }
          frame #1 {
            n937 = Index Array(array=w1979, index=w1996) -> (element=w1999:string)
            n938 = Match Pattern(string=w1999, regular expression=":") -> (before substring=w1998:string, after substring=w1997:string)  [unwired: 3 out]
            n939 = Concatenate Strings(w1998, " ", w1997, " =:" ("regular expression")) -> (w1981:string)
            n940 = Greater?(x=w1974, y=0.4) -> (0:w1994:bool)
            n941 = Greater?(x=w1974, y=0.09) -> (0:w1989:bool)
            n942 = call <vilib>:"Trim Whitespace.vi"("string"=w1981) -> ("trimmed string"=w1980:string)  [unwired: 1 in]
            n943 = Select(t=i16 0 ("precision (6)"), s=w1994, f=i16 2 ("precision (6)")) -> (s? t:f=w1990:i16)
            n944 = Select(t=w1990, s=w1989, f=i16 3) -> (s? t:f=w1987:i16)
            n945 = Number To Fractional String(number=w1986, precision (6)=w1987) -> (F-format string=w1985:string[])  [unwired: 2 out]
            n946 = for {
              tunnel: w1980 -> [w2002]
              tunnel: w1985 -> [w2000] mode=indexing
              tunnel: [w2001] -> w1984 mode=indexing
              n947 = Concatenate Strings(w2002, w2000) -> (w2001:string)
            }
            n948 = Build Array (concatenate)("Plot:Legend:" ("Input Element"), w1984, "End of:Plot Series:" ("Input Element")) -> (w1982:string[])
          }
          frame #2 {
            n949 = local read "Multi Ordinate?"() -> (w2005:bool)
            n950 = global read "Results_plotter_Global.vi" "Legend"() -> (w2004:string[])
            n951 = case shown="False" w2005 {
              tunnel: w2006 -> [w2010 _]
              tunnel: [w2007 w2018] -> w2003
              tunnel: w2004 -> [w2009 w2018]
              frame False {
                n952 = local read "Multi Ordinate"() -> (w2013:i32[])
                n953 = Index Array(array=w2013, index=0 ("Index")) -> (element=w2011:i32)
                n954 = Index Array(array=w2010, index=w2011) -> (element=w2008:string)
                n955 = for {
                  tunnel: w2009 -> [w2017] mode=indexing
                  tunnel: w2008 -> [w2016]
                  tunnel: [w2014] -> w2007 mode=indexing
                  n956 = Format Into String(format string="; %s", initial string=w2016, w2017) -> (resulting string=w2014:string)  [unwired: 1 in, 1 out]
                }
              }
              frame True {
              }
            }
          }
          frame #3 {
            n957 = call "Grid_Data.vi"("Transpose"=w2025, "XY Graph"=w2026, "Bin Centres"=w2024) -> ("Grided data"=w2021:dbl[][])  [unwired: 1 out]
            n958 = for {
              tunnel: w2023 -> [w2033] mode=indexing
              tunnel: [w2035] -> w2022 mode=indexing
              tunnel: w2021 -> [w2034] mode=indexing
              tunnel: w2020 -> [w2029]
              tunnel: w2019 -> [w2028]
              n959 = Match Pattern(string=w2033, regular expression=";") -> (before substring=w2030:string)  [unwired: 4 out]
              n960 = Search 1D Array(1D array=w2029, element=w2030) -> (index of element=w2031:i32)  [unwired: 1 out]
              n961 = Index Array(array=w2028, index=w2031) -> (element=w2027:string)
              n962 = for {
                tunnel: w2027 -> [w2040]
                tunnel: [w2039] -> w2036 mode=indexing
                tunnel: w2034 -> [w2037] mode=indexing
                n963 = Not A Number/Path/Refnum?(number/path/refnum=w2037) -> (NaN/Path/Refnum?=w2038:bool)
                n964 = case shown="True" w2038 {
                  tunnel: w2040 -> [w2043 _]
                  tunnel: [w2042 ""] -> w2039
                  tunnel: w2037 -> [w2041 _]
                  frame False {
                    n965 = call "Number_2_string.vi"("precision"=w2043, "number"=w2041) -> ("String"=w2042:string)
                  }
                  frame True {
                  }
                }
              }
              n966 = Build Array (concatenate)(w2033, w2036) -> (w2035:string[])
            }
          }
          frame #4 {
            n967 = Index Array(array=w2049, index=0 ("Index")) -> (element=w2047:i32)
            n968 = global read "Results_plotter_Global.vi" "Summarise"() -> (w2046:string[])
            n969 = for {
              shift-right: [w2059] -> w2045
              shift-left: i32[] [] -> [w2060]
              tunnel: w2052 -> [w2065]
              tunnel: w2047 -> [w2064]
              tunnel: w2050 -> [w2057] mode=indexing
              tunnel: w2046 -> [w2055] mode=indexing
              i -> [w2058]
              n970 = Equal?(x=w2064, y=w2058) -> (x = y?=w2063:bool)
              n971 = Not A Number/Path/Refnum?(number/path/refnum=w2057) -> (NaN/Path/Refnum?=w2056:bool)
              n972 = Equal?(x=w2065, y=w2058) -> (x = y?=w2062:bool)
              n973 = Equal?(x="FALSE", y=w2055) -> (x = y?=w2053:bool)
              n974 = Compound Arithmetic op=OR(w2062, w2063, w2056, w2053) -> (w2061:bool)
              n975 = case shown="False" w2061 {
                tunnel: w2060 -> [w2068 w2069]
                tunnel: [w2067 w2069] -> w2059
                tunnel: w2058 -> [w2066 _]
                frame False {
                  n976 = Build Array (concatenate)(w2068, w2066) -> (w2067:i32[])
                }
                frame True {
                }
              }
            }
          }
          frame #5 {
            n977 = local read "Plotted Series"() -> (w2073:bool[][])
            n978 = for {
              tunnel: w2075 -> [w2089]
              tunnel: [w2088] -> w2078 mode=indexing
              tunnel: w2071 -> [w2087]
              tunnel: w2074 -> [w2086]
              tunnel: w2073 -> [w2085] mode=indexing
              tunnel: i32[] [] -> [w2083]
              tunnel: w2070 -> [w2082]
              n979 = for {
                shift-right: [w2091] -> w2084
                shift-left: w2083 -> [w2092]
                tunnel: w2085 -> [w2090] mode=indexing
                i -> [w2093]
                n980 = case shown="True" w2090 {
                  tunnel: w2093 -> [_ w2097]
                  tunnel: w2092 -> [w2094 w2096]
                  tunnel: [w2094 w2095] -> w2091
                  frame False {
                  }
                  frame True {
                    n981 = Build Array (concatenate)(w2096, w2097) -> (w2095:i32[])
                  }
                }
              }
              n982 = for {
                tunnel: w2089 -> [w2105]
                tunnel: [w2106] -> w2088 mode=indexing
                tunnel: w2087 -> [w2100] mode=indexing
                tunnel: w2086 -> [w2103]
                tunnel: w2084 -> [w2102]
                tunnel: w2082 -> [w2099]
                n983 = for {
                  tunnel: w2102 -> [w2111] mode=indexing
                  tunnel: [w2110] -> w2107 mode=indexing
                  tunnel: w2100 -> [w2109]
                  tunnel: w2103 -> [w2108]
                  n984 = Index Array(array=w2108, index (row)=w2111, index (col)=w2109) -> (element=w2110:string)
                }
                n985 = Index Array(array=w2099, index=w2100) -> (element=w2101:string)
                n986 = Index Array(array=w2105, index=w2100) -> (element=w2104:dbl)
                n987 = call "Value_Occurence_Analysis.vi"("Average Numeric Values?"=FALSE, "Tolerance"=w2104, "Precision (3)"=w2101, "String Array"=w2107) -> ("Output String"=w2106:string)  [unwired: 2 out]
              }
            }
            n988 = for {
              tunnel: w2071 -> [w2081] mode=indexing
              tunnel: w2077 -> [w2080]
              tunnel: [w2079] -> w2076 mode=indexing
              n989 = Index Array(array=w2080, index=w2081) -> (element=w2079:string)
            }
          }
          frame #6 {
            n990 = for {
              shift-right: [w2129] -> w2112
              shift-left: string[][] [] -> [w2130]
              shift-right: [w2125] -> _
              shift-left: _ -> [w2126]
              tunnel: w2116 -> [w2127] mode=indexing
              tunnel: w2115 -> [w2119] mode=indexing
              tunnel: w2114 -> [w2118] mode=indexing
              i -> [w2124]
              n991 = Greater Than 0?(x=w2124) -> (x > 0?=w2123:bool)
              n992 = Match Pattern(string=w2127, regular expression="; ") -> (before substring=w2125:string)  [unwired: 4 out]
              n993 = Equal?(x=w2126, y=w2125) -> (x = y?=w2122:bool)
              n994 = Build Array (concatenate)(w2119, "", w2118) -> (w2117:string[])
              n995 = Compound Arithmetic op=AND(w2123, invert w2122) -> (w2121:bool)
              n996 = case shown="True" w2121 {
                tunnel: w2130 -> [w2134 w2137]
                tunnel: [w2133 w2136] -> w2129
                tunnel: w2117 -> [w2132 w2135]
                frame True {
                  n997 = Build Array (concatenate)(w2134, string[] [] ("array"), w2132) -> (w2133:string[][])
                }
                frame False {
                  n998 = Build Array (concatenate)(w2137, w2135) -> (w2136:string[][])
                }
              }
            }
          }
          frame #7 {
            w2142 = TRUE  # Simple Save?
            n999 = Build Array (concatenate)(w2146, w2145) -> (w2144:string[])
            n1000 = local read "Header"() -> (w2139:string)
            n1001 = call "Write_output_file.vi"("Output filename"="Output Filename", "Header"=w2139, "Channel Names"=w2144, "Data"=w2143, "Simple Save?"=w2142, "Summarise mode"=T9."No data summary") -> ("Output filename Out"=w2140:path)  [unwired: 6 in, 3 out]
            n1002 = local write "Output Filename"(w2140) -> ()
          }
          frame #8 {
            n1003 = local write "Save Plot data"(FALSE ("Save Plot data")) -> ()
            n1004 = local write "Header"("") -> ()
            n1005 = Select(t="Save Surface Fit data", s=w2151, f="Create Selectors") -> (s? t:f=w2149:string)
          }
        }
      }
      frame "What type of row averaging?" {
        n1006 = Two Button Dialog(message="Do you want to Combine rows with identical positions together?", 1:"Just average series" ("F button name (\"Cancel\")"), 2:"Combine rows" ("T button name (\"OK\")")) -> (T button?=w2157:bool)
        n1007 = Select(t="Combine rows" ("T button name (\"OK\")"), s=w2157, f="Average Rows together") -> (s? t:f=w2154:string)
      }
      frame "Combine rows" {
        w2167 = TRUE  # Show panel ?
        n1008 = local read "Output Filename"() -> (w2166:path)
        n1009 = call "Combined_file_Panel.vi"("Show panel ?"=w2167, "Output filename"=w2166) -> ("Only Plotted data?"=w2168:bool, "Include Empty Rows? Out"=w2169:bool, "Give Audit Channels Out"=w2170:bool, "Output filename Out"=w2165:path)  [unwired: 5 out]
        n1010 = case shown="False" w2168 {
          tunnel: w2172 -> [w2181 w2184]
          tunnel: [w2181 w2182] -> w2171
          frame False {
          }
          frame True {
            n1011 = global read "Results_plotter_Global.vi" "Plot Index values"() -> (w2186:dbl[][])
            n1012 = Index Array(array=w2186, index (row)=2) -> (element=w2183:dbl[])  [unwired: 1 in]
            n1013 = for {
              tunnel: w2184 -> [w2189]
              tunnel: w2183 -> [w2188] mode=indexing
              tunnel: [w2187] -> w2182 mode=indexing
              n1014 = Index Array(array=w2189, index (row)=w2188) -> (element=w2187:string[])  [unwired: 1 in]
            }
          }
        }
        n1015 = local write "Save Averaged rows"(FALSE ("Save Plot data")) -> ()
        n1016 = local read "X Ch Name"() -> (w2176:u16)
        n1017 = local read "Y Ch Name"() -> (w2177:u16)
        n1018 = local read "Z Ch Name"() -> (w2178:u16)
        n1019 = call "Find_Rows_to_Combine.vi"("Include Empty Rows?"=w2169, "file path (dialog if empty)"=w2165, "Give Audit Channels"=w2170, "Full Channel Names"=w2175, "Data"=w2171, "Z Column Index"=w2178, "Y Column Index"=w2177, "X Column Index"=w2176) -> ()  [unwired: 4 out]
        n1020 = local write "Output Filename"(w2165) -> ()
      }
      frame "Average Rows together" {
        n1021 = global read "Results_plotter_Global.vi" "XY Graph Cluster"() -> (w2191:cluster{dbl[], dbl[]}[])
        n1022 = local read "Tolerances"() -> (w2197:dbl[])
        n1023 = local read "Absisca"() -> (w2196:u16)
        n1024 = local read "Transpose"() -> (w2195:bool)
        n1025 = global read "Results_plotter_Global.vi" "Precision"() -> (w2193:string[])
        n1026 = global read "Results_plotter_Global.vi" "Summarise"() -> (w2192:string[])
        n1027 = stacked-sequence {
          seq-local: [w2209 _ _ _ _] -> [_ w2226 _ _ _]
          seq-local: [_ w2229 _ _ _] -> [_ _ _ w2311 _]
          seq-local: [w2205 _ _ _ _] -> [_ w2227 _ _ _]
          seq-local: [_ _ w2289 _ _] -> [_ _ _ w2305 _]
          tunnel: [_ _ _ _ TRUE] -> w2203
          tunnel: [_ _ _ _ "Create Selectors"] -> w2202
          tunnel: w2200 -> [_ w2232 _ _ w2314]
          tunnel: w2201 -> [_ _ w2290 _ w2313]
          tunnel: [_ _ _ _ w2313] -> w2199
          tunnel: [_ _ _ _ w2314] -> w2198
          tunnel: w2197 -> [w2211 w2230 _ _ _]
          tunnel: w2191 -> [w2210 _ _ _ _]
          tunnel: w2196 -> [w2208 _ _ _ _]
          tunnel: w2195 -> [w2207 _ _ _ _]
          tunnel: w2194 -> [w2204 _ _ _ _]
          tunnel: w2193 -> [_ w2231 _ _ _]
          tunnel: w2192 -> [_ w2228 w2291 _ _]
          tunnel: [w2204 _ _ _ _] -> w2190
          frame #0 {
            n1028 = Not(x=w2207) -> (.not. x?=w2214:bool)
            n1029 = for {
              tunnel: w2210 -> [w2221] mode=indexing
              tunnel: w2214 -> [w2218]
              shift-right: [w2216] -> w2212
              shift-left: dbl[] [] -> [w2217]
              n1030 = Unbundle(w2221) -> (w2220:dbl[], w2219:dbl[])
              n1031 = Select(t=w2220, s=w2218, f=w2219) -> (s? t:f=w2215:dbl[])
              n1032 = Build Array (concatenate)(w2217, w2215) -> (w2216:dbl[])
            }
            n1033 = Index Array(array=w2211, index=w2208) -> (element=w2206:dbl)
            n1034 = call "Numeric_bins.vi"("Values"=w2212, "Tolerance"=w2206) -> ("Bin Centres"=w2209:dbl[], "Bin Index"=w2205:i32[])  [unwired: 1 out]
          }
          frame #1 {
            n1035 = Array Size(array=w2226) -> (size(s)=w2225:i32)
            n1036 = global read "Results_plotter_Global.vi" "Plot Index values"() -> (w2223:dbl[][])
            n1037 = Index Array(array=w2223, index (row)=2) -> (element=w2222:dbl[])  [unwired: 1 in]
            n1038 = for {
              N: w2225 -> [_]
              tunnel: w2232 -> [w2242]
              tunnel: w2231 -> [w2241]
              tunnel: w2230 -> [w2240]
              tunnel: [w2233] -> w2229 mode=indexing
              tunnel: w2228 -> [w2239]
              tunnel: w2227 -> [w2237]
              tunnel: w2222 -> [w2236]
              i -> [w2238]
              n1039 = stacked-sequence {
                seq-local: [w2246 _] -> [_ w2265]
                tunnel: w2242 -> [_ w2266]
                tunnel: w2241 -> [_ w2264]
                tunnel: w2240 -> [_ w2263]
                tunnel: w2239 -> [_ w2262]
                tunnel: w2238 -> [w2245 _]
                tunnel: w2237 -> [w2244 _]
                tunnel: w2236 -> [w2243 _]
                tunnel: [_ w2260] -> w2235
                tunnel: [_ w2259] -> w2234
                frame #0 {
                  n1040 = for {
                    shift-right: [w2252] -> w2246
                    shift-left: i32[] [] -> [w2253]
                    tunnel: w2245 -> [w2251]
                    tunnel: w2244 -> [w2250] mode=indexing
                    tunnel: w2243 -> [w2248] mode=indexing
                    n1041 = Equal?(x=w2250, y=w2251) -> (x = y?=w2249:bool)
                    n1042 = case shown="False" w2249 {
                      tunnel: w2253 -> [w2254 w2257]
                      tunnel: [w2254 w2258] -> w2252
                      tunnel: w2248 -> [_ w2255]
                      frame False {
                      }
                      frame True {
                        n1043 = To Long Integer(number=w2255) -> (32bit integer=w2256:i32)
                        n1044 = Build Array (concatenate)(w2257, w2256) -> (w2258:i32[])
                      }
                    }
                  }
                }
                frame #1 {
                  n1045 = for {
                    tunnel: w2266 -> [w2280]
                    tunnel: w2265 -> [w2279]
                    tunnel: w2264 -> [w2277] mode=indexing
                    tunnel: w2263 -> [w2276] mode=indexing
                    tunnel: [w2275] -> w2260 mode=indexing
                    tunnel: w2262 -> [w2272] mode=indexing
                    shift-right: [w2267] -> w2259
                    shift-left: string[] [] -> [w2268]
                    i -> [w2274]
                    n1046 = for {
                      tunnel: w2280 -> [w2288]
                      tunnel: w2279 -> [w2287] mode=indexing
                      tunnel: [w2286] -> w2278 mode=indexing
                      tunnel: w2274 -> [w2285]
                      n1047 = Index Array(array=w2288, index (row)=w2287, index (col)=w2285) -> (element=w2286:string)
                    }
                    n1048 = Equal?(x="TRUE", y=w2272) -> (x = y?=w2271:bool)
                    n1049 = Not(x=w2271) -> (.not. x?=w2270:bool)
                    n1050 = call "Value_Occurence_Analysis.vi"("Average Numeric Values?"=w2270, "Tolerance"=w2276, "Precision (3)"=w2277, "String Array"=w2278) -> ("St Dev"=w2269:string, "Output String"=w2275:string)  [unwired: 1 out]
                    n1051 = case shown="False" w2270 {
                      tunnel: w2269 -> [_ w2284]
                      tunnel: w2268 -> [w2281 w2283]
                      tunnel: [w2281 w2282] -> w2267
                      frame False {
                      }
                      frame True {
                        n1052 = Build Array (concatenate)(w2283, w2284) -> (w2282:string[])
                      }
                    }
                  }
                }
              }
              n1053 = Build Array (concatenate)(w2235, w2234) -> (w2233:string[])
            }
          }
          frame #2 {
            n1054 = for {
              tunnel: w2291 -> [w2296] mode=indexing
              shift-right: [w2292] -> w2289
              shift-left: w2290 -> [w2293]
              tunnel: w2290 -> [w2294] mode=indexing
              n1055 = Equal?(x="TRUE", y=w2296) -> (x = y?=w2295:bool)
              n1056 = case shown="False" w2295 {
                tunnel: w2294 -> [w2302 _]
                tunnel: w2293 -> [w2299 w2303]
                tunnel: [w2298 w2303] -> w2292
                frame False {
                  n1057 = Concatenate Strings(w2302, "St Dev") -> (w2300:string)
                  n1058 = Build Array (concatenate)(w2299, w2300) -> (w2298:string[])
                }
                frame True {
                }
              }
            }
          }
          frame #3 {
            w2308 = FALSE  # Save Plotted rows only?
            w2310 = TRUE  # Simple Save?
            n1059 = local read "Output Filename"() -> (w2306:path)
            n1060 = local read "Header"() -> (w2307:string)
            n1061 = local read "Template"() -> (w2309:path)
            n1062 = call "Write_output_file.vi"("Output filename"=w2306, "Header"=w2307, "Template Filename"=w2309, "Channel Names"=w2305, "Data"=w2311, "Simple Save?"=w2310, "Save Plotted rows only?"=w2308, "Summarise mode"=T9."No data summary") -> ("Output filename Out"=w2312:path)  [unwired: 4 in, 3 out]
            n1063 = local write "Output Filename"(w2312) -> ()
          }
          frame #4 {
            n1064 = local write "Save Averaged rows"(FALSE ("Save Plot data")) -> ()
          }
        }
      }
      frame "Save Surface Fit data" {
        n1065 = local read "Transpose"() -> (w2318:bool)
        n1066 = local read "Tolerances"() -> (w2325:dbl[])
        n1067 = local read "Absisca"() -> (w2324:u16)
        n1068 = global read "Results_plotter_Global.vi" "Precision"() -> (w2321:string[])
        n1069 = stacked-sequence {
          seq-local: [w2332 _ _ _ _ _] -> [_ w2351 _ _ _ _]
          seq-local: [_ w2348 _ _ _ _] -> [_ _ _ _ w2435 _]
          seq-local: [_ _ w2374 _ _ _] -> [_ _ _ _ w2454 _]
          seq-local: [w2333 _ _ _ _ _] -> [_ _ w2375 _ _ _]
          seq-local: [_ _ w2370 _ _ _] -> [_ _ _ _ w2438 _]
          seq-local: [_ _ w2369 _ _ _] -> [_ _ _ w2405 _ _]
          seq-local: [_ _ _ w2400 _ _] -> [_ _ _ _ w2436 _]
          tunnel: [_ _ _ _ _ TRUE] -> w2329
          tunnel: [_ _ _ _ _ "Create Selectors"] -> w2328
          tunnel: w2326 -> [_ _ _ _ _ w2460]
          tunnel: w2327 -> [_ w2336 _ _ _ w2461]
          tunnel: w2325 -> [_ w2362 _ _ _ _]
          tunnel: w2324 -> [_ w2363 _ _ _ _]
          tunnel: [_ _ w2380 _ _ _] -> w2323
          tunnel: w2322 -> [_ w2339 w2380 _ _ _]
          tunnel: w2321 -> [_ _ w2376 _ _ _]
          tunnel: [_ _ _ _ _ w2461] -> w2320
          tunnel: [_ _ _ _ _ w2460] -> w2319
          tunnel: w2318 -> [_ _ _ w2399 _ _]
          frame #0 {
            n1070 = global read "Results_plotter_Global.vi" "X Values"() -> (w2332:dbl[])
            n1071 = global read "Results_plotter_Global.vi" "Raw Interpolation"() -> (w2330:dbl[][])
            n1072 = global read "Results_plotter_Global.vi" "Y Values"() -> (w2331:dbl[])
            n1073 = Insert Into Array(array=w2330, index (col)=0 ("disabled index (col)"), new element=w2331) -> (w2333:dbl[][])  [unwired: 1 in]
          }
          frame #1 {
            n1074 = global read "Results_plotter_Global.vi" "Y Axis Name"() -> (w2338:string)
            n1075 = Search 1D Array(1D array=w2339, element=w2338) -> (index of element=w2337:i32)  [unwired: 1 out]
            n1076 = Index Array(array=w2336, index=w2337) -> (element=w2335:string)
            n1077 = Match Pattern(string=w2335, regular expression=":") -> (before substring=w2365:string, after substring=w2364:string)  [unwired: 3 out]
            n1078 = Index Array(array=w2362, index=w2363) -> (element=w2353:dbl)
            n1079 = Concatenate Strings(w2365, " ", w2364, " =:" ("regular expression")) -> (w2347:string)
            n1080 = Greater?(x=w2353, y=0.9) -> (0:w2360:bool)
            n1081 = Greater?(x=w2353, y=0.09) -> (0:w2355:bool)
            n1082 = call <vilib>:"Trim Whitespace.vi"("string"=w2347) -> ("trimmed string"=w2346:string)  [unwired: 1 in]
            n1083 = Select(t=i16 0 ("precision (6)"), s=w2360, f=i16 2 ("precision (6)")) -> (s? t:f=w2356:i16)
            n1084 = Select(t=w2356, s=w2355, f=i16 3) -> (s? t:f=w2352:i16)
            n1085 = Number To Fractional String(number=w2351, precision (6)=w2352) -> (F-format string=w2350:string[])  [unwired: 2 out]
            n1086 = for {
              tunnel: w2346 -> [w2368]
              tunnel: w2350 -> [w2366] mode=indexing
              tunnel: [w2367] -> w2341 mode=indexing
              n1087 = Concatenate Strings(w2368, w2366) -> (w2367:string)
            }
            n1088 = Build Array (concatenate)("Channel:Values:Plotted" ("Input Element"), "Axis:Name:" ("Input Element"), "Axis:Values:" ("Input Element"), w2341) -> (w2348:string[])
          }
          frame #2 {
            n1089 = global read "Results_plotter_Global.vi" "X Axis Name"() -> (w2373:string)
            n1090 = Concatenate Strings(w2373, " =" ("string")) -> (w2371:string)
            n1091 = local read "Multi Ordinate"() -> (w2379:i32[])
            n1092 = Index Array(array=w2379, index=0 ("Index")) -> (element=w2377:i32)
            n1093 = Index Array(array=w2376, index=w2377) -> (element=w2369:string)
            n1094 = Index Array(array=w2380, index=w2377) -> (element=w2370:string)
            n1095 = for {
              tunnel: w2370 -> [w2382]
              tunnel: [w2385] -> w2374 mode=indexing
              tunnel: w2369 -> [w2384]
              tunnel: w2375 -> [w2383] mode=indexing
              tunnel: w2371 -> [w2381]
              n1096 = for {
                tunnel: w2383 -> [w2388] mode=indexing
                tunnel: [w2387] -> w2386 mode=indexing
                tunnel: w2384 -> [w2390]
                n1097 = Not A Number/Path/Refnum?(number/path/refnum=w2388) -> (NaN/Path/Refnum?=w2389:bool)
                n1098 = case shown="False" w2389 {
                  tunnel: w2390 -> [w2393 _]
                  tunnel: w2388 -> [w2392 _]
                  tunnel: [w2391 ""] -> w2387
                  frame False {
                    n1099 = call "Number_2_string.vi"("precision"=w2393, "number"=w2392) -> ("String"=w2391:string)
                  }
                  frame True {
                  }
                }
              }
              n1100 = Build Array (concatenate)(w2382, w2381, w2386) -> (w2385:string[])
            }
          }
          frame #3 {
            w2404 = "\t"
            n1101 = global read "Results_plotter_Global.vi" "Intensity Plot data in rows"() -> (w2406:dbl[][])
            n1102 = global read "Results_plotter_Global.vi" "Value plotted Name"() -> (w2403:string)
            n1103 = global read "Results_plotter_Global.vi" "X Axis Name"() -> (w2397:string)
            n1104 = global read "Results_plotter_Global.vi" "Y Axis Name"() -> (w2396:string)
            n1105 = case shown="False" w2399 {
              tunnel: [w2407 w2410] -> w2398
              tunnel: w2397 -> [w2408 w2410]
              tunnel: w2396 -> [w2407 w2409]
              tunnel: [w2408 w2409] -> w2395
              frame False {
              }
              frame True {
              }
            }
            n1106 = Concatenate Strings(w2398, w2404, w2395, w2404, w2403, "\r\n") -> (w2401:string)
            n1107 = for {
              tunnel: w2406 -> [w2416] mode=indexing
              tunnel: w2405 -> [w2421]
              shift-right: [w2415] -> w2400
              shift-left: w2401 -> [w2420]
              n1108 = Index Array(array=w2416, index=0) -> (element=w2412:dbl)
              n1109 = Index Array(array=w2416, index=1) -> (element=w2411:dbl)
              n1110 = Index Array(array=w2416, index=2) -> (element=w2414:dbl)
              n1111 = Not A Number/Path/Refnum?(number/path/refnum=w2414) -> (NaN/Path/Refnum?=w2413:bool)
              n1112 = case shown="False" w2413 {
                tunnel: w2421 -> [w2432 _]
                tunnel: w2420 -> [w2431 w2433]
                tunnel: w2414 -> [w2430 _]
                tunnel: [w2429 w2433] -> w2415
                tunnel: w2412 -> [w2428 _]
                tunnel: w2411 -> [w2427 _]
                frame False {
                  w2423 = "\t"
                  n1113 = call "Number_2_string.vi"("number"=w2428) -> ("String"=w2426:string)  [unwired: 1 in]
                  n1114 = call "Number_2_string.vi"("number"=w2427) -> ("String"=w2425:string)  [unwired: 1 in]
                  n1115 = call "Number_2_string.vi"("precision"=w2432, "number"=w2430) -> ("String"=w2424:string)
                  n1116 = Concatenate Strings(w2431, w2426, w2423, w2425, w2423, w2424, "\r\n") -> (w2429:string)
                }
                frame True {
                }
              }
            }
          }
          frame #4 {
            w2450 = TRUE  # append to file? (new file:F)
            n1117 = global read "Results_plotter_Global.vi" "Surface Integral"() -> (w2449:dbl)
            n1118 = global read "Results_plotter_Global.vi" "Surface Area"() -> (w2448:dbl)
            n1119 = Initialize Array("", 10 ("Dimension Size")) -> (w2459:string[])
            n1120 = Divide(x=w2449, y=w2448) -> (x/y=w2447:dbl)
            n1121 = call "Asterisk_header.vi"("Channel names"=w2459) -> ("Header string"=w2437:string)
            n1122 = call "Value_to_string.vi"("Value"=w2449, "Label for value"="Surface Integral") -> ("Output string"=w2444:string)  [unwired: 1 in]
            n1123 = call "Value_to_string.vi"("Value"=w2448, "Label for value"="Surface Area") -> ("Output string"=w2445:string)  [unwired: 1 in]
            n1124 = call "Value_to_string.vi"("Value"=w2447, "Label for value"="Surface Average") -> ("Output string"=w2443:string)  [unwired: 1 in]
            n1125 = Concatenate Strings(w2445, w2444, w2443) -> (w2440:string)
            n1126 = call "Ch_names_to_rows.vi"("Channel Names"=w2435) -> ("3 Row names"=w2434:string[][])
            n1127 = local read "Output Filename"() -> (w2451:path)
            n1128 = Build Array (concatenate)(w2434, w2454) -> (w2452:string[][])
            n1129 = Array To Spreadsheet String(array=w2452, 3:"%s" ("format string")) -> (spreadsheet string=w2439:string)  [unwired: 1 out]
            n1130 = Format Into String(format string="\n%s\n\n%s\n%s\n\n\nInterpolated Surface of %s\n%s\n%s\n%s\n\n\n%s", w2437, w2436, w2437, w2438, w2437, w2439, w2437, w2440) -> (resulting string=w2442:string)  [unwired: 2 in, 1 out]
            n1131 = call "Write_Characters_To_File.vi"("file path (dialog if empty)"=w2451, "character string"=w2442, "append to file? (new file:F)"=w2450) -> ()  [unwired: 2 in, 4 out]
          }
          frame #5 {
            n1132 = local write "Save Surface Fit"(FALSE ("Save Plot data")) -> ()
          }
        }
      }
      frame "Save Data in Rows" {
        w2476 = TRUE  # Show panel ?
        n1133 = local read "Output Filename"() -> (w2473:path)
        n1134 = local write "Save Data in Rows"(FALSE ("Save All data")) -> ()
        n1135 = call "Output_file_Panel.vi"("Show panel ?"=w2476, "Channel Names"=w2471, "Header"="Header", "Output filename"=w2473) -> ("Save Full Res Data?"=w2468:bool, "Desired Columns"=w2477:i32[], "Header Out"=w2475:string, "Output filename Out"=w2479:path, "Channels to Tabulate in header Out"=w2465:i32[], "Save Plotted rows only?"=w2466:bool, "Summarise mode"=w2474:T9, "Grouping info"=w2467:T14[])
        "Plotted rows only?" <- w2466
        n1136 = case shown="False" w2468 {
          tunnel: w2479 -> [w2495 w2497]
          tunnel: w2477 -> [w2494 _]
          tunnel: w2475 -> [w2493 _]
          tunnel: w2466 -> [w2492 _]
          tunnel: w2474 -> [w2491 _]
          tunnel: w2472 -> [w2490 _]
          tunnel: w2471 -> [w2489 _]
          tunnel: [w2488 w2497] -> w2470
          tunnel: ["Create Selectors" "Is Filename Empty?"] -> w2469
          tunnel: w2467 -> [w2484 _]
          tunnel: w2465 -> [w2483 _]
          frame False {
            w2486 = FALSE  # Simple Save?
            n1137 = local read "Template"() -> (w2487:path)
            n1138 = call "Write_output_file.vi"("Output filename"=w2495, "Header"=w2493, "Template Filename"=w2487, "Channel Names"=w2489, "Data"=w2490, "Desired Columns"=w2494, "Simple Save?"=w2486, "Save Plotted rows only?"=w2492, "Summarise mode"=w2491, "Grouping info"=w2484, "Channels to Tabulate in header"=w2483) -> ("Output filename Out"=w2488:path)  [unwired: 1 in, 3 out]
          }
          frame True {
            "Mode" <- Plotter_Mode."Save file" ("Mode")
          }
        }
        n1139 = local write "Output Filename"(w2470) -> ()
      }
      frame "Is Filename Empty?" {
        # "This Express VI is the reason we can't strip object code from ResultsFilePlotter; may be able to convert to standard VI"
        n1140 = call "File Dialog"("start path"="Full_Res_Results_Folder", "prompt"="Please select a new or existing folder to save the results files in") -> ("selected path"=w2501:path, "cancelled"=w2499:bool)  [unwired: 5 in, 7 out]
        n1141 = local write "Full_Res_Results_Folder"(w2501) -> ()
        n1142 = case shown="False" w2499 {
          tunnel: ["Full Res file manipulator" ("f") "Create Selectors" ("t")] -> w2503
          frame False {
          }
          frame True {
          }
        }
      }
      frame "Check for overwrite or append" {
        n1143 = local read "Output Filename"() -> (w2517:path)
        n1144 = Format Into String(format string="Do you want to append to the result file\n\"%s\"" ("message"), w2517) -> (resulting string=w2512:string)  [unwired: 2 in, 1 out]
        n1145 = call <vilib>:"Three Button Dialog.vi"("Window Title (\"\")"="Output File Dialog" ("Window Title (\"\")"), "Right Button Text (\"Cancel\")"="Cancel" ("Button 3 Name"), "Center Button Text (\"No\")"="Overwrite" ("F button name (\"Cancel\")"), "Left Button Text (\"Yes\")"="Append" ("T button name (\"OK\")"), "message"=w2512) -> ("Which Button?"=w2511:T11)  [unwired: 6 out]
        n1146 = case shown="\"Center Button\"" w2511 {
          tunnel: w2517 -> [_ w2524 _]
          tunnel: ["Full Res file manipulator" "Full Res file manipulator" "Create Selectors" ("t")] -> w2510
          frame "Left Button" {
          }
          frame "Center Button" {
            n1147 = call "Delete_with_Check.vi"("FilePath"=w2524) -> ()  [unwired: 1 out]
          }
          frame "Right Button", Default {
          }
        }
      }
      frame "Create Plot summary" {
        w2539 = TRUE  # Summarise All
        n1148 = global read "Results_plotter_Global.vi" "Plot Index values"() -> (w2542:dbl[][])
        n1149 = local read "Intensity Plot?"() -> (w2538:bool)
        n1150 = global read "Results_plotter_Global.vi" "Row Reference"() -> (w2534:i32[][])
        n1151 = Index Array(array=w2534, index (col)=0 ("disabled index (col)")) -> (element=w2533:i32[])  [unwired: 1 in]
        n1152 = Index Array(array=w2542, index (row)=2) -> (element=w2544:dbl[])  [unwired: 1 in]
        n1153 = Select(t="Save Intensity plot as jpg", s=w2538, f="Create summary per series") -> (s? t:f=w2529:string)
        n1154 = To Long Integer(number=w2544) -> (32bit integer=w2541:i32[])
        n1155 = for {
          tunnel: w2549 -> [w2562]
          tunnel: [w2561] -> w2540 mode=indexing
          tunnel: w2541 -> [w2559] mode=indexing
          tunnel: w2533 -> [w2560]
          shift-right: [w2556] -> w2531
          shift-left: i32[] [] -> [w2557]
          n1156 = Index Array(array=w2560, index=w2559) -> (element=w2555:i32)
          n1157 = Search 1D Array(1D array=w2557, element=w2555) -> (index of element=w2558:i32)  [unwired: 1 out]
          n1158 = Index Array(array=w2562, index (row)=w2559) -> (element=w2561:string[])  [unwired: 1 in]
          n1159 = case shown="0, Default" w2558 {
            tunnel: w2555 -> [_ w2566]
            tunnel: w2557 -> [w2563 w2565]
            tunnel: [w2563 w2564] -> w2556
            frame 0, Default {
            }
            frame -1 {
              n1160 = Build Array (concatenate)(w2565, w2566) -> (w2564:i32[])
            }
          }
        }
        n1161 = local read "Result files to read"() -> (w2530:path[])
        n1162 = for {
          tunnel: w2531 -> [w2554] mode=indexing
          tunnel: w2530 -> [w2553]
          tunnel: [w2550] -> w2528 mode=indexing
          n1163 = Index Array(array=w2553, index=w2554) -> (element=w2552:path)
          n1164 = Strip Path(path=w2552) -> (name=w2551:string)  [unwired: 1 out]
          n1165 = call "Add_filename_suffix.vi"("Filename"=w2551) -> ("Base name"=w2550:string)  [unwired: 1 in, 3 out]
        }
        n1166 = call "Value_Occurence_Analysis.vi"("String Array"=w2528) -> ("Output String"=w2527:string)  [unwired: 3 in, 2 out]
        n1167 = global write "Results_plotter_Global.vi" "Current Data Filenames"(w2527) -> ()
        n1168 = call "Summarise.vi"("Channel Names"=w2545, "Data"=w2540, "Summarise All"=w2539) -> ("Summary"=w2547:string[][])  [unwired: 2 in]
        n1169 = global write "Results_plotter_Global.vi" "Plot Summary"(w2547) -> ()
      }
      frame "Create summary per series" {
        n1170 = local read "Plotted Series"() -> (w2570:bool[][])
        n1171 = global read "Results_plotter_Global.vi" "Plot Summary"() -> (w2568:string[][])
        n1172 = for {
          tunnel: w2570 -> [w2587] mode=indexing
          tunnel: i32[] [] -> [w2586]
          tunnel: w2575 -> [w2584]
          tunnel: w2572 -> [w2582]
          shift-right: [w2576] -> w2567
          shift-left: w2568 -> [w2578]
          w2581 = TRUE  # Summarise All
          n1173 = for {
            shift-right: [w2595] -> w2585
            shift-left: w2586 -> [w2596]
            tunnel: w2587 -> [w2594] mode=indexing
            i -> [w2597]
            n1174 = case shown="True" w2594 {
              tunnel: w2597 -> [_ w2601]
              tunnel: w2596 -> [w2598 w2600]
              tunnel: [w2598 w2599] -> w2595
              frame False {
              }
              frame True {
                n1175 = Build Array (concatenate)(w2600, w2601) -> (w2599:i32[])
              }
            }
          }
          n1176 = for {
            tunnel: w2585 -> [w2593] mode=indexing
            tunnel: w2584 -> [w2592]
            tunnel: [w2591] -> w2583 mode=indexing
            n1177 = Index Array(array=w2592, index (row)=w2593) -> (element=w2591:string[])  [unwired: 1 in]
          }
          n1178 = call "Summarise.vi"("Channel Names"=w2582, "Data"=w2583, "Summarise All"=w2581) -> ("Summary"=w2579:string[][])  [unwired: 2 in]
          n1179 = Index Array(array=w2579, index (col)=2 ("disabled index (col)")) -> (element=w2577:string[])  [unwired: 1 in]
          n1180 = for {
            tunnel: w2578 -> [w2590] mode=indexing
            tunnel: w2577 -> [w2589] mode=indexing
            tunnel: [w2588] -> w2576 mode=indexing
            n1181 = Build Array (concatenate)(w2590, w2589) -> (w2588:string[])
          }
        }
        n1182 = global write "Results_plotter_Global.vi" "Plot Summary"(w2567) -> ()
      }
      frame "Save Intensity plot as jpg" {
        n1183 = local read "Job Directory"() -> (w2608:path)
        n1184 = global read "Constants_global.vi" "EnFlo SW Folder"() -> (w2610:path)
        n1185 = Build Path(base path=w2610, name or relative path=path "Anemometry/Anemometry Sub Vis/Data_plotting_vis/Intensity Plot Vis") -> (appended path=w2604:path)
        n1186 = call "Remote_call_prep.vi"("Vi Name in"="Create picture Vi Name", "Job Directory In"=w2608, "VI Directory"=w2604) -> ("Vi Name out"=w2606:string, "Job Directory out"=w2603:path, "cancelled"=w2602:bool)
        n1187 = local write "Create picture Vi Name"(w2606) -> ()
        n1188 = local write "Job Directory"(w2603) -> ()
        n1189 = Build Path(base path=w2604, name or relative path=w2606) -> (appended path=w2605:path)
        n1190 = case shown="False" w2602 {
          tunnel: w2605 -> [w2619 _]
          tunnel: w2603 -> [w2618 _]
          frame False {
            n1191 = Open VI Reference(type specifier VI Refnum (for type only)="type specifier VI Refnum (for type only)", vi path=w2619) -> (vi reference=w2624:refnum<vi>, error out=w2623:errorcluster)  [unwired: 2 in, 2 out]
            n1192 = property class="VI Interface Type 0"(reference=w2624, error in=w2623, "Front Panel Window:Open"=TRUE) -> (reference out=w2620:refnum<vi>, error out=w2621:errorcluster)
            n1193 = local read "Intensity Graph"() -> (w2627:dbl[][])
            n1194 = local read "No of Contours"() -> (w2617:i32)
            n1195 = call-by-ref "?"(reference=w2620, error in=w2621, "No of Contours"=w2617, "Job Directory"=w2618, "Intensity Graph"=w2627) -> (reference out=w2626:refnum<vi>, error out=w2625:errorcluster)  [unwired: 3 in]
            n1196 = Close Reference(reference=w2626, error in (no error)=w2625) -> ()  [unwired: 1 out]
          }
          frame True {
          }
        }
        n1197 = local write "Save Plot as jpg"(FALSE ("Save All data")) -> ()
      }
      frame "Run Calculation Routine" {
        n1198 = stacked-sequence {
          seq-local: [w2636 _ _] -> [_ w2646 _]
          seq-local: [w2635 _ _] -> [_ w2647 _]
          tunnel: [_ w2645 _] -> w2630
          tunnel: w2629 -> [_ _ _]
          frame #0 {
            n1199 = global read "Constants_global.vi" "EnFlo SW Folder"() -> (w2642:path)
            n1200 = Build Path(base path=w2642, name or relative path=path "Anemometry/Anemometry Sub Vis/Data_plotting_vis/Calculation Vis") -> (appended path=w2639:path)
            n1201 = local read "Job Directory"() -> (w2638:path)
            n1202 = call "Remote_call_prep.vi"("Vi Name in"="...using routine", "Job Directory In"=w2638, "VI Directory"=w2639) -> ("Vi Name out"=w2640:string, "Job Directory out"=w2637:path, "cancelled"=w2636:bool)
            n1203 = local write "Job Directory"(w2637) -> ()
            n1204 = local write "...using routine"(w2640) -> ()
            n1205 = Build Path(base path=w2639, name or relative path=w2640) -> (appended path=w2635:path)
          }
          frame #1 {
            n1206 = case shown="False" w2646 {
              tunnel: w2647 -> [w2655 _]
              tunnel: [w2651 w2668] -> w2645
              tunnel: "What to do next?" -> [w2650 w2668]
              frame False {
                n1207 = Open VI Reference(type specifier VI Refnum (for type only)="VI Refnum Calculation", vi path=w2655) -> (vi reference=w2661:refnum<vi>, error out=w2660:errorcluster)  [unwired: 1 in, 3 out]
                n1208 = property class="VI Interface Type 1"(reference=w2661, error in=w2660, "Front Panel Window:Open"=TRUE) -> (reference out=w2657:refnum<vi>, error out=w2658:errorcluster)
                n1209 = call-by-ref "?"(reference=w2657, error in=w2658) -> (reference out=w2663:refnum<vi>, error out=w2662:errorcluster, "New Values In"=w2648:string[][], "New Chs In"=w2656:string[])  [unwired: 2 in]
                n1210 = for {
                  tunnel: w2656 -> [w2666] mode=indexing
                  tunnel: [w2665] -> w2649 mode=indexing
                  n1211 = call "Check_Ch_Name_colons.vi"("No of Colons"=2, "Ch Name in"=w2666) -> ("Ch Name out"=w2665:string)
                }
                n1212 = Empty String/Path?(string/path=w2649) -> (empty?=w2653:bool[])
                n1213 = Or Array Elements(Boolean array=w2653) -> (logical OR=w2652:bool)
                n1214 = Close Reference(reference=w2663, error in (no error)=w2662) -> ()  [unwired: 1 out]
                n1215 = Select(t=w2650, s=w2652, f="Input calculated values") -> (s? t:f=w2651:string)
                n1216 = global write "Results_plotter_Global.vi" "New Values In"(w2648) -> ()
                n1217 = global write "Results_plotter_Global.vi" "New Chs In"(w2649) -> ()
              }
              frame True {
              }
            }
          }
          frame #2 {
            w2671 = FALSE ("Raw DF in Orig Pos?")
            n1218 = local write "Edit Raw Data Header Info"(w2671) -> ()
            n1219 = local write "Calculate new metadata"(FALSE ("Save All data")) -> ()
            n1220 = local write "Plotted rows only?"(TRUE ("Plotted rows only?")) -> ()
            n1221 = local write "Raw DF in Orig Pos?"(w2671) -> ()
            n1222 = local write "Edit Raw DF?"(w2671) -> ()
            n1223 = local write "Mode"(Plotter_Mode."Edit values per row" ("Mode")) -> ()
          }
        }
      }
      frame "Input calculated values" {
        n1224 = local read "Result files to read"() -> (w2677:path[])
        n1225 = local read "Raw DF in Orig Pos?"() -> (w2674:bool)
        n1226 = stacked-sequence {
          seq-local: [w2681 _ _ _] -> [_ w2694 w2706 _]
          seq-local: [_ w2691 _ _] -> [_ _ w2707 _]
          tunnel: [_ _ _ w2759] -> w2679
          tunnel: w2677 -> [_ _ w2708 _]
          tunnel: w2676 -> [_ _ w2705 _]
          tunnel: w2675 -> [_ _ w2704 _]
          tunnel: w2674 -> [_ _ w2703 _]
          tunnel: w2673 -> [_ _ _ w2756]
          frame #0 {
            n1227 = global read "Results_plotter_Global.vi" "Plot Index values"() -> (w2684:dbl[][])
            n1228 = global read "Results_plotter_Global.vi" "Row Reference"() -> (w2685:i32[][])
            n1229 = Index Array(array=w2684, index (row)=2) -> (element=w2682:dbl[])  [unwired: 1 in]
            n1230 = for {
              tunnel: w2685 -> [w2689]
              tunnel: w2682 -> [w2688] mode=indexing
              tunnel: [w2687] -> w2681 mode=indexing
              n1231 = Index Array(array=w2689, index (row)=w2688) -> (element=w2687:i32[])  [unwired: 1 in]
            }
            n1232 = local write "Delete Plotted data from file"(FALSE ("Save All data")) -> ()
          }
          frame #1 {
            n1233 = Index Array(array=w2694, index (col)=0 ("disabled index (col)")) -> (element=w2690:i32[])  [unwired: 1 in]
            n1234 = for {
              shift-right: [w2696] -> w2691
              shift-left: i32[] [] -> [w2697]
              tunnel: w2690 -> [w2695] mode=indexing
              n1235 = Search 1D Array(1D array=w2697, element=w2695) -> (index of element=w2698:i32)  [unwired: 1 out]
              n1236 = case shown="-1" w2698 {
                tunnel: w2697 -> [w2699 w2702]
                tunnel: [w2699 w2701] -> w2696
                tunnel: w2695 -> [_ w2700]
                frame 0, Default {
                }
                frame -1 {
                  n1237 = Build Array (concatenate)(w2702, w2700) -> (w2701:i32[])
                }
              }
            }
          }
          frame #2 {
            n1238 = for {
              tunnel: w2708 -> [w2715]
              tunnel: w2707 -> [w2712] mode=indexing
              tunnel: w2706 -> [w2713]
              tunnel: w2705 -> [w2711]
              tunnel: w2704 -> [w2710]
              tunnel: w2703 -> [w2709]
              # "New Values"
              # "Row in file"
              n1239 = Index Array(array=w2715, index=w2712) -> (element=w2714:path)
              n1240 = stacked-sequence {
                seq-local: [w2720 _] -> [_ w2754]
                seq-local: [w2718 _] -> [_ w2749]
                tunnel: w2714 -> [_ w2755]
                tunnel: w2713 -> [w2722 _]
                tunnel: w2712 -> [w2721 _]
                tunnel: w2711 -> [_ _]
                tunnel: w2710 -> [_ _]
                tunnel: w2709 -> [_ w2753]
                frame #0 {
                  n1241 = global read "Results_plotter_Global.vi" "New Values In"() -> (w2716:string[][])
                  n1242 = for {
                    tunnel: w2721 -> [w2733]
                    tunnel: w2722 -> [w2729] mode=indexing
                    shift-right: [w2727] -> w2720
                    shift-left: i32[] [] -> [w2728]
                    shift-right: [w2726] -> w2718
                    shift-left: string[][] [] -> [w2725]
                    tunnel: w2716 -> [w2724]
                    i -> [w2723]
                    n1243 = Index Array(array=w2729, index=0) -> (element=w2731:i32)
                    n1244 = Equal?(x=w2731, y=w2733) -> (x = y?=w2730:bool)
                    n1245 = case shown="True" w2730 {
                      tunnel: w2729 -> [_ w2739]
                      tunnel: w2728 -> [w2735 w2744]
                      tunnel: [w2735 w2742] -> w2727
                      tunnel: w2725 -> [w2734 w2740]
                      tunnel: [w2734 w2741] -> w2726
                      tunnel: w2724 -> [_ w2737]
                      tunnel: w2723 -> [_ w2736]
                      frame False {
                      }
                      frame True {
                        n1246 = Index Array(array=w2737, index (row)=w2736) -> (element=w2738:string[])  [unwired: 1 in]
                        n1247 = Index Array(array=w2739, index=1) -> (element=w2743:i32)
                        n1248 = Build Array (concatenate)(w2744, w2743) -> (w2742:i32[])
                        n1249 = Build Array (concatenate)(w2740, w2738) -> (w2741:string[][])
                      }
                    }
                  }
                }
                frame #1 {
                  w2748 = FALSE  # Edit all Rows?
                  w2750 = FALSE  # Edit Raw DF?
                  w2751 = FALSE  # Edit Raw Data Header Info
                  w2752 = FALSE  # Value  Constant?
                  n1250 = global read "Results_plotter_Global.vi" "New Chs In"() -> (w2746:string[])
                  n1251 = local read "Job Directory"() -> (w2747:path)
                  n1252 = call "Add_Update_Values.vi"("Filename"=w2755, "Value  Constant?"=w2752, "Edit Raw data files?"=w2750, "New Chs In"=w2746, "Edit Raw Data Header Info"=w2751, "New Values In"=w2749, "Selected Rows"=w2754, "Edit all Rows?"=w2748, "Raw DF in Orig Pos?"=w2753, "Job Directory"=w2747) -> ()  [unwired: 1 in, 5 out]
                }
              }
            }
          }
          frame #3 {
            n1253 = local read "nRows"() -> (w2758:i32)
            n1254 = Less?(x=w2758, y=w2756) -> (x < y?=w2757:bool)
            n1255 = Current VI's Path() -> (path=w2760:path)
            n1256 = case shown="True" w2757 {
              tunnel: ["Create Selectors" "Initialise" ("t")] -> w2759
              frame False {
              }
              frame True {
              }
            }
            n1257 = call "Bring_to_front.vi"("path"=w2760) -> ()
          }
        }
      }
      frame "Save XY plot as jpg" {
        n1258 = local read "Create picture Vi Name"() -> (w2767:string)
        n1259 = local read "Job Directory"() -> (w2770:path)
        n1260 = global read "Constants_global.vi" "EnFlo SW Folder"() -> (w2772:path)
        n1261 = Build Path(base path=w2772, name or relative path=path "Anemometry/Anemometry Sub Vis/Data_plotting_vis/XY Plot Vis") -> (appended path=w2768:path)
        n1262 = call "Remote_call_prep.vi"("Vi Name in"=w2767, "Job Directory In"=w2770, "VI Directory"=w2768) -> ("Vi Name out"=w2769:string, "Job Directory out"=w2765:path, "cancelled"=w2764:bool)
        n1263 = local write "Create picture Vi Name"(w2769) -> ()
        n1264 = local write "Job Directory"(w2765) -> ()
        n1265 = Build Path(base path=w2768, name or relative path=w2769) -> (appended path=w2766:path)
        n1266 = case shown="False" w2764 {
          tunnel: [w2785 FALSE ("Saved Automatically?")] -> w2775
          tunnel: [w2784 path "" ("Plot data file")] -> w2774
          tunnel: [w2783 "" ("Tex Info String")] -> w2773
          tunnel: w2766 -> [w2782 _]
          tunnel: w2765 -> [w2781 _]
          frame False {
            n1267 = Open VI Reference(type specifier VI Refnum (for type only)="type specifier VI Refnum (for type only) 2", vi path=w2782) -> (vi reference=w2792:refnum<vi>, error out=w2791:errorcluster)  [unwired: 1 in, 3 out]
            n1268 = property class="VI Interface Type 2"(reference=w2792, error in=w2791, "Front Panel Window:Open"=TRUE) -> (reference out=w2788:refnum<vi>, error out=w2789:errorcluster)
            n1269 = global read "Results_plotter_Global.vi" "XY Graph Cluster"() -> (w2786:cluster{dbl[], dbl[]}[])
            n1270 = call-by-ref "?"(reference=w2788, error in=w2789, "Plot Array"=w2786, "Template"=w2781) -> (reference out=w2794:refnum<vi>, error out=w2793:errorcluster, "Saved Automatically?"=w2785:bool, "Tex Info String"=w2783:string, "Plot data file"=w2784:path)
            n1271 = Close Reference(reference=w2794, error in (no error)=w2793) -> ()  [unwired: 1 out]
          }
          frame True {
          }
        }
        n1272 = local write "Save Plot as jpg"(FALSE ("Save All data")) -> ()
        n1273 = case shown="True" w2775 {
          tunnel: w2774 -> [_ w2806]
          tunnel: [w2798 "Save Plot Data"] -> w2763
          tunnel: w2773 -> [_ w2804]
          frame False {
            n1274 = global read "Results_plotter_Global.vi" "New Chs In"() -> (w2803:string[])
            n1275 = Array Size(array=w2803) -> (size(s)=w2802:i32)
            n1276 = Greater Than 0?(x=w2802) -> (x > 0?=w2801:bool)
            n1277 = Select(t="Input calculated values", s=w2801, f="Create Selectors") -> (s? t:f=w2798:string)
          }
          frame True {
            n1278 = local write "Output Filename"(w2806) -> ()
            n1279 = local write "Header"(w2804) -> ()
          }
        }
      }
      frame "Full Res file manipulator" {
        n1280 = local read "Result files to read"() -> (w2816:path[])
        n1281 = local read "Output Filename"() -> (w2814:path)
        n1282 = local read "Mode"() -> (w2815:T4)
        n1283 = local read "Raw DF in Orig Pos?"() -> (w2811:bool)
        n1284 = global read "Results_plotter_Global.vi" "New Values In"() -> (w2808:string[][])
        n1285 = local read "Plotted rows only?"() -> (w2807:bool)
        n1286 = global read "Results_plotter_Global.vi" "New Chs In"() -> (w2809:string[])
        n1287 = stacked-sequence {
          seq-local: [w2821 _ _ _ _] -> [_ w2849 w2884 _ _]
          seq-local: [_ w2848 _ _ _] -> [_ _ w2885 _ _]
          seq-local: [_ w2844 _ _ _] -> [_ _ w2876 _ _]
          seq-local: [_ _ w2874 _ _] -> [_ _ _ w3097 _]
          seq-local: [_ _ w2873 _ _] -> [_ _ _ w3096 _]
          seq-local: [_ _ w2868 _ _] -> [_ _ _ w3093 _]
          tunnel: [_ _ _ w3100 _] -> w2818
          tunnel: w2816 -> [_ _ w2886 _ _]
          tunnel: w2815 -> [_ w2846 w2883 w3098 _]
          tunnel: w2814 -> [_ _ w2882 _ _]
          tunnel: w2807 -> [w2820 _ w2881 _ _]
          tunnel: w2809 -> [_ _ w2880 _ _]
          tunnel: w2813 -> [_ _ w2879 w3094 _]
          tunnel: w2812 -> [_ _ w2878 w3095 _]
          tunnel: w2811 -> [_ _ w2877 _ _]
          tunnel: w2810 -> [_ _ _ w3099 _]
          tunnel: w2808 -> [_ _ w2870 _ _]
          frame #0 {
            n1288 = global read "Results_plotter_Global.vi" "Row Reference"() -> (w2822:i32[][])
            n1289 = case shown="True" w2820 {
              tunnel: w2822 -> [w2824 w2825]
              tunnel: [w2824 w2826] -> w2821
              frame False {
              }
              frame True {
                n1290 = local read "Plotted Series"() -> (w2828:bool[][])
                n1291 = for {
                  tunnel: w2828 -> [w2835]
                  shift-right: [w2829] -> w2826
                  shift-left: i32[][] [] -> [w2831]
                  tunnel: w2825 -> [w2830] mode=indexing
                  i -> [w2834]
                  n1292 = Index Array(array=w2835, index (col)=w2834) -> (element=w2833:bool[])  [unwired: 1 in]
                  n1293 = Or Array Elements(Boolean array=w2833) -> (logical OR=w2832:bool)
                  n1294 = case shown="True" w2832 {
                    tunnel: w2831 -> [w2836 w2839]
                    tunnel: w2830 -> [_ w2838]
                    tunnel: [w2836 w2837] -> w2829
                    frame False {
                    }
                    frame True {
                      n1295 = Build Array (concatenate)(w2839, w2838) -> (w2837:i32[][])
                    }
                  }
                }
              }
            }
            n1296 = local write "Delete Plotted data from file"(FALSE ("Save All data")) -> ()
          }
          frame #1 {
            n1297 = local read "Job Directory"() -> (w2845:path)
            n1298 = case shown="\"Delete unwanted rows\", Default" w2846 {
              tunnel: [FALSE w2862] -> w2847
              tunnel: [w2858 w2860] -> w2844
              tunnel: w2845 -> [w2858 w2861]
              tunnel: [w2858 w2860] -> w2843
              frame "Post Process Plotted Rows" {
              }
              frame "Delete unwanted rows", Default {
                n1299 = call "Remote_call_prep.vi"("Job Directory In"=w2861) -> ("Job Directory out"=w2860:path)  [unwired: 2 in, 2 out]
                n1300 = local write "Job Directory"(w2860) -> ()
                n1301 = Not Equal?(x=w2861, y=w2860) -> (x != y?=w2862:bool)
              }
            }
            n1302 = Index Array(array=w2849, index (col)=0 ("disabled index (col)")) -> (element=w2841:i32[])  [unwired: 1 in]
            n1303 = for {
              shift-right: [w2851] -> w2848
              shift-left: i32[] [] -> [w2852]
              tunnel: w2841 -> [w2850] mode=indexing
              n1304 = Search 1D Array(1D array=w2852, element=w2850) -> (index of element=w2853:i32)  [unwired: 1 out]
              n1305 = case shown="-1" w2853 {
                tunnel: w2852 -> [w2854 w2857]
                tunnel: [w2854 w2856] -> w2851
                tunnel: w2850 -> [_ w2855]
                frame 0, Default {
                }
                frame -1 {
                  n1306 = Build Array (concatenate)(w2857, w2855) -> (w2856:i32[])
                }
              }
            }
            n1307 = case shown="True" w2847 {
              tunnel: w2843 -> [_ w2864]
              frame False {
              }
              frame True {
                n1308 = local read "Template"() -> (w2863:path)
                n1309 = Path To String(path=w2864) -> (string=w2867:string)
                n1310 = call "Read_Write_Template.vi"("Template File"=w2863, "Mode"=Global_mode."Write Global to File", "Single Value In"=w2867, "Data type"="Log Folder Name" ("Variable name")) -> ()  [unwired: 4 in, 8 out]
              }
            }
          }
          frame #2 {
            w2872 = path[] []
            n1311 = local read "Full_Res_Results_Folder"() -> (w2871:path)
            n1312 = for {
              tunnel: w2886 -> [w2908]
              tunnel: w2885 -> [w2905] mode=indexing
              tunnel: w2884 -> [w2906]
              tunnel: w2883 -> [w2904]
              tunnel: w2882 -> [w2903]
              tunnel: w2881 -> [w2902]
              tunnel: w2880 -> [w2901]
              tunnel: w2879 -> [w2900]
              tunnel: w2878 -> [w2899]
              tunnel: w2877 -> [w2898]
              tunnel: w2876 -> [w2897]
              shift-right: [w2896] -> _
              shift-left: FALSE -> [w2895]
              shift-right: [w2893] -> w2874
              shift-left: w2872 -> [w2894]
              shift-right: [w2891] -> w2873
              shift-left: w2872 -> [w2892]
              tunnel: w2871 -> [w2890]
              tunnel: w2870 -> [w2889]
              shift-right: [w2887] -> w2868
              shift-left: i32[] [] -> [w2888]
              # "Row No in file"
              # "Row No in plotter"
              n1313 = Index Array(array=w2908, index=w2905) -> (element=w2907:path)
              n1314 = stacked-sequence {
                seq-local: [w2913 _ _ _] -> [_ w2949 w2998 _]
                seq-local: [_ w2947 _ _] -> [_ _ w2997 _]
                seq-local: [w2909 _ _ _] -> [_ _ w2990 w3091]
                tunnel: w2907 -> [_ w2948 w2999 _]
                tunnel: w2906 -> [w2923 _ _ _]
                tunnel: w2905 -> [w2916 _ _ _]
                tunnel: w2904 -> [_ w2946 w2996 _]
                tunnel: w2903 -> [_ _ w2995 _]
                tunnel: w2902 -> [_ _ w2994 _]
                tunnel: w2901 -> [_ _ w2993 _]
                tunnel: w2900 -> [_ _ w2992 _]
                tunnel: w2899 -> [_ _ w2991 _]
                tunnel: w2898 -> [_ _ w2989 _]
                tunnel: w2897 -> [_ _ w2988 _]
                tunnel: [_ w2945 _ _] -> w2896
                tunnel: w2895 -> [_ w2944 _ _]
                tunnel: w2894 -> [_ _ w2987 _]
                tunnel: [_ _ w2986 _] -> w2893
                tunnel: w2892 -> [_ _ w2985 _]
                tunnel: [_ _ w2984 _] -> w2891
                tunnel: w2890 -> [_ _ w2983 _]
                tunnel: w2889 -> [_ _ w2982 _]
                tunnel: w2888 -> [_ _ _ w3092]
                tunnel: [_ _ _ w3090] -> w2887
                frame #0 {
                  w2922 = i32[] []
                  # "10/30/13\n#optimation"
                  n1315 = global read "Results_plotter_Global.vi" "Row Reference"() -> (w2921:i32[][])
                  n1316 = local read "Cursor index"() -> (w2920:i32)
                  n1317 = for {
                    tunnel: w2916 -> [w2932]
                    tunnel: w2923 -> [w2928] mode=indexing
                    shift-right: [w2926] -> w2914
                    shift-left: w2922 -> [w2927]
                    shift-right: [w2925] -> w2910
                    shift-left: w2922 -> [w2924]
                    n1318 = Index Array(array=w2928, index=0) -> (element=w2930:i32)
                    n1319 = Equal?(x=w2930, y=w2932) -> (x = y?=w2929:bool)
                    n1320 = case shown="True" w2929 {
                      tunnel: w2928 -> [_ w2936]
                      tunnel: w2927 -> [w2934 w2942]
                      tunnel: [w2934 w2940] -> w2926
                      tunnel: w2924 -> [w2933 w2938]
                      tunnel: [w2933 w2939] -> w2925
                      frame False {
                      }
                      frame True {
                        n1321 = Index Array(array=w2936, index=2) -> (element=w2935:i32)
                        n1322 = Build Array (concatenate)(w2938, w2935) -> (w2939:i32[])
                        n1323 = Index Array(array=w2936, index=1) -> (element=w2941:i32)
                        n1324 = Build Array (concatenate)(w2942, w2941) -> (w2940:i32[])
                      }
                    }
                  }
                  n1325 = Index Array(array=w2921, index (row)=w2920) -> (element=w2918:i32[])  [unwired: 1 in]
                  n1326 = local read "Selected Row?"() -> (w2911:bool)
                  n1327 = Index Array(array=w2918, index #1=0 ("index"), index #2=1 ("index")) -> (element #2=w2915:i32)  [unwired: 1 out]
                  n1328 = Build Array(w2915) -> (w2912:i32[])
                  n1329 = Select(t=w2912, s=w2911, f=w2910) -> (s? t:f=w2909:i32[])
                  n1330 = Select(t=w2912, s=w2911, f=w2914) -> (s? t:f=w2913:i32[])
                }
                frame #1 {
                  n1331 = case shown="\"Edit values per row\"" w2946 {
                    tunnel: w2949 -> [_ _ _ _ _ w2965]
                    tunnel: w2948 -> [_ _ _ _ _ w2963]
                    tunnel: [TRUE ("T button?") TRUE ("T button?") TRUE ("T button?") TRUE ("T button?") TRUE ("T button?") w2962] -> w2947
                    tunnel: [w2950 w2952 w2954 w2956 w2958 w2961] -> w2945
                    tunnel: w2944 -> [w2950 w2952 w2954 w2956 w2958 w2960]
                    frame "Save file" {
                    }
                    frame "Edit values per row" {
                    }
                    frame "Edit Values with constants" {
                    }
                    frame "Edit Raw Data file header" {
                    }
                    frame "Post Process Plotted Rows" {
                    }
                    frame "Delete unwanted rows" {
                      n1332 = Array Size(array=w2965) -> (size(s)=w2964:i32)
                      n1333 = case shown="False" w2960 {
                        tunnel: w2964 -> [w2974 _]
                        tunnel: w2963 -> [w2973 _]
                        tunnel: [w2968 w2981] -> w2962
                        tunnel: [w2967 w2981] -> w2961
                        frame False {
                          n1334 = Format Into String(format string="Remove %d rows from \"%s\"", w2974, w2973) -> (resulting string=w2971:string)  [unwired: 2 in, 1 out]
                          n1335 = call <vilib>:"Three Button Dialog.vi"("Allow user to close window? (TRUE)"=TRUE, "Right Button Text (\"Cancel\")"="Yes To All Files" ("Right Button Text (\"Cancel\")"), "message"=w2971) -> ("Which Button?"=w2969:T11)  [unwired: 3 in, 5 out]
                          n1336 = case shown="\"Left Button\"" w2969 {
                            tunnel: [TRUE TRUE w2979 w2980] -> w2968
                            tunnel: [FALSE TRUE w2979 w2980] -> w2967
                            frame "Left Button" {
                            }
                            frame "Right Button" {
                            }
                            frame "Center Button" {
                              w2979 = FALSE
                            }
                            frame "Window Close" {
                              w2980 = FALSE
                            }
                          }
                        }
                        frame True {
                          w2981 = TRUE
                        }
                      }
                    }
                  }
                }
                frame #2 {
                  n1337 = case shown="True" w2997 {
                    tunnel: w2999 -> [_ w3018]
                    tunnel: w2998 -> [_ w3017]
                    tunnel: w2996 -> [_ w3016]
                    tunnel: w2995 -> [_ w3015]
                    tunnel: w2994 -> [_ w3014]
                    tunnel: w2993 -> [_ w3013]
                    tunnel: w2992 -> [_ w3012]
                    tunnel: w2991 -> [_ w3011]
                    tunnel: w2990 -> [_ w3010]
                    tunnel: w2989 -> [_ w3009]
                    tunnel: w2988 -> [_ w3008]
                    tunnel: w2987 -> [w3001 w3007]
                    tunnel: [w3001 w3006] -> w2986
                    tunnel: w2985 -> [w3000 w3005]
                    tunnel: [w3000 w3004] -> w2984
                    tunnel: w2983 -> [_ w3003]
                    tunnel: w2982 -> [_ w3002]
                    frame False {
                    }
                    frame True {
                      n1338 = case shown="\"Edit Values with constants\"" w3016 {
                        tunnel: w3018 -> [w3024 w3030 w3048 w3061 w3078]
                        tunnel: w3017 -> [w3027 w3037 w3047 w3060 w3077]
                        tunnel: w3015 -> [_ _ _ _ _]
                        tunnel: w3014 -> [_ _ _ w3058 w3075]
                        tunnel: w3013 -> [_ _ _ w3056 w3073]
                        tunnel: w3012 -> [_ _ _ _ w3072]
                        tunnel: w3011 -> [_ _ _ _ w3070]
                        tunnel: w3010 -> [_ _ _ _ w3069]
                        tunnel: w3009 -> [_ _ _ w3055 w3067]
                        tunnel: w3008 -> [_ _ _ w3053 w3065]
                        tunnel: w3007 -> [w3026 w3034 w3046 w3051 w3063]
                        tunnel: [w3026 w3035 w3046 w3051 w3063] -> w3006
                        tunnel: w3005 -> [w3025 w3033 w3045 w3050 w3062]
                        tunnel: [w3025 w3031 w3045 w3050 w3062] -> w3004
                        tunnel: w3003 -> [w3023 _ _ _ _]
                        tunnel: w3002 -> [_ _ _ w3049 _]
                        frame "Save file" {
                          n1339 = Strip Path(path=w3024) -> (name=w3021:string)  [unwired: 1 out]
                          n1340 = call "Add_filename_suffix.vi"("Filename"=w3021, "Suffix to add"=".xls") -> ("Filename out"=w3019:string)  [unwired: 3 out]
                          n1341 = Build Path(base path=w3023, name or relative path=w3019) -> (appended path=w3022:path)
                          n1342 = call "Save_full_Res_rows.vi"("Selected Rows"=w3027, "Filename to write"=w3022, "Filename Orig"=w3024) -> ()  [unwired: 2 out]
                        }
                        frame "Edit Raw Data file header", Default {
                          n1343 = call "GetRawDataFilePaths.vi"("Results file or Folder"=w3030) -> ("RawDataFilePaths"=w3028:string[], "RowNumbers"=w3029:i32[])  [unwired: 9 in]
                          n1344 = for {
                            tunnel: w3028 -> [w3044]
                            tunnel: w3037 -> [w3038] mode=indexing
                            tunnel: [w3042] -> w3036 mode=indexing
                            tunnel: [w3041] -> w3032 mode=indexing
                            tunnel: w3030 -> [w3041]
                            tunnel: w3029 -> [w3040]
                            n1345 = Search 1D Array(1D array=w3040, element=w3038) -> (index of element=w3039:i32)  [unwired: 1 in]
                            n1346 = Index Array(array=w3044, index=w3039) -> (element=w3043:string)
                            n1347 = call "String_to_Pathname.vi"("Input String"=w3043) -> ("path"=w3042:path)
                          }
                          n1348 = Build Array (concatenate)(w3033, w3032) -> (w3031:path[])
                          n1349 = Build Array (concatenate)(w3034, w3036) -> (w3035:path[])
                        }
                        frame "Delete unwanted rows" {
                          n1350 = call "Delete_unwanted_rows.vi"("Selected Rows"=w3047, "Filename"=w3048) -> ()  [unwired: 1 out]
                        }
                        frame "Edit Values with constants" {
                          w3059 = TRUE  # Value  Constant?
                          n1351 = local read "Edit Raw Data Header Info"() -> (w3052:bool)
                          n1352 = local read "Edit Raw DF?"() -> (w3054:bool)
                          n1353 = Not(x=w3058) -> (.not. x?=w3057:bool)
                          n1354 = call "Add_Update_Values.vi"("Filename"=w3061, "Value  Constant?"=w3059, "Edit Raw data files?"=w3054, "New Chs In"=w3056, "Edit Raw Data Header Info"=w3052, "New Values In"=w3049, "Selected Rows"=w3060, "Edit all Rows?"=w3057, "Raw DF in Orig Pos?"=w3055, "Job Directory"=w3053) -> ()  [unwired: 1 in, 5 out]
                        }
                        frame "Edit values per row" {
                          w3064 = FALSE  # Edit Raw Data Header Info
                          w3076 = FALSE  # Value  Constant?
                          n1355 = for {
                            tunnel: w3073 -> [w3089] mode=indexing
                            tunnel: w3072 -> [w3088]
                            tunnel: [w3087] -> w3071 mode=indexing
                            n1356 = Search 1D Array(1D array=w3088, element=w3089) -> (index of element=w3087:i32)  [unwired: 1 out]
                          }
                          n1357 = for {
                            tunnel: w3071 -> [w3083]
                            tunnel: w3070 -> [w3082]
                            tunnel: w3069 -> [w3080] mode=indexing
                            tunnel: [w3079] -> w3068 mode=indexing
                            n1358 = Index Array(array=w3082, index (row)=w3080) -> (element=w3081:string[])  [unwired: 1 in]
                            n1359 = for {
                              tunnel: w3083 -> [w3086] mode=indexing
                              tunnel: w3081 -> [w3085]
                              tunnel: [w3084] -> w3079 mode=indexing
                              n1360 = Index Array(array=w3085, index=w3086) -> (element=w3084:string)
                            }
                          }
                          n1361 = Not(x=w3075) -> (.not. x?=w3074:bool)
                          n1362 = local read "Edit Raw DF?"() -> (w3066:bool)
                          n1363 = call "Add_Update_Values.vi"("Filename"=w3078, "Value  Constant?"=w3076, "Edit Raw data files?"=w3066, "New Chs In"=w3073, "Edit Raw Data Header Info"=w3064, "New Values In"=w3068, "Selected Rows"=w3077, "Edit all Rows?"=w3074, "Raw DF in Orig Pos?"=w3067, "Job Directory"=w3065) -> ()  [unwired: 1 in, 5 out]
                        }
                      }
                    }
                  }
                }
                frame #3 {
                  n1364 = Build Array (concatenate)(w3092, w3091) -> (w3090:i32[])
                }
              }
            }
          }
          frame #3 {
            n1365 = case shown="\"Edit Raw Data file header\"" w3098 {
              tunnel: ["Create Selectors" w3108 "Initialise" ("t") w3167] -> w3100
              tunnel: w3099 -> [_ _ _ w3164]
              tunnel: w3097 -> [w3101 w3107 _ _]
              tunnel: w3096 -> [_ w3106 _ _]
              tunnel: w3095 -> [_ w3105 _ _]
              tunnel: w3094 -> [_ w3104 _ _]
              tunnel: w3093 -> [_ w3103 _ _]
              frame "Edit Raw Data file header" {
                n1366 = call "Edit_Raw_DF_Header.vi"("Selected files"=w3101) -> ()  [unwired: 15 out]
              }
              frame "Post Process Plotted Rows" {
                n1367 = stacked-sequence {
                  seq-local: [w3110 _ _] -> [_ w3134 _]
                  seq-local: [w3109 _ _] -> [_ _ w3159]
                  seq-local: [_ w3131 _] -> [_ _ w3158]
                  tunnel: [_ _ "Create Selectors"] -> w3108
                  tunnel: w3107 -> [_ _ w3161]
                  tunnel: w3106 -> [_ _ w3160]
                  tunnel: w3105 -> [_ w3133 _]
                  tunnel: w3104 -> [w3111 _ _]
                  tunnel: w3103 -> [_ w3130 _]
                  frame #0 {
                    n1368 = global read "Results_plotter_Global.vi" "Dispose"() -> (w3113:string[])
                    n1369 = for {
                      tunnel: w3113 -> [w3122] mode=indexing
                      shift-right: [w3118] -> w3110
                      shift-left: i32[] [] -> [w3120]
                      i -> [w3119]
                      n1370 = String Subset(string=w3122, length (rest)=1 ("length (rest)")) -> (substring=w3124:string)  [unwired: 1 out]
                      n1371 = Equal?(x="T", y=w3124) -> (x = y?=w3121:bool)
                      n1372 = case shown="False" w3121 {
                        tunnel: w3120 -> [w3128 w3129]
                        tunnel: [w3127 w3129] -> w3118
                        tunnel: w3119 -> [w3126 _]
                        frame False {
                          n1373 = Build Array (concatenate)(w3128, w3126) -> (w3127:i32[])
                        }
                        frame True {
                        }
                      }
                    }
                    n1374 = for {
                      tunnel: w3111 -> [w3117]
                      tunnel: w3110 -> [w3116] mode=indexing
                      tunnel: [w3115] -> w3109 mode=indexing
                      n1375 = Index Array(array=w3117, index=w3116) -> (element=w3115:string)
                    }
                    n1376 = local write "Post Process Plotted Data"(FALSE ("Post Process Plotted Data")) -> ()
                  }
                  frame #1 {
                    n1377 = global read "Results_plotter_Global.vi" "Precision"() -> (w3132:string[])
                    n1378 = for {
                      tunnel: w3134 -> [w3140]
                      tunnel: w3133 -> [w3136]
                      tunnel: w3132 -> [w3139]
                      tunnel: [w3138] -> w3131 mode=indexing
                      tunnel: w3130 -> [w3137] mode=indexing
                      n1379 = Index Array(array=w3136, index (row)=w3137) -> (element=w3135:string[])  [unwired: 1 in]
                      n1380 = for {
                        tunnel: w3140 -> [w3150] mode=indexing
                        tunnel: w3135 -> [w3152]
                        tunnel: w3139 -> [w3151]
                        tunnel: [w3144] -> w3138 mode=indexing
                        n1381 = Index Array(array=w3152, index=w3150) -> (element=w3143:string)
                        n1382 = Index Array(array=w3151, index=w3150) -> (element=w3142:string)
                        n1383 = Fract/Exp String To Number(string=w3143) -> (offset past number=w3148:i32, number=w3145:dbl)  [unwired: 3 out]
                        n1384 = String Length(string=w3143) -> (length=w3149:i32)
                        n1385 = Equal?(x=w3149, y=w3148) -> (x = y?=w3146:bool)
                        n1386 = Empty String/Path?(string/path=w3143) -> (empty?=w3147:bool)
                        n1387 = Compound Arithmetic op=AND(invert w3147, w3146) -> (w3141:bool)
                        n1388 = case shown="True" w3141 {
                          tunnel: w3142 -> [_ w3155]
                          tunnel: w3145 -> [_ w3156]
                          tunnel: [w3153 w3154] -> w3144
                          tunnel: w3143 -> [w3153 _]
                          frame False {
                          }
                          frame True {
                            n1389 = call "Number_2_string.vi"("precision"=w3155, "number"=w3156) -> ("String"=w3154:string)
                          }
                        }
                      }
                    }
                  }
                  frame #2 {
                    n1390 = Build Array (concatenate)(w3159, w3158) -> (w3157:string[][])
                    n1391 = call "Post_Process_Profile_Remote.vi"("Results Plotter Rows"=w3157, "Raw Data files to PP"=w3161, "Current Results filenames"=w3160) -> ()  [unwired: 1 out]
                  }
                }
              }
              frame "Delete unwanted rows" {
              }
              frame "Edit Values with constants", Default {
                n1392 = local read "nRows"() -> (w3166:i32)
                n1393 = Less?(x=w3166, y=w3164) -> (x < y?=w3165:bool)
                n1394 = case shown="True" w3165 {
                  tunnel: ["Create Selectors" "Initialise" ("t")] -> w3167
                  frame False {
                  }
                  frame True {
                  }
                }
              }
            }
          }
          frame #4 {
            n1395 = Current VI's Path() -> (path=w3170:path)
            n1396 = call "Bring_to_front.vi"("path"=w3170) -> ()
          }
        }
      }
      frame "End" {
        n1397 = local read "Template"() -> (w3172:path)
        n1398 = local read "Empty"() -> (w3173:bool)
        n1399 = call "Valid_Path.vi"("Filename"=w3172) -> ("Valid Path?"=w3171:bool)
        n1400 = case shown="True" w3173 {
          frame False {
          }
          frame True {
            n1401 = property on="Result files to read" class="Arr (strict)"("Index Values"=u32[] [0] ("Write Attribute")) -> ()  [unwired: 2 in, 2 out]
            n1402 = local write "Result files to read"(path[] [] ("Result files to read")) -> ()
            n1403 = local write "Empty"(FALSE ("Empty")) -> ()
          }
        }
        n1404 = case shown="False" w3171 {
          tunnel: w3174 -> [w3183 _]
          frame False {
            n1405 = local write "Template"(w3183) -> ()
          }
          frame True {
          }
        }
      }
      frame "Empty Results file array" {
        n1406 = local read "Template"() -> (w3185:path)
        n1407 = call "Valid_Path.vi"("Filename"=w3185) -> ("Valid Path?"=w3184:bool)
        n1408 = case shown="True" w3184 {
          tunnel: w3186 -> [w3195 _]
          frame False {
            n1409 = local write "Template"(w3195) -> ()
          }
          frame True {
          }
        }
        n1410 = property on="Result files to read" class="Arr (strict)"("Index Values"=u32[] [0] ("Write Attribute")) -> ()  [unwired: 2 in, 2 out]
        n1411 = local write "Result files to read"(path[] [] ("Result files to read")) -> ()
        n1412 = local write "Empty"(FALSE ("Empty")) -> ()
      }
      frame "Save Setup" {
        w3200 = "Current_Setup.xls" ("Setup filename")
        n1413 = local read "Create picture Vi Name"() -> (w3215:string)
        n1414 = local read "Result files to read"() -> (w3223:path[])
        n1415 = local read "Additional X Values"() -> (w3221:dbl[])
        n1416 = local read "Additional Y Values"() -> (w3220:dbl[])
        n1417 = local read "Output Filename"() -> (w3216:path)
        n1418 = local read "Intensity Plot?"() -> (w3214:bool)
        n1419 = local read "Multi Ordinate?"() -> (w3213:bool)
        n1420 = local read "Multi Ordinate"() -> (w3209:i32[])
        n1421 = local read "Filter Array"() -> (w3217:u16[])
        n1422 = local read "Transpose"() -> (w3222:bool)
        n1423 = local read "Template"() -> (w3201:path)
        n1424 = local read "Ordinate"() -> (w3219:u16)
        n1425 = local read "Filter Bins 2"() -> (w3210:i32[])
        n1426 = local read "Filter Bins 1"() -> (w3211:i32[])
        n1427 = local read "Absisca"() -> (w3218:u16)
        n1428 = call "Read_Write_Plot_Setup.vi"("Mode"=enum16{"Load", "Save"}."Load", "Setup filename"=w3200) -> ("Cluster 2"=w3224:T10)  [unwired: 1 in, 1 out]
        n1429 = Bundle By Name(cluster=w3224, "Result files to read"=w3223, "Template"=w3201, "Transpose"=w3222, "Additional X Values"=w3221, "Additional Y Values"=w3220, "Ordinate"=w3219, "Absisca"=w3218, "Filter Array"=w3217, "color and symbol"=TRUE, "Output Filename"=w3216, "Jpg Vi Name"=w3215, "Intensity Plot?"=w3214, "Multi Ordinate?"=w3213, "Filter Bins 1"=w3211, "Filter Bins 2"=w3210, "Multi Ordinate"=w3209) -> (w3212:T10)
        n1430 = local read "Save Setup"() -> (w3199:bool)
        n1431 = local read "stop"() -> (w3207:bool)
        n1432 = Not(x=w3207) -> (.not. x?=w3206:bool)
        n1433 = Path To String(path="Job Directory") -> (string=w3205:string)
        n1434 = call "Read_Write_Plot_Setup.vi"("Mode"=enum16{"Load", "Save"}."Save", "Setup filename"=w3200, "Cluster"=w3212) -> ()  [unwired: 2 out]
        n1435 = call "Read_Write_Template.vi"("Template File"=w3201, "Mode"=Global_mode."Write Global to File", "Single Value In"=w3205, "Data type"="Log Folder Name" ("Variable name")) -> ()  [unwired: 4 in, 8 out]
        n1436 = Select(t="Save to named setup file", s=w3199, f="Check modification dates?") -> (s? t:f=w3197:string)
      }
      frame "Save to named setup file" {
        w3231 = TRUE  # Save New File?
        n1437 = call "Save_current_setup.vi"("Save New File?"=w3231, "Setup File Type"=Setup_Filetype."Results File Plotter Setups") -> ()  [unwired: 4 out]
        n1438 = local write "Save Setup"(FALSE ("Save Setup")) -> ()
      }
    }
    "Current" <- w11
  }
